vi "WVDIAL+HSRL_v5.1.vi"() -> ()   [LabVIEW 2012]
uses:
  C:/Users/H2ODial/Desktop/Shared Telescope WV DIAL Code/Libraries and VIs/PowerMeterCommands.dll
  Shared Telescope WV DIAL Code/Libraries and VIs/PowerMeterCommands.dll
  <vilib>/DAQmx/write.llb/DAQmx Write (Digital 1D Bool NChan 1Samp 1Line).vi
  <vilib>/DAQmx/miscellaneous.llb/DAQmx Fill In Error Info.vi
  <vilib>/Analysis/baseanly.llb/Mean (DBL).vi
  NCAR_DIAL_Labview/AMCS_Data.vi
  Shared Telescope WV DIAL Code/Libraries and VIs/Scalar_Data.vi
  <vilib>/Analysis/NI_AALBase.lvlib
  Shared Telescope WV DIAL Code/Libraries and VIs/Scalar_Data_2.vi
  Shared Telescope WV DIAL Code/Libraries and VIs/Scalar_Data_4.vi
  Shared Telescope WV DIAL Code/Libraries and VIs/Scalar_Data_3.vi
  Shared Telescope WV DIAL Code/bristol/CLDevIFace.dll
panel:
  out "sigma_off_total":dbl[](array[numeric])=[4.801394588286161e-25, 4.768950050217253e-25, 4.736689753639405e-25, 4.704613337303019e-25, 4.672720432926519e-25, 4.641010665257011e-25, 4.609483652155645e-25, 4.578139004644591e-25, 4.546976326993031e-25, 4.515995216769696e-25, 4.485195264899329e-25, 4.454576055746445e-25, 4.424137167181121e-25, 4.393878170609112e-25, 4.36379863107592e-25, 4.33389810729471e-25, 4.304176151739443e-25, 4.274632310672864e-25, 4.245266124220741e-25, 4.216077126439569e-25, 4.1870648453569715e-25, 4.158228803020544e-25, 4.1295685155887294e-25, 4.101083493348861e-25, 4.0727732407759397e-25, 4.044637256610407e-25, 4.016675033855836e-25, 3.9888860598986357e-25, 3.961269816478675e-25, 3.933825779804876e-25, 3.9065534205464125e-25, 3.879452203900322e-25, 3.852521589644783e-25, 3.8257610321550862e-25, 3.7991699804548973e-25, 3.772747878252632e-25, 3.7464941639826676e-25, 3.7204082708226036e-25, 3.6944896267636864e-25, 3.6687376545860182e-25, 3.643151771951297e-25, 3.617731391374568e-25, 3.592475920295502e-25, 3.5673847610815624e-25, 3.5424573110509713e-25, 3.51769296250307e-25, 3.4930911027336777e-25, 3.4686511140682367e-25, 3.4443723738419093e-25, 3.420254254472963e-25, 3.396296123410816e-25, 3.3724973432070024e-25, 3.348857271482379e-25, 3.3253752609613435e-25, 3.302050659473697e-25, 3.278882809942613e-25, 3.2558710504094295e-25, 3.2330147140280016e-25, 3.2103131290665886e-25, 3.1877656188850774e-25, 3.1653715019639748e-25, 3.1431300918716313e-25, 3.1210406972649136e-25, 3.099102621887104e-25, 3.077315164535497e-25, 3.055677619063733e-25, 3.0341892743640323e-25, 3.0128494143392254e-25, 2.9916573178829195e-25, 2.9706122588715016e-25, 2.949713506116264e-25, 2.928960323357407e-25, 2.9083519692181943e-25, 2.8878876971857424e-25, 2.8675667555590972e-25, 2.8473883874352263e-25, 2.82735183065705e-25, 2.807456317775674e-25, 2.78770107600355e-25, 2.768085327176829e-25, 2.7486082876930466e-25, 2.7292691684857373e-25, 2.710067174953994e-25, 2.69100150690391e-25, 2.6720713585077757e-25, 2.6532759182425502e-25, 2.6346143688111433e-25, 2.616085887119142e-25, 2.5976896441660036e-25, 2.5794248050002976e-25, 2.5612905286688828e-25, 2.543285968121087e-25, 2.5254102701448346e-25, 2.5076625753044143e-25, 2.4900420178674013e-25, 2.472547725712684e-25, 2.455178820294026e-25, 2.437934416518099e-25, 2.4208136227195425e-25, 2.4038155405432917e-25, 2.386939264904309e-25, 2.3701838838914442e-25, 2.3535484787249933e-25, 2.3370321236430464e-25, 2.320633885866848e-25, 2.304352825543552e-25, 2.288187995634922e-25, 2.2721384419102023e-25, 2.256203202865053e-25, 2.2403813096701963e-25, 2.224671786131482e-25, 2.2090736486310434e-25, 2.1935859061206393e-25, 2.1782075600723924e-25, 2.162937604472023e-25, 2.147775025765241e-25, 2.1327188029253344e-25, 2.1177679073943044e-25, 2.1029213031283628e-25, 2.088177946592786e-25, 2.073536786873868e-25, 2.058996765626047e-25, 2.044556817235209e-25, 2.0302158688396276e-25, 2.015972840423812e-25, 2.0018266449704104e-25, 1.9877761885463494e-25, 1.973820370468632e-25, 1.9599580834763557e-25, 1.9461882138944004e-25, 1.9325096418746903e-25, 1.918921241569432e-25, 1.905421881443037e-25, 1.892010424507014e-25, 1.8786857286323568e-25, 1.8654466468810693e-25, 1.8522920278453332e-25, 1.8392207160043708e-25, 1.826231552176911e-25, 1.813323373944262e-25, 1.800495016075253e-25, 1.7877453110235048e-25, 1.7750730895249978e-25, 1.7624771810553433e-25, 1.7499564144345078e-25, 1.7375096184837848e-25, 1.7251356226542884e-25, 1.7128332576430962e-25, 1.700601356212511e-25, 1.6884387538163331e-25, 1.6763442894316712e-25, 1.6643168063629809e-25, 1.6523551530533992e-25, 1.6404581839097108e-25, 1.6286247602390061e-25, 1.6168537512090233e-25, 1.605144034614135e-25, 1.5934944980685089e-25, 1.5819040397930432e-25, 1.5703715697926553e-25, 1.5588960107181738e-25, 1.5474762991142214e-25, 1.5361113863299152e-25, 1.5248002396306513e-25, 1.5135418433697008e-25, 1.50233520001562e-25, 1.4911793312712513e-25, 1.480073279180435e-25, 1.4690161073176908e-25, 1.4580069018064647e-25, 1.447044772476486e-25, 1.4361288539606514e-25, 1.4252583067416848e-25, 1.4144323182887283e-25, 1.4036501040910553e-25, 1.3929109086478254e-25, 1.3822140065101003e-25, 1.3715587032647203e-25, 1.3609443364486227e-25, 1.3503702764541747e-25, 1.3398359274152155e-25, 1.329340728030297e-25, 1.3188841522272228e-25, 1.3084657100845003e-25, 1.2980849483220153e-25, 1.2877414509217843e-25, 1.2774348397529735e-25, 1.2671647750218706e-25, 1.2569309555783823e-25, 1.2467331194344784e-25, 1.2365710438524509e-25, 1.226444545632135e-25, 1.2163534812596623e-25, 1.2062977468041493e-25, 1.196277278032819e-25, 1.1862920501492717e-25, 1.1763420776665477e-25, 1.1664274140569122e-25, 1.1565481514090832e-25, 1.146704420038681e-25, 1.136896387746299e-25, 1.1271242593980075e-25, 1.1173882761421185e-25, 1.107688714604918e-25, 1.0980258860269755e-25, 1.0884001353764384e-25, 1.078811840315363e-25, 1.0692614100744287e-25, 1.0597492844191873e-25, 1.050275932281712e-25, 1.040841850623073e-25, 1.0314475630412393e-25, 1.0220936184080334e-25, 1.0127805894236583e-25, 1.0035090711634834e-25, 9.942796795457985e-26, 9.85093049826673e-26, 9.759498349455631e-26, 9.668507040548591e-26, 9.577963407225883e-26, 9.487874414542166e-26, 9.398247139650076e-26, 9.309088755804386e-26, 9.220406515296338e-26, 9.132207733747452e-26, 9.044499773262688e-26, 8.957290026345629e-26, 8.870585900482974e-26, 8.784394801646169e-26, 8.698724119587757e-26, 8.613581212497107e-26, 8.528973392272335e-26, 8.444907910479177e-26, 8.361391944296957e-26, 8.278432583478717e-26, 8.196036817304802e-26, 8.114211522534205e-26, 8.032963451681958e-26, 7.952299221933221e-26, 7.872225304713498e-26, 7.792748015992029e-26, 7.713873506910441e-26, 7.635607755587433e-26, 7.557956559150637e-26, 7.480925526823318e-26, 7.40452007331766e-26, 7.328745413088994e-26, 7.253606555846716e-26, 7.179108301816113e-26, 7.105255237909276e-26, 7.032051735602558e-26, 6.959501948332896e-26, 6.887609809279164e-26, 6.816379032159524e-26, 6.745813109633723e-26, 6.675915313529315e-26, 6.606688697494169e-26, 6.538136097430423e-26, 6.47026013369233e-26, 6.403063215180626e-26, 6.336547541226546e-26, 6.270715106859048e-26, 6.20556770626669e-26, 6.141106938516726e-26, 6.077334213535519e-26, 6.014250756428306e-26, 5.951857615555011e-26, 5.890155669044941e-26, 5.829145630606328e-26, 5.768828060635133e-26, 5.709203369799531e-26, 5.650271830406457e-26, 5.592033586495535e-26, 5.534488657823541e-26, 5.477636955007899e-26, 5.421478286457689e-26, 5.366012367016147e-26, 5.311238832156924e-26, 5.257157245373203e-26, 5.203767111080975e-26, 5.151067883628761e-26, 5.099058981646601e-26, 5.047739796747887e-26, 4.99710970692362e-26, 4.9471680904655766e-26, 4.897914334302848e-26, 4.8493478509221053e-26, 4.8014680897944407e-26, 4.754274547829409e-26, 4.707766789526016e-26, 4.661944455372514e-26, 4.616807276932442e-26, 4.5723550945439755e-26, 4.52858787046509e-26, 4.485505703210599e-26, 4.443108844474691e-26, 4.401397715518555e-26, 4.360372926484654e-26, 4.320035290481737e-26, 4.2803858415410786e-26, 4.2414258571215696e-26, 4.2031568752669364e-26, 4.1655807122192707e-26, 4.1286994901985047e-26, 4.0925156557589725e-26, 4.057032001511829e-26, 4.022251691740667e-26, 3.988178290967981e-26, 3.954815788073776e-26, 3.9221686230680586e-26, 3.8902417233706774e-26, 3.859040524446151e-26, 3.828571019686779e-26, 3.7988397781509877e-26, 3.769854001153642e-26, 3.7416215439626103e-26, 3.7141509747308686e-26, 3.687451613900974e-26, 3.6615335855838153e-26, 3.63640786278229e-26, 3.612086341870923e-26, 3.5885818841799324e-26, 3.5659083977640876e-26, 3.544080898134836e-26, 3.5231155864237455e-26, 3.5030299361038637e-26, 3.4838427775418294e-26, 3.465574396234356e-26, 3.4482466342706975e-26, 3.4318830100156596e-26, 3.4165088275400604e-26, 3.402151318089598e-26, 3.388839783242867e-26, 3.3766057389929274e-26, 3.36548309398701e-26, 3.3555083377338027e-26, 3.346720715137672e-26, 3.3391624601031894e-26, 3.3328790250155764e-26, 3.3279193257884915e-26, 3.324336013175799e-26, 3.322185772847288e-26, 3.3215296392257455e-26, 3.3224333404110883e-26, 3.3249676503872935e-26, 3.329208802997051e-26, 3.335238896228958e-26, 3.343146339557761e-26, 3.353026321412742e-26, 3.364981297192093e-26, 3.379121497286846e-26, 3.395565434610739e-26, 3.414440403258726e-26, 3.4358829907497297e-26, 3.460039513028062e-26, 3.487066380487166e-26, 3.51713038203815e-26, 3.55040877164833e-26, 3.587089122589996e-26, 3.6273688416960675e-26, 3.6714542267064066e-26, 3.7195588478670957e-26, 3.7719011171675543e-26, 3.8287006590553707e-26, 3.890173237259351e-26, 3.95652358320561e-26, 4.02793573539223e-26, 4.1045600378726224e-26, 4.186495854869218e-26, 4.2737690452423645e-26, 4.3663028300744097e-26, 4.4638807992990383e-26, 4.5661005992560553e-26, 4.6723172620936825e-26, 4.781575526222953e-26, 4.8925318931385875e-26, 5.0033690286108284e-26, 5.1117084461502723e-26, 5.214532077700266e-26, 5.308129043822377e-26, 5.388090789277132e-26, 5.44938332756638e-26, 5.486527227774992e-26, 5.493910002738325e-26, 5.466237631938079e-26, 5.399100135383679e-26, 5.289584428918705e-26, 5.1368276864546713e-26, 4.9423845443889993e-26, 4.710298039802831e-26, 4.446823095455392e-26, 4.1598358649719716e-26, 3.85804282785832e-26, 3.5501475783679474e-26, 3.2441260709634926e-26, 2.946712395982361e-26, 2.6631308337930007e-26, 2.3970517538376977e-26, 2.150714060589855e-26, 1.9251465674211592e-26, 1.720428679383541e-26, 1.53594676712807e-26, 1.3706206451822994e-26, 1.2230884236655608e-26, 1.0918482976983566e-26, 9.753612237371755e-27, 8.721210233721729e-27, 7.806991018507e-27, 6.997701798420481e-27, 6.2812456801226914e-27, 5.646712358776296e-27, 5.084349444566265e-27, 4.5854974957865986e-27, 4.142505607433107e-27, 3.748638403172051e-27, 3.397981811656704e-27, 3.085352100165531e-27, 2.8062108305879284e-27, 2.5565869422707086e-27, 2.3330065259403903e-27, 2.1324302344192426e-27, 1.9521978729601313e-27, 1.789979757382958e-27, 1.643734082137034e-27, 1.5116697902511733e-27, 1.3922142210516644e-27, 1.2839850124507306e-27, 1.1857657103866845e-27, 1.096484610302639e-27, 1.015196395714895e-27, 9.410662182426697e-28, 8.733558712047939e-28, 8.114117898619021e-28, 7.546546232319497e-28, 7.025701642912456e-28, 6.547014513806149e-28, 6.106418931238552e-28, 5.700292622253593e-28, 5.325404588349162e-28, 4.9788692660923625e-28, 4.658106430581142e-28, 4.360806068197592e-28, 4.08489753956538e-28, 3.828522501146923e-28, 3.5900111064396606e-28, 3.3678610372110053e-28, 3.1607190332545146e-28, 2.967364589362001e-28, 2.7866955609085765e-28, 2.617715425159856e-28, 2.459522015206387e-28, 2.31129753123374e-28, 2.1722996779390465e-28, 2.041853801540389e-28, 1.9193458968197297e-28, 1.8042163895501554e-28, 1.6959545965331195e-28, 1.5940937941231567e-28, 1.498206814409963e-28, 1.4079021188262282e-28, 1.322820287603016e-28, 1.2426308841814503e-28, 1.1670296471282332e-28, 1.095735979222345e-28, 1.028490696002857e-28, 9.650540091750711e-29, 9.052037168469339e-29, 8.487335801198675e-29, 7.954518653327039e-29, 7.451800341677787e-29, 6.977515667544699e-29, 6.530109029807567e-29, 6.108124904915991e-29, 5.710199275226091e-29, 5.335051912802774e-29, 4.981479429414531e-29, 4.6483490131613607e-29, 4.334592782554835e-29, 4.039202695474115e-29, 3.7612259553878387e-29, 3.4997608663220985e-29, 3.253953089846661e-29, 3.0229922636158786e-29, 2.806108945951869e-29, 2.602571852405365e-29, 2.41168535589881e-29, 2.2327872228526563e-29, 2.065246562048159e-29, 1.9084619645126237e-29, 1.761859814754614e-29, 1.624892755927198e-29, 1.4970382931010645e-29, 1.3777975202772093e-29, 1.2666939582553547e-29, 1.1632724915852204e-29, 1.0670983941271466e-29, 9.777564337076934e-30, 8.948500471556312e-30, 8.180005779879964e-30, 7.468465697390879e-30, 6.810431085231261e-30, 6.202612091610602e-30, 5.641872396741644e-30, 5.12522379523866e-30, 4.6498210741493256e-30, 4.2129571491792276e-30, 3.812058425696018e-30, 3.444680354488451e-30, 3.108503155773409e-30, 2.8013276878747435e-30, 2.5210714397788027e-30, 2.2657646294144864e-30, 2.033546391805329e-30, 1.8226610435053844e-30, 1.6314544116870018e-30, 1.4583702181671436e-30, 1.301946510394041e-30, 1.160812132981031e-30, 1.0336832348936875e-30, 9.19359808752369e-31, 8.167222599729037e-31, 7.247280046352818e-31, 6.42408096031317e-31, 5.688638808252746e-31, 5.032636866339413e-31, 4.448395436382558e-31, 3.928839435526092e-31, 3.4674663990238277e-31, 3.058314941188273e-31, 2.6959337244037458e-31, 2.3753509904461953e-31, 2.0920447127862125e-31, 1.8419134350394772e-31, 1.6212478764982733e-31, 1.4267034433980083e-31, 1.255274084032685e-31, 1.1042704425817586e-31, 9.713732882503646e-32, 8.542234365126433e-32, 7.509010926979831e-32, 6.599724118567433e-32, 5.798258327626743e-32, 5.0914513032109e-32, 4.4677742840358584e-32, 3.9171311676341143e-32, 3.430696615097442e-32, 3.000769114943473e-32, 2.620636555271221e-32, 2.2844537200985846e-32, 1.9871313368209626e-32, 1.724236277148701e-32, 1.491902447124409e-32, 1.2867518305554977e-32, 1.1058250844486695e-32, 9.465210287068717e-33]
  out "sigma_on_total":dbl[](array[numeric])=[1.4915279728419454e-23, 1.4842365731966544e-23, 1.4769019163032043e-23, 1.4695253757788467e-23, 1.462108321716903e-23, 1.4546521199986097e-23, 1.447158131870194e-23, 1.439627713335683e-23, 1.432062214702501e-23, 1.4244629800835914e-23, 1.416831346884805e-23, 1.4091686453334493e-23, 1.401476198047694e-23, 1.3937553195090692e-23, 1.3860073157963141e-23, 1.378233483947944e-23, 1.370435111777655e-23, 1.3626134773198228e-23, 1.3547698485081338e-23, 1.3469054828400842e-23, 1.3390216270010062e-23, 1.3311195164756476e-23, 1.3232003753881505e-23, 1.315265415980152e-23, 1.3073158384514339e-23, 1.2993528307058406e-23, 1.2913775679522576e-23, 1.2833912126101407e-23, 1.2753949138594952e-23, 1.2673898077025441e-23, 1.2593770164365874e-23, 1.2513576486882712e-23, 1.2433327991214158e-23, 1.2353035482876853e-23, 1.2272709624381212e-23, 1.2192360933728872e-23, 1.2111999783785617e-23, 1.2031636399495558e-23, 1.1951280858745917e-23, 1.1870943088820745e-23, 1.179063286847115e-23, 1.1710359823865174e-23, 1.1630133430362646e-23, 1.1549963011158184e-23, 1.1469857736050211e-23, 1.1389826621774752e-23, 1.1309878531936014e-23, 1.1230022176071374e-23, 1.1150266109305435e-23, 1.1070618733984849e-23, 1.0991088297833858e-23, 1.0911682894818458e-23, 1.0832410465605054e-23, 1.075327879786099e-23, 1.0674295526174507e-23, 1.0595468132519867e-23, 1.0516803947245639e-23, 1.0438310149891488e-23, 1.0359993768724897e-23, 1.028186168237809e-23, 1.0203920620632735e-23, 1.0126177164388007e-23, 1.004863774789339e-23, 9.971308658609087e-24, 9.894196038876879e-24, 9.817305886336727e-24, 9.740644055897453e-24, 9.66421625982583e-24, 9.588028070218673e-24, 9.512084918974381e-24, 9.436392099708197e-24, 9.360954769268839e-24, 9.285777948467669e-24, 9.210866524075807e-24, 9.136225249623787e-24, 9.061858747248887e-24, 8.987771509156659e-24, 8.913967899106149e-24, 8.840452153334211e-24, 8.767228383070224e-24, 8.694300575302228e-24, 8.621672594735212e-24, 8.54934818499285e-24, 8.477330970786176e-24, 8.405624458768497e-24, 8.334232040093874e-24, 8.26315699129617e-24, 8.19240247593568e-24, 8.121971546612565e-24, 8.051867146610725e-24, 7.982092111191124e-24, 7.91264916943216e-24, 7.8435409460626e-24, 7.774769962767551e-24, 7.706338640024972e-24, 7.638249298761754e-24, 7.570504162344009e-24, 7.503105357207897e-24, 7.436054915859422e-24, 7.369354777003414e-24, 7.303006789004784e-24, 7.237012709367644e-24, 7.171374208324226e-24, 7.106092869293601e-24, 7.041170190650204e-24, 6.97660758762949e-24, 6.912406393431767e-24, 6.848567861106454e-24, 6.785093165255731e-24, 6.721983403264505e-24, 6.659239596832755e-24, 6.596862693493495e-24, 6.534853568410539e-24, 6.473213025417807e-24, 6.411941798788716e-24, 6.3510405548309414e-24, 6.290509892750529e-24, 6.230350346372108e-24, 6.170562386105167e-24, 6.111146419211091e-24, 6.052102792160526e-24, 5.9934317915687354e-24, 5.9351336452706864e-24, 5.877208524321972e-24, 5.8196565437619854e-24, 5.76247776404035e-24, 5.705672192417565e-24, 5.64923978370303e-24, 5.5931804425196404e-24, 5.5374940234905e-24, 5.4821803327048984e-24, 5.427239129518993e-24, 5.372670126602239e-24, 5.318472992194707e-24, 5.2646473503769066e-24, 5.211192782785618e-24, 5.158108829459499e-24, 5.10539498956517e-24, 5.053050723041136e-24, 5.001075451509333e-24, 4.949468558840217e-24, 4.8982293926143675e-24, 4.8473572651000655e-24, 4.796851453670154e-24, 4.746711202525307e-24, 4.6969357232888325e-24, 4.647524195499162e-24, 4.598475768361955e-24, 4.549789560679955e-24, 4.501464662660979e-24, 4.453500135934965e-24, 4.4058950150043495e-24, 4.3586483075526205e-24, 4.311758995648534e-24, 4.2652260364250495e-24, 4.219048362653655e-24, 4.173224883693688e-24, 4.127754486132952e-24, 4.0826360346046016e-24, 4.0378683722163014e-24, 3.9934503217979535e-24, 3.9493806859339985e-24, 3.9056582480862345e-24, 3.862281772971552e-24, 3.819250007463403e-24, 3.7765616807759944e-24, 3.734215505595965e-24, 3.6922101783280385e-24, 3.650544379764647e-24, 3.609216775654606e-24, 3.5682260172589774e-24, 3.527570741894083e-24, 3.4872495734622375e-24, 3.447261123048104e-24, 3.407603989033656e-24, 3.368276758374866e-24, 3.3292780061505364e-24, 3.290606296806844e-24, 3.2522601840825837e-24, 3.2142382118355154e-24, 3.176538914110844e-24, 3.1391608160083538e-24, 3.1021024337339513e-24, 3.0653622750140015e-24, 3.0289388399119578e-24, 2.9928306205862763e-24, 2.957036102223797e-24, 2.921553762996284e-24, 2.886382074756912e-24, 2.8515195030565572e-24, 2.8169645078141113e-24, 2.782715543322614e-24, 2.748771058894172e-24, 2.71512949885664e-24, 2.6817893031738804e-24, 2.6487489074336617e-24, 2.6160067433846084e-24, 2.5835612389782294e-24, 2.5514108189999835e-24, 2.51955390492328e-24, 2.4879889154638994e-24, 2.456714266715629e-24, 2.4257283723422857e-24, 2.3950296439844203e-24, 2.3646164913248486e-24, 2.3344873224248166e-24, 2.3046405438364146e-24, 2.2750745608716746e-24, 2.2457877779121212e-24, 2.216778598453289e-24, 2.1880454252542657e-24, 2.1595866608282875e-24, 2.131400707227615e-24, 2.103485966569378e-24, 2.0758408409643995e-24, 2.0484637328312535e-24, 2.021353045010762e-24, 1.994507180833902e-24, 1.9679245444152724e-24, 1.9416035408428514e-24, 1.915542576055622e-24, 1.8897400572521647e-24, 1.8641943928932106e-24, 1.8389039929188542e-24, 1.813867268749188e-24, 1.7890826334938338e-24, 1.7645485021106223e-24, 1.7402632913600035e-24, 1.7162254201577694e-24, 1.6924333094442993e-24, 1.66888538241001e-24, 1.6455800646330604e-24, 1.6225157840636093e-24, 1.5996909711590041e-24, 1.5771040590484899e-24, 1.5547534835828714e-24, 1.5326376832802828e-24, 1.510755099657201e-24, 1.4891041771310975e-24, 1.4676833631346243e-24, 1.44649110822398e-24, 1.4255258660850895e-24, 1.4047860937336335e-24, 1.3842702513880348e-24, 1.3639768026964584e-24, 1.3439042147649745e-24, 1.324050958126476e-24, 1.304415506922052e-24, 1.284996338865958e-24, 1.2657919353597275e-24, 1.2468007815143876e-24, 1.228021366173415e-24, 1.2094521820183057e-24, 1.1910917255865317e-24, 1.1729384973433326e-24, 1.1549910016186627e-24, 1.1372477468095316e-24, 1.1197072453129342e-24, 1.1023680135666647e-24, 1.0852285721375928e-24, 1.0682874457072983e-24, 1.0515431631559607e-24, 1.0349942575468164e-24, 1.0186392661829782e-24, 1.002476730637983e-24, 9.865051967629649e-25, 9.707232147605914e-25, 9.551293391457332e-25, 9.39722128860001e-25, 9.245001471889606e-25, 9.094619619146324e-25, 8.946061452123616e-25, 8.799312737179386e-25, 8.65435928609183e-25, 8.51118695565651e-25, 8.369781647900126e-25, 8.230129310101864e-25, 8.092215935920228e-25, 7.956027564445635e-25, 7.821550280769177e-25, 7.688770216681373e-25, 7.557673549946735e-25, 7.428246505170648e-25, 7.30047535360111e-25, 7.174346412961231e-25, 7.04984604874062e-25, 6.926960672865143e-25, 6.8056767449681615e-25, 6.685980771732338e-25, 6.567859307790466e-25, 6.451298955087012e-25, 6.336286363602155e-25, 6.222808230746433e-25, 6.110851302620752e-25, 6.000402372716947e-25, 5.891448283289271e-25, 5.7839759247643095e-25, 5.677972235862969e-25, 5.573424204095667e-25, 5.470318865351133e-25, 5.368643304265269e-25, 5.268384654678351e-25, 5.16953009900346e-25, 5.072066868702154e-25, 4.975982244718514e-25, 4.881263556774869e-25, 4.787898184158063e-25, 4.695873555477195e-25, 4.605177149080389e-25, 4.515796492621548e-25, 4.42771916358447e-25, 4.340932789269877e-25, 4.255425046890637e-25, 4.171183663666919e-25, 4.0881964166458944e-25, 4.006451133456628e-25, 3.925935691662753e-25, 3.8466380195018056e-25, 3.768546095362677e-25, 3.6916479484173746e-25, 3.6159316584590197e-25, 3.541385356169944e-25, 3.467997222902915e-25, 3.3957554911138307e-25, 3.3246484443824274e-25, 3.254664417370916e-25, 3.1857917961611124e-25, 3.1180190182139765e-25, 3.051334572486769e-25, 2.985726999551206e-25, 2.9211848919101016e-25, 2.857696893775905e-25, 2.7952517013337095e-25, 2.733838062926984e-25, 2.6734447792968603e-25, 2.6140607032789457e-25, 2.5556747403616704e-25, 2.498275848573554e-25, 2.441853038787586e-25, 2.3863953746296823e-25, 2.3318919728376534e-25, 2.278332003183737e-25, 2.225704688927324e-25, 2.1739993065442936e-25, 2.1232051862289785e-25, 2.0733117118382346e-25, 2.0243083210918132e-25, 1.976184505768082e-25, 1.9289298117223313e-25, 1.8825338392641452e-25, 1.8369862430522042e-25, 1.7922767325107508e-25, 1.7483950717412174e-25, 1.7053310799305548e-25, 1.6630746313165588e-25, 1.621615655402141e-25, 1.580944137272083e-25, 1.5410501175792854e-25, 1.5019236927958814e-25, 1.4635550153571604e-25, 1.4259342939087199e-25, 1.3890517934829874e-25, 1.3528978355570778e-25, 1.3174627983975394e-25, 1.2827371171531552e-25, 1.2487112840480117e-25, 1.2153758486306102e-25, 1.1827214179365787e-25, 1.1507386566320074e-25, 1.1194182872674774e-25, 1.0887510905251834e-25, 1.058727905293928e-25, 1.029339628950446e-25, 1.0005772175855101e-25, 9.72431686140841e-26, 9.44894108685872e-26, 9.179556185822558e-26, 8.916074086770922e-26, 8.658407316171975e-26, 8.406468999218454e-26, 8.160172863179967e-26, 7.919433238617652e-26, 7.684165062493321e-26, 7.454283879629295e-26, 7.229705845113006e-26, 7.010347726836595e-26, 6.796126907225739e-26, 6.586961385949759e-26, 6.38276978141041e-26, 6.18347133417278e-26, 5.988985907910388e-26, 5.799233992536743e-26, 5.614136706431352e-26, 5.43361579806481e-26, 5.25759364915564e-26, 5.0859932759575334e-26, 4.918738332379802e-26, 4.755753111884154e-26, 4.5969625496531854e-26, 4.442292225171654e-26, 4.291668364069986e-26, 4.1450178406905347e-26, 4.002268180317973e-26, 3.863347561315701e-26, 3.7281848171048934e-26, 3.5967094390677064e-26, 3.468851577979995e-26, 3.344542046705501e-26, 3.223712322196132e-26, 3.106294547577355e-26, 2.992221534363318e-26, 2.8814267646988245e-26, 2.77384439311716e-26, 2.669409248940071e-26, 2.5680568381228437e-26, 2.4697233453325032e-26, 2.3743456359824082e-26, 2.281861258018756e-26, 2.1922084440028567e-26, 2.105326112933142e-26, 2.021153872040787e-26, 1.9396320185987354e-26, 1.8607015418529674e-26, 1.7843041244697932e-26, 1.7103821443779257e-26, 1.6388786762649565e-26, 1.5697374932592083e-26, 1.5029030684283447e-26, 1.4383205761250682e-26, 1.3759358934207283e-26, 1.315695601525129e-26, 1.2575469868929259e-26, 1.2014380425673393e-26, 1.147317469184652e-26, 1.095134676079673e-26, 1.0448397822754321e-26, 9.963836172753061e-27, 9.4971772196569e-27, 9.04794349305064e-27, 8.615664649294304e-27, 8.199877476875684e-27, 7.800125900786263e-27, 7.41596098654387e-27, 7.046940940939089e-27, 6.69263111496513e-27, 6.352604002895075e-27, 6.026439241289035e-27, 5.7137236071845856e-27, 5.414051014326314e-27, 5.127022508554483e-27, 4.852246261413911e-27, 4.58933756343785e-27, 4.337918814680109e-27, 4.097619514659347e-27, 3.868076251135339e-27, 3.648932686256661e-27, 3.439839542349354e-27, 3.240454585084498e-27, 3.0504426059763557e-27, 2.8694754024787748e-27, 2.697231756497351e-27, 2.533397411574622e-27, 2.3776650476361677e-27, 2.229734254391782e-27, 2.089311502695099e-27, 1.9561101136589846e-27, 1.8298502264715367e-27, 1.7102587635784418e-27, 1.597069394077526e-27, 1.490022495057276e-27, 1.388865110858837e-27, 1.2933509098837144e-27, 1.203240139522051e-27, 1.1182995788130716e-27, 1.0383024886079031e-27, 9.630285597373842e-28, 8.922638586327791e-28, 8.25800770799641e-28, 7.634379416762275e-28, 7.049802153718404e-28, 6.502385707805079e-28, 5.990300553614198e-28, 5.511777164565142e-28, 5.065105301666708e-28, 4.6486332770176045e-28, 4.260767194248587e-28, 3.8999701624520967e-28, 3.5647614867305684e-28, 3.2537158343332264e-28, 2.965462375694583e-28, 2.698683902202115e-28, 2.4521159197164444e-28, 2.224545718662294e-28, 2.0148114208971141e-28, 1.8218010041295442e-28, 1.644451303999103e-28, 1.481746994271063e-28, 1.3327195466405238e-28, 1.196446169846401e-28, 1.0720487294456503e-28, 9.586926490362017e-29, 8.55585793950267e-29, 7.619773383069837e-29, 6.77156616513607e-29, 6.004519607440531e-29, 5.312295253643437e-29, 4.688920998465674e-29, 4.128779115562369e-29, 3.6265942014961644e-29, 3.1774210502624405e-29, 2.7766324764021174e-29, 2.4199071058475946e-29, 2.1032171517063065e-29, 1.8228161961805425e-29, 1.5752269980978955e-29, 1.357229347392151e-29, 1.165847988469448e-29, 9.983406339113933e-30, 8.52186091863709e-30, 7.250725293042887e-30, 6.148858947224475e-30, 5.196985233425073e-30, 4.377579477510319e-30, 3.674759372687666e-30, 3.0741778843134e-30, 2.5629188881985504e-30, 2.129395756437773e-30, 1.7632530969735417e-30, 1.4552718422808334e-30, 1.1972778702820177e-30, 9.820543263583868e-31, 8.032577992814456e-31, 6.553384851850636e-31, 5.334644543652936e-31, 4.334501134917267e-31, 3.516889327327518e-31, 2.85090482423036e-31, 2.3102179813251066e-31, 1.8725306598992244e-31, 1.5190759294300348e-31, 1.2341599889417139e-31, 1.004745403179991e-31, 8.200744823762983e-32, 6.713313779722865e-32, 5.513412267391353e-32, 4.5430445638202427e-32, 3.755641725612538e-32, 3.1140438418044294e-32, 2.588766950196661e-32, 2.1565299891004846e-32, 1.7990166479232517e-32, 1.501846887779191e-32, 1.2537332288520025e-32, 1.0457976319433735e-32, 8.710259118374657e-33]
  out "FileHour":i32=22
  out "L_Count":i32=2014
  out "background start":u32=534
  in  "Tab Control 2":enum32{"WV ND narrow", "WV ND wide"}(tab)
  out "CH3 RingBuffer long":dbl[][](array[numeric])
  out "CH3 RingBuffer short":dbl[][](array[numeric])
  in  "?":T1(tab)=enum."Raw Counts WV offline"
  out "NRB":dbl[][](graph)=[[2.020963360170281e-05, 7.627540920388829e-05, 0.0001737203677038386, 0.00031804133708114346, 0.0005081997367790425, 0.0007554792778400287, 0.0010484291521190752, 0.0014236671746623347, 0.0018766688616627084, 0.0024211128093211674, 0.003108603837864134, 0.003914025877784729, 0.004924828296497507, 0.006081056662523466, 0.007420472218672901, 0.008849650154360648, 0.010371729184413437, 0.012315479668306428, 0.014485774002489606, 0.016805076080561115, 0.019481297865527998, 0.021782337623552018, 0.0245233110616514, 0.027333614587787998, 0.030183602307263715, 0.03352578050261507, 0.036850415772967736, 0.04072527859793505, 0.044699853731394866, 0.04892654575091603, 0.05290103345620475, 0.057070591271614055, 0.06094791096393855, 0.06495661419487804, 0.06966097196013363, 0.07443274679199274, 0.07932433134895593, 0.08293278269107832, 0.08529593272037989, 0.08628493365309849, 0.08614683735981367, 0.0895522821951441, 0.09408054635124959, 0.10001183787388598, 0.10805726515641365, 0.11220235971302907, 0.11527139909776056, 0.11731524632465085, 0.11559758869278183, 0.11288241937180105, 0.10864149774714038, 0.103759844699048, 0.10036669203501673, 0.10079345225327473, 0.10133653719142077, 0.10392011108797332, 0.10765399257016298, 0.10847639040173439, 0.1111727634355607, 0.11033102836642139, 0.11160364425162826, 0.11237201174223443, 0.11293220353502097, 0.11611470152399855, 0.11988280457515896, 0.1250182824785479, 0.1293078925043753, 0.13161491538627124, 0.1335256951432043, 0.13877781635672834, 0.14588833388403924, 0.1525162849835717, 0.15629147529686666, 0.15546951921340244, 0.15481563526094977, 0.15325369084913773, 0.15095672838537877, 0.14780066163663746, 0.1426466570792243, 0.13569619631305252, 0.12398915720169047, 0.11506725294987205, 0.10321777758317247, 0.09475089868063362, 0.09155910071015527, 0.08842753125965389, 0.08308384640818023, 0.08599724174764481, 0.08457909373021681, 0.08350939060632413, 0.08526662116351132, 0.07841811966698599, 0.07521579178540691, 0.06714558649742469, 0.06342255068533684, 0.0637050627258514, 0.06408089778095057, 0.06704969463901601, 0.0696808363958791, 0.0690587099521849, 0.07456904160810134, 0.07536933669652675, 0.07668013652465497, 0.08322232788474623, 0.08562734854276098, 0.0914376493267812, 0.10133394710158722, 0.10837240306663742, 0.12475509624148345, 0.16689793981091888, 0.23328664075032238, 0.35188808487682044, 0.5424281177090396, 0.8071927480904378, 1.2119772875984736, 1.7864080691388573, 2.601123869622575, 3.7000497375140617, 5.029243150658778, 6.542194578493981, 8.126428612546306, 9.704567759797246, 11.19301703376241, 12.458015726961536, 13.38676804260307, 13.894705494058375, 14.001451661847625, 13.839516750580922, 13.57394546500907, 13.250439970369818, 12.852273526374864, 12.35166295810407, 11.696144981925006, 10.931202915907384, 10.067595672481655, 9.103078928975787, 8.057659858480005, 6.97764665635014, 6.015345272701211, 5.278975287205386, 4.831871743689986, 4.660409912964652, 4.644444811055265, 4.7061144696068675, 4.741728200035577, 4.697784589712353, 4.5959042054612365, 4.450651241302527, 4.261398951257744, 4.050910195919229, 3.817489544303836, 3.5391131213436853, 3.2471327707683266, 2.975372528669963, 2.7267156398073373, 2.4794075581227033, 2.2273460486656664, 1.9551503161957537, 1.681024324129587, 1.4297160338094892, 1.2240862485794186, 1.037972885987915, 0.8765919728781653, 0.7308761413820998, 0.5826095867681264, 0.4708388989763128, 0.36158164533313786, 0.2833790088137393, 0.21666235218657698, 0.15638062340463046, 0.12028362008697967, 0.06960870675373829, 0.05410227103997058, 0.04031082286780983, 0.026593266101065743, 0.02303214909282192, 0.00827236726618211, 0.010031014655625252, 0.004461672806757203, 0.004937293453871461, 0.0011189613557765225, -0.018667141890600966, -0.018872838871342095, -0.009406477976568009, -0.0027650427450897283, 0.005612791374859748, 0.008659276298978927, -0.0012303973150859023, -0.0028859048034287865, -0.003627869770464881, -0.013730022858502925, -0.004673180139108649, 0.0071442043013560256, 0.0115445776691833, 0.019906170998752894, 0.023391228903177564, 0.01967930475729538, 0.010995517265275487, 0.008115537576785637, -0.008223490292534318, -0.008438612653904309, 0.007960046811788043, 0.007633039417571788, -0.0004920247046047625, -0.018576844235517226, -0.029210706571153305, -0.02555488488399655, -0.020119112459026443, -0.007402263593608766, 0.011644527320968785, -0.01134613452622009, -0.0037786349328193087, -0.011711243530276473, -0.02625968079350423, -0.011476780802441635, -0.030276888116334433, -0.02700109417602674, -0.024285158897854292, -0.015530507697806365, -0.0023207153684570575, -0.0025022619331753634, -0.011912562987963986, -0.02851488484103791, -0.022015152082293835, -0.01805572762928951, -0.00815221326567346, 0.003959976956190213, -0.0021511167155719144, -0.0025144759222573672, -0.008964532499299552, -0.02218590368617358, -0.035458762869299394, -0.030773037425800096, -0.030318462017452714, -0.02803907105532127, 0.0019023128619800737, -0.0012174877176892695, 0.0015626356358757053, 0.002513768685763893, -0.0069235112795537875, -0.014038908589074271, 0.00026926693626070427, -0.004576651815937033, -0.005005446986479409, 0.002050171099187623, -0.025756957477399346, -0.016750248538706224, -0.02637945667262903, -0.022113050246786746, 0.005829396983909488, 0.0050485003851483325, 0.003420343736463852, -0.013159434753370733, -0.03381571228294774, -0.01272766080488575, -0.003788053872003038, 0.009631082249493569, 0.016045839178541382, 0.0016302557263238831, 0.023844005674827643, 0.013960216541708901, 0.011136676238174143, 0.028032091129227214, 0.017487522576306355, 0.04137567842060789, 0.025654331272517476, 0.000796023293004166, -0.033164529559518166, -0.03959109502790817, -0.02959140387729691, -0.023540134803692603, 0.0030128961838231825, -0.019727930076879518, -0.01198284053437428, -0.00635811825370373, -0.0021514957939473703, -0.0021671145869274814, -0.029594293415964007, -0.03134140667130025, -0.033883730757818864, -0.009231781364444126, 0.028572211280513266, 0.04823955509288692, 0.02871403590065173, 0.0070423701229230615, -0.016278958837779002, -0.03397605321686615, -0.005066656134954104, 0.0014812005230668084, -0.004584876793526415, 0.001223666380830473, -0.030129931552195035, 0.008289109622824066, 0.012036114688207785, -0.016748027203555824, 0.008747467856935214, -0.021031536574595663, -0.007757778497261617, 0.010980941834970684, 0.021399715586409306, 0.01767444861275386, 0.010303809677163614, 0.00012060615500020031, 0.007709142008481225, -0.0023218662271697983, 0.025646980532729863, 0.014981252977212298, -0.002367766920443276, -0.00332388994006669, -0.0058702938677793436, 0.03570388838213545, 0.03081868105785836, 0.03326881277230231, 0.018910305438978196, 0.0053442870882247666, -0.0051159040068622505, 0.017623249679543405, 0.03234752526807859, 0.03188287890750651, 0.06134170519066627, 0.023146905690649644, 0.0059249658756949115, -0.003974539407197516, 0.018410156916276905, 0.05182593366384886, 0.04516463879368706, 0.05387047816217671, 0.011801021902527076, -0.011588637587261547, 0.0019312835928925137, -0.03080000228073684, -0.010352979069787742, -0.013693015812498746, -0.003517126713415386, 0.03921565233645448, -0.009862417922918417, 0.005370899710682564, 0.016283545331230467, 0.017134883727146246, 0.05368299764129211, 0.04407000565518596, -0.008297158021748054, -0.00564111244594224, -0.026660152863915026, -0.004534401297258525, 0.032397142809446944, 0.013207812000496193, -0.01893162368151735, -0.007440246237142469, -0.012310638417782491, 0.02282021134422728, 0.062422427276102296, 0.019397856401382287, -0.002716279279138828, -0.026323015759716115, -0.036044486835827824, -0.024109098029399333, 0.012374814449785358, 0.0014391039013826803, 0.02911306157265743, 0.009159108188869449, -0.010587063885684103, -0.011943882028404565, -0.0820656827265583, -0.044452872804326714, -0.07637119491514727, -0.07413513146238972, 0.004625445579948104, -0.009211776415148807, -0.03848559535083536, -0.05813105040942421, -0.09480179587972846, -0.09896740806181374, -0.03472852766949326, -0.021983250596292254, 0.037794391566584984, 0.054799855311378515, 0.04242087588745626, 0.053967580287972335, 0.009200127794353351, -0.04795880637436305, -0.031437811975261444, -0.03979226904188478, -0.08503634384069148, -0.021710951279749993, -0.025738461775737298, 0.03315191076055578, 0.07633799519138025, 0.0707682969939044, 0.06863494844866702, 0.03082821640020612, 0.03704206224883394, 0.04686889864022042, -0.011012085963750223, -0.023365847152530577, -0.028634347138830132, -0.03136718694634836, -0.003953699520006499, -0.0196587741828821, -0.03289396117013728, -0.028833910608738567, 0.004988896811954685, 0.05621844997698572, 0.018975425774946802, -0.011096875217535, -0.06690985801808111, -0.11946401924829003, -0.08943792088401828, -0.08108707660125468, -0.04228806538120522, 0.012426725681956973, 0.01973436839980497, 0.017029387838860283, 0.04638261125470255, 0.014932252316656498, 0.017846033193922004, 0.059621203073039544, 0.0673673206694292, 0.08268120310490894, 0.06975153907287768, 0.05611371886686261, 0.06749308044390862, 0.02609093121500152, 0.04510785208158361, -0.016372315881433223, -0.06293661229021995, -0.036286936842063265, -0.019612281739682, 0.0026594488066321955, -0.011294665308557756, -0.04246052667494757, -0.04817384365082581, -0.05024433447113321, -0.0016083365005076667, 0.0033558047554186014, -0.009114849352938284, 0.013421518647955502, -0.03188020076747843, -0.06050726934267876, 0.0021617656233865897, -0.0022993429588677155, 0.10612322997663393, 0.12529542603481097, 0.027450963778686308, -0.012096409398199824, -0.15913366627246373, -0.12900762816664782, -0.10585704118748897, -0.04144659666163028, 0.030858084086696623, 0.047027575960958, 0.08816604810853647, 0.03127089667825644, -0.03357497744665111, -0.11395010424757208, -0.11308578368860221, -0.08134612078056679, 0.009920149045176213, 0.02518560161832109, 0.0002779712489847596, -0.004606485913066665, -0.04177843649116545, 0.051675537811200316, 0.04482825224307555, 0.050702690537533714, 0.0737429422203154, 0.046842295828900815, 0.10674692783834813, 0.09275551401568609, 0.07138693168848631, 0.058576725292767265, 0.028095765630968453, 0.0693620670680278, -0.010772914176104499, -0.04342170224420895, -0.056254474572071736, -0.13644413976886144, 0.014557354563469746, 0.050034067115134355, 0.061593395038345836, 0.03601591742875882, -0.056155634356297085, -0.06175192314005483, -0.07662500798175192, -0.03522660725174814, -0.00046542314356257775, -0.012929734176502571, 0.02768652457938517, 0.03408264454281327, -0.013878047709166395, -0.038478810523569267, -0.1515200684818307, -0.15373300005585958, -0.10627146182240307, -0.10831151121493415, -0.04169032943946463, 0.02222739550862387, -0.014334907722049577, 0.054299505082943206, -0.0070609371519486765, 0.0184649663031647, -0.0054622972602069945, -0.06863365486177031, 0.01201291251053317, -0.027303815566110588, 0.01042671236106932, 0.013000541027569132, -0.031866771570098706, -0.006466556560079296, 0.08490918563657528, 0.05179707245234805, 0.16133951606185634, 0.13604092425607042, 0.03418598889027207, 0.13100628979611995, 0.06768111071870647, 0.02931926070144779, 0.07525663643219518, 0.10031739236145769, 0.026996385460592603, 0.06989058251582808, -0.013960122450387092, -0.1155217419768775, -0.03210224794422068, -0.08834642305071791, -0.07232788698569816, -0.056185446909282157, -0.10492340376044737, -0.07591236126055854, -0.029151562981127987, 0.1059359995097289, 0.2290326634989594, 0.20376963000926943, 0.10619988170605181, 0.01541616096575596, 0.01641737390748474, -0.05170867076903334, 0.07262480608035493, -0.045415793397229655, -0.11357741152513673, -0.08035666037071708, -0.14336264821290465, -0.025757547319254642, -0.08027844576743458, 0.022826217380744793, 0.03465884490689662, 0.009236917565209704, 0.036885725627331195, 0.055827749120229905, 0.09974406608053392, 0.09013619677715916, -0.003602506141673624, 0.03354456710096207, 0.037697864053219336, -0.09873163522974107, 0.0, 0.0, 0.0, 0.0, 0.0]] caption="Water Vapor Number Density"
  out "NRB 2":dbl[][](graph)=[[3.664325328762682e-05, 8.578066435905075e-05, 0.00019640091176320866, 0.00037959626807595445, 0.0006348941300169956, 0.0010215884116584445, 0.0015577066105081365, 0.002167181287015159, 0.00285868511986523, 0.003668298545758931, 0.004701471580960624, 0.006119238107290852, 0.007863432861492558, 0.010027546431010968, 0.012544665615599495, 0.015057091633429633, 0.018321199010642525, 0.021994771578991126, 0.02576613085481857, 0.029885958030703964, 0.03425297390662341, 0.038911443131181854, 0.04334736477360056, 0.04775304605122944, 0.05159548492017764, 0.0558931790813754, 0.06075683986532259, 0.06635038055893583, 0.0729387056097223, 0.0789819206715066, 0.08618887765510425, 0.09225733369277504, 0.09803757981160244, 0.10452987474653358, 0.11052100070164539, 0.11753346139397144, 0.12371740766300787, 0.12986232406282863, 0.1332572648681056, 0.13581257784585182, 0.13594266126483961, 0.13724017226734156, 0.138393214577315, 0.14471226645352597, 0.15623587260027075, 0.16291281380405623, 0.1717221504944407, 0.17319798151707771, 0.16784968448373194, 0.1618948524741329, 0.15492238732832733, 0.14903833416814286, 0.14854204141962923, 0.15098254634132516, 0.1505020673799309, 0.14816993150707145, 0.14695435588246414, 0.14738673828676546, 0.15017230940349388, 0.15631955960520136, 0.15756823190408892, 0.1515231096530448, 0.1516663535839558, 0.15638374112611497, 0.16375722622580002, 0.17306111652265244, 0.17223560435005145, 0.1672184647591005, 0.16249465423311685, 0.17007763442454282, 0.1805126492178654, 0.19030191123054985, 0.1972657308720967, 0.1970685601301737, 0.19509320214190604, 0.19444082103115096, 0.19176008516353008, 0.18023975016191435, 0.17553392953526645, 0.1589115233396072, 0.1494930505615103, 0.1404823603590125, 0.12382982374055787, 0.12407760907511578, 0.10881639010131301, 0.09561572619723971, 0.0882912079214967, 0.08382857013548725, 0.08574458988161086, 0.09697617068565112, 0.10179933566625249, 0.08843213423746735, 0.08993605790003598, 0.0775946763081636, 0.06517139451732387, 0.06868335468685989, 0.06346525520118712, 0.06598702775484523, 0.07045104113630396, 0.07102195433096696, 0.07460779155512785, 0.07746827856440726, 0.08260722223831354, 0.08657904659911396, 0.09054832969784396, 0.09551308044262664, 0.09985979319220557, 0.11234012160577972, 0.13344354734651076, 0.17615659076104, 0.2495518960496045, 0.37182616765598403, 0.5594051674782835, 0.8344407805039018, 1.2563723339361608, 1.8681848065032547, 2.737229515826324, 3.929537166422711, 5.350204222523604, 6.966061098745903, 8.66208339939891, 10.341975055100326, 11.935367463661503, 13.300662152686877, 14.267805234744909, 14.785089509845278, 14.913141856242337, 14.772494080298378, 14.543483383948129, 14.25620427152592, 13.83548322509587, 13.283062588092468, 12.606934235658315, 11.774215949749557, 10.860643703956509, 9.837362612197245, 8.682597924211157, 7.494315190194337, 6.478754925825519, 5.665308298845379, 5.191036744019726, 5.025932242202884, 5.055960440886686, 5.123865980751719, 5.174725599310386, 5.147101895525789, 4.976951201411453, 4.828893300639637, 4.612501706145317, 4.3683408098930645, 4.087032861483217, 3.7956576938103916, 3.506470079590515, 3.2180497928459344, 3.012004016358344, 2.735950746965229, 2.4516877014440337, 2.146942348131546, 1.7890684043257388, 1.4990052134210268, 1.2202517370303771, 1.0356179509160008, 0.8693406081400015, 0.7491759950971097, 0.6275305653787341, 0.5291365503854003, 0.4203155045195759, 0.2672628273301941, 0.21370409406342974, 0.12911361513084438, 0.06501317083388042, 0.02539583745573544, -0.012089949641497389, -0.05574979809012831, -0.05780916519963046, -0.02581982704940756, -0.06773021933237808, -0.04159120834983531, -0.013684271791444791, -0.02925516348583521, -0.01886348769001042, -0.02005763389694655, -0.05137487371923708, -0.042764254463579995, -0.014843225422055963, -0.07627923472508875, -0.07398188654126416, -0.08038095851011275, -0.08855621682356063, -0.047626616961437024, -0.030890685408544994, 0.0027726760745075255, -0.028340679637629283, 0.0003432702817362685, -0.04023984207539884, -0.07530845334370231, -0.05350892106831006, -0.11053324742329858, -0.08469750602153464, -0.09334889800108401, -0.0865420190820581, -0.07796731806669636, -0.09889364370634941, -0.10468314249220471, -0.12140286744331506, -0.09496750523481973, -0.08654718319151583, -0.11883524786270719, -0.11622808085934366, -0.10991152419441563, -0.0647681283309405, -0.05543312587141729, -0.04186488014360598, -0.062385788712694276, -0.07167666457274835, -0.04135656635028461, -0.00034857076676722863, 0.0023180535386341256, -0.012875930890484357, -0.015872741012524543, -0.029413379939107802, 0.005824093917938762, -0.001189793465023191, -0.025906332035571154, -0.026640032626319022, -0.10873360774857133, -0.1219570191470042, -0.09847094276556558, -0.11215933722065854, -0.071888439130888, -0.08291809814418706, -0.0886174618980101, -0.09189450627667858, -0.11186366153700103, -0.09694602193750136, -0.050105940958925704, -0.10881119085938451, -0.10898269094652316, -0.07894581910102427, -0.13860952493382891, -0.07432300053383152, -0.03372062186983823, -0.10756129355863683, -0.06910252526280258, -0.12560304205273806, -0.12543069709359272, -0.1050837398725921, -0.07992262883897083, -0.0283237504648303, -0.017192241614252236, 0.08968558348025148, 0.007084812394832199, -0.06456460842583929, -0.07147170895732163, -0.17409528374490113, -0.10725079136171854, -0.012493590602395764, -0.04404597699099435, -0.07785989144641998, -0.1358695904781577, -0.16347724775947556, -0.19966135088168044, -0.15525037660933627, -0.07007066483256019, -0.12467040267367596, -0.11836523786672688, -0.10276733515461521, -0.178296774057137, -0.14328683444796936, -0.13929559570292535, -0.08524184624135792, -0.03819862223612276, -0.06310824519101588, -0.05290360994291476, -0.0867771901391151, -0.13372494643931376, -0.1024960477509449, -0.07310257360140365, -0.07903111727571714, -0.07985773342813518, -0.051727323012341425, -0.07837479282718213, -0.11995201495362466, -0.10214487951734484, -0.12084824693539285, -0.13413084373119105, -0.17154162476973325, -0.14039856929788408, -0.13502765623358717, -0.06454280108088699, 0.07605107097219688, 0.03656242562741421, 0.07766746508933023, -0.01949192189510563, -0.05701004654385092, -0.04726366598125846, -0.0467090833412978, -0.0458503250575347, -0.10583431075323613, -0.12498203422581738, -0.26472400202253593, -0.16794175535117126, -0.11050519636985778, -0.13016937979279103, -0.037577853099010815, -0.004715750340805577, -0.09070690238999544, 0.0018057087155675252, 0.06587121748154647, -0.07692786129636506, -0.038112005554471654, -0.07342025498393201, -0.15773816035770707, -0.10042924853418898, -0.1784491875894576, -0.20301076016150366, -0.08874286727345129, -0.13040518138049073, -0.04245190125162826, -0.045763957355803006, -0.19348351555802645, -0.11657564464071989, -0.0866179503313669, -0.0757076372853694, -0.08490164248101639, -0.012025169966696931, -0.08524310802003922, -0.026394072637770452, 0.01922988319657702, -0.05334715318203209, -0.047878153735040195, -0.1268426281926552, -0.08839999443774964, -0.1471754814889216, -0.1562164888162528, -0.11797961509431791, -0.14833011319894504, -0.15713938759572277, -0.011484275480767954, -0.034854850611195115, -0.11498486107226094, -0.14542080053472647, -0.3161548322647022, -0.2096908128432946, -0.2435551794643545, -0.1436996494552559, -0.03590692288322063, -0.20979368319600922, -0.14217752561858113, -0.15878033650435738, -0.30298609558038825, -0.2830164293681652, -0.19527796719014534, -0.2377945198957981, -0.17209450960779715, -0.11820380644599332, -0.13613596833764807, -0.06532520870301776, -0.00691668295614864, -0.0510676680334108, -0.12714579811304888, -0.2430346098985066, -0.3432144120723012, -0.2820653162396176, -0.2682098316761112, -0.2382546451872164, -0.1420891565303358, -0.19745921770926092, -0.08289975756851237, -0.048063020318079824, -0.18067969664435302, -0.17296674487447297, -0.23780106525275038, -0.2663473667355993, -0.1093171708713277, -0.0468313333592609, -0.050838175619409245, -0.134681150257329, -0.1866572308965044, -0.24490173939278867, -0.33253008886489027, -0.13802882809134132, -0.11306165376573979, -0.05761637958478377, 0.03172154305292979, -0.04541653329409793, -0.14908939562556683, -0.2224901363967072, -0.34564121504083917, -0.4087340307819123, -0.26332684088350494, -0.2352254213301905, -0.22826136595503657, -0.2227560113188565, -0.3733987945226789, -0.4110442575158397, -0.34073516993063213, -0.09487175055393855, 0.020917858882750794, -0.008058012458123901, 0.0700165757429996, -0.07115497316786143, 0.03153680251782819, 0.15790980024844817, 0.1641132084348499, 0.24391461855724683, 0.12960735583891575, 0.10163863337027003, 0.0838944487804799, 0.1720791715301368, 0.05903813637156058, 0.08905638817606407, -0.016481621174385598, -0.22159130712211367, -0.16063036994351407, -0.22259376100315034, -0.28112479633627757, -0.29228966901783576, -0.3076125648916034, -0.2805211995660978, -0.3017712541935481, -0.31144483911618875, -0.43412481419281473, -0.43023965187700125, -0.20188944486026972, -0.27420142595684477, 0.013713629991017853, -0.028596916247378035, -0.039069805678392376, 0.19294321396540667, 0.17972185572463478, 0.18549084828814674, 0.07048443651756973, -0.11343311135747812, -0.29841516560985804, -0.2972761821112056, -0.3409202288340118, -0.5320179271800709, -0.4987901681996697, -0.4780362261568327, -0.32662572761079006, -0.1002226475223006, -0.0753845288233559, -0.08354263466865222, -0.18861965545636977, -0.19998531287066043, -0.17117125317718318, -0.2992747934838438, -0.12807157220413126, -0.21496416832975196, 0.08587690253315688, 0.2037386837128645, 0.16055995438757897, 0.13266073109192197, -0.2054014796174304, -0.1932500945387914, -0.14164792482204105, 0.16204421903549737, 0.2511776151464063, 0.31800844569434256, 0.2828700402765013, 0.016053902779057747, -0.14184982936095286, -0.4497981002191686, -0.6274939130073838, -0.5677717117379886, -0.5759759546968973, -0.43877003703932643, -0.18043950812909038, -0.0921534279978055, 0.10099356685156655, 0.18903604406975974, -0.15174000628449463, -0.41148800635102206, -0.566803846861678, -0.5115463032133246, -0.4129540572098877, -0.24028247811734693, -0.23977254169195888, -0.345077903898352, -0.241778997730978, -0.10766740461698888, -0.21835428157464457, -0.09230638613298363, -0.1284446395086948, -0.5192175147934049, -0.4351522788387683, -0.5998272027681343, -0.5675233644782293, -0.29772182900366384, -0.2973449941751325, -0.048187728449152666, -0.39293515187697864, -0.4421070854547212, -0.352408459392467, -0.5879522290161076, -0.2238498370045122, -0.09526501886026201, 0.007208237516608921, 0.19395301485279565, -0.11300521930202113, -0.11262402645988066, -0.15153283209957735, -0.3712153748258471, -0.1459983507594029, -0.1567300858462336, -0.18707999985448762, 0.23432297253693712, 0.16846254945019018, 0.07629297631676758, 0.19136254912494025, -0.12062080957902285, -0.32023983064470013, -0.04910129955080258, 0.0015425908560119479, -0.044204928981273914, 0.09871775263329234, -0.009079933122504033, -0.28594055973071747, -0.30670099144406304, -0.177820902544205, -0.09656446131626387, -0.015583447727136416, -0.3277693404416181, -0.4282959614885696, -0.5048961466647641, -0.5582089570104771, -0.2812038900059238, -0.12876376332627615, -0.34552882475842406, -0.28813538104215924, 0.030640225348324696, 0.0016523068854503661, -0.14345942998926606, -0.04468268163652816, -0.31162496954386854, -0.1450758615164144, 0.30012179559782776, 0.20618762476249392, -0.055158004203827576, -0.20430842352277223, -0.7069182028239812, -0.8205920021670954, -0.4099852583386871, -0.27801002398188, 0.21945954110074956, 0.4101198038162659, 0.4701765419411601, 0.302559158685815, 0.0697361625789132, -0.09454933461102194, -0.2318322222960131, -0.02752833201168319, 0.13465278700133865, 0.4222037190408889, 0.0, 0.0, 0.0, 0.0, 0.0]] caption="Water Vapor Number Density"
  out "CH 1 (WV off) counts display":dbl[][](graph)=[[67.32, 72.32, 54.31999999999999, 35.31999999999999, 40.31999999999999, 63.31999999999999, 69.32, 62.31999999999999, 52.31999999999999, 57.31999999999999, 66.32, 84.32, 103.32, 59.31999999999999, 74.32, 91.32, 84.32, 100.32, 94.32, 94.32, 137.32, 99.32, 104.32, 121.32, 120.32, 129.32, 130.32, 137.32, 127.32, 139.32, 130.32, 146.32, 138.32, 129.32, 149.32, 154.32, 145.32, 163.32, 136.32, 156.32, 139.32, 141.32, 101.32, 124.32, 119.32, 151.32, 140.32, 131.32, 152.32, 153.32, 150.32, 122.32, 109.32, 114.32, 115.32, 101.32, 84.32, 95.32, 76.32, 96.32, 85.32, 87.32, 96.32, 75.32, 97.32, 64.32, 79.32, 57.31999999999999, 83.32, 98.32, 57.31999999999999, 72.32, 114.32, 85.32, 77.32, 65.32, 68.32, 70.32, 112.32, 69.32, 59.31999999999999, 76.32, 51.31999999999999, 41.31999999999999, 73.32, 37.31999999999999, 46.31999999999999, 18.319999999999993, 36.31999999999999, 44.31999999999999, 57.31999999999999, 40.31999999999999, 24.319999999999993, 12.319999999999993, 15.319999999999993, 22.319999999999993, 18.319999999999993, 14.319999999999993, 42.31999999999999, 15.319999999999993, 10.319999999999993, 6.319999999999993, 18.319999999999993, 41.31999999999999, 12.319999999999993, 17.319999999999993, 3.319999999999993, 19.319999999999993, 20.319999999999993, 43.31999999999999, 24.319999999999993, 43.31999999999999, 65.32, 153.32, 249.32, 361.32, 500.32, 608.3199999999999, 935.3199999999999, 1167.32, 1537.32, 2033.32, 2562.32, 3109.32, 3585.32, 3781.32, 3650.32, 3442.32, 3096.32, 2960.32, 2642.32, 2484.32, 2229.32, 1833.32, 1407.32, 1152.32, 937.3199999999999, 797.3199999999999, 653.3199999999999, 589.3199999999999, 449.32, 426.32, 441.32, 479.32, 498.32, 445.32, 420.32, 428.32, 354.32, 309.32, 248.32, 214.32, 225.32, 264.32, 261.32, 257.32, 271.32, 187.32, 146.32, 129.32, 109.32, 97.32, 70.32, 46.31999999999999, 38.31999999999999, -0.6800000000000068, 11.319999999999993, 0.3199999999999932, -2.680000000000007, 4.319999999999993, -8.680000000000007, 4.319999999999993, 13.319999999999993, 0.3199999999999932, -7.680000000000007, -14.680000000000007, -3.680000000000007, -6.680000000000007, -7.680000000000007, -10.680000000000007, 9.319999999999993, -3.680000000000007, -8.680000000000007, 1.3199999999999932, -17.680000000000007, 9.319999999999993, 7.319999999999993, 8.319999999999993, 15.319999999999993, -8.680000000000007, -1.6800000000000068, 21.319999999999993, 0.3199999999999932, 1.3199999999999932, 12.319999999999993, 7.319999999999993, -3.680000000000007, -2.680000000000007, 9.319999999999993, -1.6800000000000068, -7.680000000000007, 9.319999999999993, 4.319999999999993, -11.680000000000007, 2.319999999999993, 12.319999999999993, 9.319999999999993, 0.3199999999999932, 1.3199999999999932, 3.319999999999993, -11.680000000000007, 6.319999999999993, -23.680000000000007, -17.680000000000007, -2.680000000000007, -4.680000000000007, 5.319999999999993, 9.319999999999993, -9.680000000000007, -3.680000000000007, -5.680000000000007, 2.319999999999993, -10.680000000000007, -4.680000000000007, -3.680000000000007, 0.3199999999999932, -1.6800000000000068, 16.319999999999993, -7.680000000000007, -0.6800000000000068, 21.319999999999993, 2.319999999999993, 9.319999999999993, 0.3199999999999932, 19.319999999999993, 11.319999999999993, -7.680000000000007, 16.319999999999993, 3.319999999999993, -3.680000000000007, 1.3199999999999932, 3.319999999999993, -0.6800000000000068, -1.6800000000000068, 0.3199999999999932, 14.319999999999993, -9.680000000000007, 16.319999999999993, -16.680000000000007, -19.680000000000007, -17.680000000000007, 0.3199999999999932, 4.319999999999993, 1.3199999999999932, -4.680000000000007, 1.3199999999999932, -8.680000000000007, 7.319999999999993, -4.680000000000007, -6.680000000000007, -1.6800000000000068, -0.6800000000000068, 5.319999999999993, -6.680000000000007, 4.319999999999993, -6.680000000000007, 23.319999999999993, 8.319999999999993, 2.319999999999993, 5.319999999999993, -1.6800000000000068, 5.319999999999993, -2.680000000000007, 2.319999999999993, 1.3199999999999932, -3.680000000000007, 2.319999999999993, -1.6800000000000068, 7.319999999999993, 8.319999999999993, -12.680000000000007, 2.319999999999993, 3.319999999999993, 11.319999999999993, -9.680000000000007, 1.3199999999999932, 3.319999999999993, -10.680000000000007, -3.680000000000007, 2.319999999999993, 5.319999999999993, -4.680000000000007, -10.680000000000007, 15.319999999999993, -10.680000000000007, -9.680000000000007, 4.319999999999993, -21.680000000000007, 10.319999999999993, -6.680000000000007, -13.680000000000007, 19.319999999999993, -2.680000000000007, -27.680000000000007, 8.319999999999993, 10.319999999999993, 21.319999999999993, -4.680000000000007, 7.319999999999993, 2.319999999999993, -0.6800000000000068, -6.680000000000007, 8.319999999999993, 3.319999999999993, 22.319999999999993, -1.6800000000000068, -11.680000000000007, -10.680000000000007, -6.680000000000007, 19.319999999999993, 19.319999999999993, 0.3199999999999932, 11.319999999999993, -4.680000000000007, 3.319999999999993, 5.319999999999993, -0.6800000000000068, 2.319999999999993, -5.680000000000007, -7.680000000000007, -3.680000000000007, -2.680000000000007, -7.680000000000007, -3.680000000000007, 7.319999999999993, 0.3199999999999932, -5.680000000000007, 0.3199999999999932, 7.319999999999993, 9.319999999999993, 5.319999999999993, 2.319999999999993, -7.680000000000007, -3.680000000000007, 6.319999999999993, 7.319999999999993, 3.319999999999993, 16.319999999999993, 2.319999999999993, -4.680000000000007, 4.319999999999993, 5.319999999999993, 13.319999999999993, -0.6800000000000068, -9.680000000000007, -11.680000000000007, 16.319999999999993, 3.319999999999993, 17.319999999999993, 9.319999999999993, 3.319999999999993, -5.680000000000007, -8.680000000000007, -1.6800000000000068, -0.6800000000000068, -11.680000000000007, 4.319999999999993, -10.680000000000007, -3.680000000000007, -3.680000000000007, -3.680000000000007, -8.680000000000007, -4.680000000000007, 1.3199999999999932, -17.680000000000007, -1.6800000000000068, -1.6800000000000068, 7.319999999999993, -22.680000000000007, 7.319999999999993, 9.319999999999993, 6.319999999999993, -5.680000000000007, -4.680000000000007, 5.319999999999993, 0.3199999999999932, 6.319999999999993, 14.319999999999993, -4.680000000000007, 1.3199999999999932, 1.3199999999999932, 3.319999999999993, 1.3199999999999932, -3.680000000000007, 0.3199999999999932, 8.319999999999993, -0.6800000000000068, 0.3199999999999932, 10.319999999999993, 5.319999999999993, 11.319999999999993, 2.319999999999993, -8.680000000000007, -5.680000000000007, -6.680000000000007, -6.680000000000007, -12.680000000000007, -9.680000000000007, 8.319999999999993, 4.319999999999993, 9.319999999999993, -5.680000000000007, 3.319999999999993, -2.680000000000007, 4.319999999999993, -2.680000000000007, 12.319999999999993, 4.319999999999993, -7.680000000000007, 15.319999999999993, -5.680000000000007, -2.680000000000007, 6.319999999999993, -0.6800000000000068, -7.680000000000007, -4.680000000000007, 18.319999999999993, 3.319999999999993, -16.680000000000007, 12.319999999999993, 9.319999999999993, 9.319999999999993, 2.319999999999993, -16.680000000000007, 4.319999999999993, 2.319999999999993, 13.319999999999993, -2.680000000000007, 1.3199999999999932, 2.319999999999993, -4.680000000000007, 2.319999999999993, 2.319999999999993, 0.3199999999999932, 26.319999999999993, 10.319999999999993, 2.319999999999993, -2.680000000000007, 8.319999999999993, 5.319999999999993, 10.319999999999993, 3.319999999999993, 8.319999999999993, 13.319999999999993, -6.680000000000007, -2.680000000000007, -15.680000000000007, 7.319999999999993, 2.319999999999993, 14.319999999999993, 7.319999999999993, 6.319999999999993, 6.319999999999993, 7.319999999999993, -0.6800000000000068, 5.319999999999993, 17.319999999999993, -10.680000000000007, -2.680000000000007, -10.680000000000007, 9.319999999999993, -5.680000000000007, 9.319999999999993, 2.319999999999993, 11.319999999999993, 6.319999999999993, -2.680000000000007, -4.680000000000007, 5.319999999999993, 14.319999999999993, 1.3199999999999932, -7.680000000000007, -0.6800000000000068, -17.680000000000007, -3.680000000000007, 12.319999999999993, -6.680000000000007, 7.319999999999993, 14.319999999999993, -10.680000000000007, 0.3199999999999932, -16.680000000000007, 0.3199999999999932, 14.319999999999993, 0.3199999999999932, 11.319999999999993, 1.3199999999999932, 0.3199999999999932, -6.680000000000007, 6.319999999999993, -5.680000000000007, 1.3199999999999932, 6.319999999999993, 15.319999999999993, -0.6800000000000068, -10.680000000000007, 13.319999999999993, 8.319999999999993, -5.680000000000007, -2.680000000000007, -10.680000000000007, 5.319999999999993, 26.319999999999993, 19.319999999999993, 5.319999999999993, 1.3199999999999932, 25.319999999999993, -2.680000000000007, -6.680000000000007, -5.680000000000007, -19.680000000000007, 1.3199999999999932, 7.319999999999993, -12.680000000000007, 6.319999999999993, 9.319999999999993, 9.319999999999993, -0.6800000000000068, -12.680000000000007, 16.319999999999993, -7.680000000000007, 0.3199999999999932, -16.680000000000007, -8.680000000000007, -10.680000000000007, 4.319999999999993, 2.319999999999993, 3.319999999999993, -0.6800000000000068, -0.6800000000000068, -4.680000000000007, 4.319999999999993, 2.319999999999993, -9.680000000000007, 2.319999999999993, 12.319999999999993, 2.319999999999993, 0.3199999999999932, -8.680000000000007, 17.319999999999993, 6.319999999999993, 5.319999999999993, 13.319999999999993, -3.680000000000007, 2.319999999999993, -2.680000000000007, -10.680000000000007, -22.680000000000007, -3.680000000000007, 0.0]] caption="Water Vapor Number Density"
  out "CH 3 (HSRL comb) counts display":dbl[][](graph)=[[175.76, 44.75999999999999, 32.75999999999999, 72.75999999999999, 15.759999999999991, 26.75999999999999, 96.75999999999999, 72.75999999999999, 82.75999999999999, 40.75999999999999, 82.75999999999999, 123.75999999999999, 69.75999999999999, 95.75999999999999, 105.75999999999999, 118.75999999999999, 81.75999999999999, 84.75999999999999, 153.76, 193.76, 106.75999999999999, 228.76, 210.76, 153.76, 208.76, 170.76, 180.76, 208.76, 269.76, 218.76, 232.76, 193.76, 222.76, 174.76, 145.76, 258.76, 181.76, 258.76, 231.76, 237.76, 200.76, 220.76, 234.76, 184.76, 237.76, 208.76, 210.76, 150.76, 188.76, 220.76, 216.76, 187.76, 160.76, 158.76, 152.76, 155.76, 115.75999999999999, 111.75999999999999, 108.75999999999999, 101.75999999999999, 102.75999999999999, 160.76, 152.76, 138.76, 95.75999999999999, 105.75999999999999, 52.75999999999999, 85.75999999999999, 120.75999999999999, 62.75999999999999, 98.75999999999999, 105.75999999999999, 91.75999999999999, 29.75999999999999, 111.75999999999999, 111.75999999999999, 32.75999999999999, 79.75999999999999, 82.75999999999999, 92.75999999999999, 60.75999999999999, 60.75999999999999, 15.759999999999991, 60.75999999999999, 14.759999999999991, 57.75999999999999, 59.75999999999999, 70.75999999999999, 65.75999999999999, 30.75999999999999, 84.75999999999999, 6.759999999999991, 32.75999999999999, 8.759999999999991, 13.759999999999991, 59.75999999999999, 25.75999999999999, 34.75999999999999, 32.75999999999999, 9.759999999999991, -4.240000000000009, 16.75999999999999, 14.759999999999991, 65.75999999999999, 29.75999999999999, 11.759999999999991, 56.75999999999999, 36.75999999999999, 3.759999999999991, 9.759999999999991, 64.75999999999999, 63.75999999999999, 72.75999999999999, 138.76, 221.76, 340.76, 478.76, 656.76, 928.76, 1199.76, 1441.76, 1982.76, 2581.76, 3187.76, 3657.76, 3744.76, 3807.76, 3394.76, 3075.76, 3067.76, 2645.76, 2431.76, 2085.76, 1767.76, 1414.76, 1167.76, 976.76, 785.76, 676.76, 570.76, 515.76, 467.76, 494.76, 414.76, 443.76, 474.76, 446.76, 393.76, 379.76, 303.76, 261.76, 286.76, 273.76, 257.76, 270.76, 285.76, 234.76, 316.76, 171.76, 125.75999999999999, 101.75999999999999, 110.75999999999999, 56.75999999999999, 9.759999999999991, 16.75999999999999, 3.759999999999991, 59.75999999999999, -21.24000000000001, 9.759999999999991, 0.7599999999999909, 36.75999999999999, 8.759999999999991, -37.24000000000001, -11.240000000000009, -7.240000000000009, -53.24000000000001, -0.2400000000000091, 41.75999999999999, 15.759999999999991, -16.24000000000001, 21.75999999999999, -9.240000000000009, 47.75999999999999, 17.75999999999999, -0.2400000000000091, -18.24000000000001, 62.75999999999999, 26.75999999999999, 45.75999999999999, -4.240000000000009, -12.240000000000009, -13.240000000000009, -36.24000000000001, 41.75999999999999, 39.75999999999999, -16.24000000000001, 27.75999999999999, -0.2400000000000091, -20.24000000000001, -28.24000000000001, -26.24000000000001, -17.24000000000001, -1.240000000000009, -18.24000000000001, 0.7599999999999909, -6.240000000000009, 19.75999999999999, -33.24000000000001, -4.240000000000009, -4.240000000000009, -3.240000000000009, 5.759999999999991, -42.24000000000001, -13.240000000000009, -10.240000000000009, -33.24000000000001, -16.24000000000001, 8.759999999999991, 22.75999999999999, 38.75999999999999, -16.24000000000001, -35.24000000000001, 28.75999999999999, -15.240000000000009, -36.24000000000001, -44.24000000000001, -51.24000000000001, -34.24000000000001, 21.75999999999999, -3.240000000000009, -32.24000000000001, 35.75999999999999, 3.759999999999991, -16.24000000000001, -30.24000000000001, -12.240000000000009, 10.759999999999991, 16.75999999999999, -0.2400000000000091, -15.240000000000009, 48.75999999999999, -29.24000000000001, -4.240000000000009, 6.759999999999991, 0.7599999999999909, -40.24000000000001, -4.240000000000009, 5.759999999999991, 9.759999999999991, -16.24000000000001, -13.240000000000009, -7.240000000000009, 5.759999999999991, 16.75999999999999, -56.24000000000001, 9.759999999999991, 7.759999999999991, -45.24000000000001, 12.759999999999991, 18.75999999999999, 19.75999999999999, -14.240000000000009, -16.24000000000001, 12.759999999999991, 10.759999999999991, -72.24000000000001, 15.759999999999991, -41.24000000000001, 14.759999999999991, -44.24000000000001, -1.240000000000009, -15.240000000000009, -39.24000000000001, 48.75999999999999, -18.24000000000001, -16.24000000000001, 14.759999999999991, 7.759999999999991, 14.759999999999991, 11.759999999999991, -14.240000000000009, -1.240000000000009, 30.75999999999999, 25.75999999999999, -29.24000000000001, -35.24000000000001, -10.240000000000009, 12.759999999999991, 42.75999999999999, -45.24000000000001, -31.24000000000001, -53.24000000000001, 17.75999999999999, 41.75999999999999, 5.759999999999991, 66.75999999999999, -9.240000000000009, 29.75999999999999, -20.24000000000001, -19.24000000000001, -30.24000000000001, -29.24000000000001, 17.75999999999999, -2.240000000000009, 23.75999999999999, 13.759999999999991, -7.240000000000009, -33.24000000000001, 1.759999999999991, -2.240000000000009, 15.759999999999991, 7.759999999999991, -10.240000000000009, -18.24000000000001, 13.759999999999991, -29.24000000000001, 5.759999999999991, -22.24000000000001, 21.75999999999999, 38.75999999999999, -13.240000000000009, 50.75999999999999, -32.24000000000001, 6.759999999999991, 16.75999999999999, -8.240000000000009, 51.75999999999999, 29.75999999999999, 13.759999999999991, -14.240000000000009, -30.24000000000001, -37.24000000000001, 40.75999999999999, -1.240000000000009, 1.759999999999991, -14.240000000000009, 24.75999999999999, -8.240000000000009, 10.759999999999991, -41.24000000000001, 32.75999999999999, 60.75999999999999, 20.75999999999999, -10.240000000000009, 19.75999999999999, -11.240000000000009, 16.75999999999999, -14.240000000000009, 25.75999999999999, 32.75999999999999, 15.759999999999991, -17.24000000000001, -2.240000000000009, -8.240000000000009, -36.24000000000001, 20.75999999999999, 23.75999999999999, -26.24000000000001, 8.759999999999991, 38.75999999999999, -8.240000000000009, -23.24000000000001, -67.24000000000001, -16.24000000000001, -17.24000000000001, 14.759999999999991, 38.75999999999999, -56.24000000000001, -38.24000000000001, 4.759999999999991, 4.759999999999991, -10.240000000000009, 65.75999999999999, -19.24000000000001, 25.75999999999999, 10.759999999999991, -7.240000000000009, -4.240000000000009, 31.75999999999999, 6.759999999999991, 13.759999999999991, -16.24000000000001, 50.75999999999999, 5.759999999999991, 96.75999999999999, -9.240000000000009, -14.240000000000009, 15.759999999999991, 0.7599999999999909, 17.75999999999999, -9.240000000000009, -11.240000000000009, 2.759999999999991, 15.759999999999991, -15.240000000000009, -5.240000000000009, -7.240000000000009, -38.24000000000001, -59.24000000000001, 4.759999999999991, -3.240000000000009, -15.240000000000009, -15.240000000000009, 58.75999999999999, -20.24000000000001, -16.24000000000001, -11.240000000000009, -6.240000000000009, 9.759999999999991, -7.240000000000009, 3.759999999999991, -7.240000000000009, -10.240000000000009, 26.75999999999999, -3.240000000000009, -11.240000000000009, -22.24000000000001, -40.24000000000001, 22.75999999999999, -35.24000000000001, 10.759999999999991, -6.240000000000009, -11.240000000000009, -43.24000000000001, -12.240000000000009, -31.24000000000001, -59.24000000000001, 35.75999999999999, 13.759999999999991, 13.759999999999991, -26.24000000000001, -50.24000000000001, -16.24000000000001, 6.759999999999991, 33.75999999999999, 20.75999999999999, 3.759999999999991, -25.24000000000001, -22.24000000000001, 37.75999999999999, -9.240000000000009, 4.759999999999991, 12.759999999999991, 1.759999999999991, -3.240000000000009, 51.75999999999999, 50.75999999999999, -1.240000000000009, -15.240000000000009, 15.759999999999991, -17.24000000000001, 33.75999999999999, 7.759999999999991, -0.2400000000000091, 12.759999999999991, 35.75999999999999, -43.24000000000001, -31.24000000000001, -0.2400000000000091, -18.24000000000001, 32.75999999999999, 15.759999999999991, -0.2400000000000091, 42.75999999999999, 44.75999999999999, -5.240000000000009, 24.75999999999999, -40.24000000000001, -25.24000000000001, 14.759999999999991, 16.75999999999999, 3.759999999999991, 15.759999999999991, 2.759999999999991, 3.759999999999991, -4.240000000000009, -4.240000000000009, -3.240000000000009, 2.759999999999991, -48.24000000000001, 31.75999999999999, -43.24000000000001, 6.759999999999991, -20.24000000000001, -13.240000000000009, -6.240000000000009, -21.24000000000001, 4.759999999999991, -57.24000000000001, -29.24000000000001, -28.24000000000001, 30.75999999999999, -23.24000000000001, -17.24000000000001, -3.240000000000009, 8.759999999999991, 14.759999999999991, 6.759999999999991, 36.75999999999999, -25.24000000000001, -14.240000000000009, 3.759999999999991, -23.24000000000001, -3.240000000000009, 11.759999999999991, -2.240000000000009, -65.24000000000001, -42.24000000000001, -41.24000000000001, 64.75999999999999, 0.7599999999999909, -21.24000000000001, -2.240000000000009, 58.75999999999999, -27.24000000000001, -32.24000000000001, 2.759999999999991, -0.2400000000000091, -21.24000000000001, -4.240000000000009, 53.75999999999999, 22.75999999999999, 4.759999999999991, -18.24000000000001, -26.24000000000001, -0.2400000000000091, -60.24000000000001, 6.759999999999991, 14.759999999999991, 2.759999999999991, 5.759999999999991, -7.240000000000009, 34.75999999999999, 44.75999999999999, -36.24000000000001, -32.24000000000001, 13.759999999999991, -2.240000000000009, 19.75999999999999, 22.75999999999999, 25.75999999999999, -18.24000000000001, -27.24000000000001, -2.240000000000009, 0.7599999999999909, 6.759999999999991, -17.24000000000001, -29.24000000000001, -3.240000000000009, 25.75999999999999, 27.75999999999999, -26.24000000000001, -35.24000000000001, 22.75999999999999, 17.75999999999999, 21.75999999999999, 31.75999999999999, -21.24000000000001, 13.759999999999991, 0.0]] caption="Water Vapor Number Density"
  out "CH3 (HSRL combined) smooth S":dbl[](array[numeric])=[92.31466666666667, 54.048, 54.998000000000005, 59.789666666666676, 63.998000000000005, 71.50633333333334, 80.09800000000001, 85.31466666666668, 88.91466666666668, 92.41466666666669, 97.88133333333334, 107.03966666666668, 117.18966666666668, 128.8396666666667, 140.3896666666667, 148.08966666666666, 159.59799999999998, 170.88133333333332, 179.64799999999997, 188.03966666666668, 195.46466666666663, 202.30633333333333, 206.18966666666665, 208.6063333333333, 207.72299999999998, 208.04799999999997, 209.7063333333333, 212.93966666666665, 218.20633333333333, 220.78966666666668, 225.63133333333332, 226.6563333333333, 226.4813333333333, 227.48133333333334, 226.97299999999998, 228.148, 227.348, 226.24799999999996, 220.423, 213.57299999999998, 203.498, 195.78966666666665, 188.373, 188.123, 194.16466666666668, 193.75633333333332, 195.63133333333332, 189.18966666666665, 175.9646666666667, 163.02300000000002, 149.96466666666666, 138.78966666666668, 133.16466666666665, 130.38966666666667, 125.29799999999999, 118.99799999999999, 113.923, 110.35633333333332, 108.66466666666666, 109.37299999999999, 106.66466666666665, 99.298, 96.26466666666667, 96.18133333333334, 97.63966666666667, 100.08133333333333, 96.65633333333332, 91.10633333333332, 85.98966666666668, 87.44800000000001, 90.21466666666666, 92.48133333333332, 93.25633333333334, 90.66466666666668, 87.38133333333336, 84.81466666666668, 81.48966666666668, 74.64800000000002, 70.87300000000002, 62.57300000000001, 57.42300000000001, 52.656333333333336, 45.306333333333335, 44.323, 37.964666666666666, 32.58966666666666, 29.406333333333333, 27.28966666666667, 27.28966666666667, 30.181333333333335, 30.989666666666665, 26.339666666666666, 26.214666666666666, 22.139666666666663, 18.20633333333333, 18.789666666666665, 17.00633333333333, 17.323, 18.122999999999998, 17.90633333333333, 18.439666666666664, 18.772999999999996, 19.63133333333333, 20.18133333333333, 20.70633333333333, 21.431333333333335, 21.989666666666665, 24.281333333333333, 28.314666666666664, 36.698, 51.048, 74.68966666666665, 110.34799999999998, 161.63966666666664, 238.96466666666663, 348.8313333333333, 501.59799999999996, 706.4146666666666, 943.3563333333334, 1204.5563333333334, 1469.0563333333337, 1720.7230000000006, 1948.939666666667, 2132.806333333334, 2248.648, 2292.264666666667, 2276.239666666667, 2220.989666666667, 2154.3230000000003, 2081.031333333334, 1990.814666666667, 1884.606333333334, 1764.139666666667, 1625.506333333334, 1479.539666666667, 1322.6979999999999, 1152.5230000000001, 982.1896666666668, 838.1896666666667, 723.3896666666667, 653.9396666666668, 624.4480000000001, 619.4563333333334, 619.0896666666667, 616.6563333333334, 605.0646666666667, 577.298, 552.723, 521.0646666666668, 487.098, 449.88966666666664, 412.49799999999993, 376.24799999999993, 340.95633333333325, 315.1063333333333, 282.6646666666666, 250.16466666666668, 216.38133333333332, 178.123, 147.43133333333333, 118.56466666666665, 99.40633333333334, 82.43966666666668, 70.18966666666668, 58.08966666666668, 48.398, 37.98966666666667, 23.872999999999998, 18.864666666666665, 11.264666666666665, 5.606333333333332, 2.164666666666665, -1.0186666666666686, -4.643666666666669, -4.760333333333335, -2.1020000000000016, -5.452000000000002, -3.310333333333335, -1.0770000000000026, -2.277000000000002, -1.4520000000000017, -1.527000000000002, -3.8686666666666687, -3.1853333333333356, -1.0936666666666688, -5.560333333333336, -5.3353333333333355, -5.735333333333335, -6.2520000000000024, -3.3270000000000017, -2.1353333333333353, 0.18966666666666465, -1.9186666666666685, 0.022999999999998133, -2.6686666666666685, -4.943666666666669, -3.477000000000002, -7.110333333333335, -5.393666666666668, -5.885333333333335, -5.402000000000002, -4.818666666666669, -6.052000000000001, -6.343666666666668, -7.285333333333336, -5.643666666666668, -5.093666666666668, -6.927000000000001, -6.7103333333333355, -6.285333333333336, -3.6686666666666694, -3.1103333333333354, -2.327000000000002, -3.4353333333333356, -3.9103333333333348, -2.2353333333333354, -0.01866666666666883, 0.122999999999998, -0.677000000000002, -0.827000000000002, -1.5186666666666686, 0.29799999999999804, -0.06033333333333535, -1.302000000000002, -1.3270000000000022, -5.368666666666669, -5.968666666666668, -4.777000000000002, -5.393666666666669, -3.4270000000000023, -3.9186666666666685, -4.152000000000002, -4.268666666666668, -5.152000000000002, -4.427000000000002, -2.268666666666669, -4.885333333333335, -4.852000000000002, -3.485333333333335, -6.068666666666668, -3.2270000000000016, -1.452000000000002, -4.593666666666669, -2.927000000000002, -5.277000000000002, -5.227000000000002, -4.343666666666668, -3.2770000000000024, -1.152000000000002, -0.6936666666666685, 3.589666666666665, 0.28133333333333166, -2.5436666666666685, -2.7936666666666685, -6.7520000000000024, -4.127000000000002, -0.47700000000000187, -1.6686666666666685, -2.927000000000002, -5.068666666666669, -6.052000000000002, -7.3353333333333355, -5.660333333333335, -2.5353333333333348, -4.477000000000002, -4.218666666666669, -3.6353333333333353, -6.260333333333335, -4.993666666666669, -4.818666666666669, -2.9270000000000023, -1.3020000000000018, -2.1353333333333353, -1.777000000000002, -2.8936666666666686, -4.427000000000002, -3.3686666666666687, -2.3853333333333353, -2.560333333333335, -2.5686666666666684, -1.652000000000002, -2.485333333333335, -3.777000000000002, -3.1936666666666684, -3.752000000000002, -4.135333333333335, -5.2520000000000024, -4.268666666666669, -4.077000000000002, -1.9353333333333353, 2.2646666666666646, 1.0813333333333313, 2.2813333333333317, -0.5686666666666684, -1.6520000000000017, -1.3603333333333354, -1.3353333333333355, -1.302000000000002, -2.9853333333333354, -3.5020000000000024, -7.368666666666669, -4.643666666666669, -3.0353333333333357, -3.5520000000000023, -1.0186666666666688, -0.12700000000000222, -2.4270000000000023, 0.04799999999999793, 1.7396666666666647, -2.0186666666666686, -0.9936666666666688, -1.902000000000002, -4.060333333333335, -2.5686666666666684, -4.535333333333336, -5.127000000000002, -2.227000000000002, -3.252000000000002, -1.052000000000002, -1.127000000000002, -4.735333333333335, -2.8353333333333355, -2.0936666666666683, -1.8186666666666684, -2.027000000000002, -0.2853333333333352, -2.0103333333333353, -0.6186666666666687, 0.44799999999999807, -1.2353333333333352, -1.102000000000002, -2.902000000000002, -2.0103333333333353, -3.327000000000002, -3.5103333333333353, -2.635333333333335, -3.293666666666668, -3.4686666666666683, -0.252000000000002, -0.7603333333333355, -2.4936666666666687, -3.1353333333333353, -6.777000000000002, -4.468666666666669, -5.160333333333336, -3.027000000000002, -0.7520000000000018, -4.368666666666669, -2.943666666666669, -3.2686666666666686, -6.202000000000002, -5.760333333333335, -3.9520000000000017, -4.785333333333336, -3.443666666666669, -2.352000000000002, -2.693666666666669, -1.2853333333333352, -0.1353333333333353, -0.9936666666666687, -2.4603333333333355, -4.677000000000001, -6.568666666666669, -5.368666666666669, -5.077000000000002, -4.485333333333335, -2.660333333333335, -3.677000000000002, -1.535333333333335, -0.8853333333333353, -3.310333333333335, -3.152000000000002, -4.310333333333335, -4.802000000000002, -1.9603333333333353, -0.8353333333333354, -0.9020000000000019, -2.377000000000002, -3.277000000000002, -4.277000000000002, -5.777000000000002, -2.3853333333333353, -1.9436666666666687, -0.9853333333333354, 0.5396666666666647, -0.7686666666666686, -2.5103333333333353, -3.727000000000002, -5.760333333333335, -6.777000000000002, -4.343666666666668, -3.860333333333335, -3.7270000000000016, -3.6186666666666687, -6.035333333333335, -6.610333333333335, -5.452000000000002, -1.5103333333333349, 0.3313333333333313, -0.12700000000000178, 1.0979999999999985, -1.1103333333333354, 0.4896666666666649, 2.4396666666666644, 2.522999999999998, 3.731333333333331, 1.9729999999999979, 1.5396666666666647, 1.2646666666666646, 2.581333333333331, 0.8813333333333311, 1.3229999999999977, -0.24366666666666892, -3.2603333333333353, -2.352000000000002, -3.243666666666669, -4.077000000000002, -4.218666666666668, -4.4186666666666685, -4.010333333333335, -4.2936666666666685, -4.410333333333336, -6.118666666666668, -6.035333333333336, -2.818666666666669, -3.810333333333335, 0.18966666666666454, -0.39366666666666883, -0.5353333333333354, 2.6313333333333313, 2.439666666666665, 2.5063333333333313, 0.9479999999999982, -1.5186666666666686, -3.977000000000002, -3.943666666666669, -4.5020000000000024, -6.993666666666668, -6.527000000000002, -6.227000000000002, -4.235333333333335, -1.2936666666666683, -0.9686666666666687, -1.0686666666666687, -2.402000000000002, -2.5353333333333357, -2.160333333333335, -3.7603333333333353, -1.602000000000002, -2.6770000000000023, 1.0646666666666644, 2.5146666666666646, 1.9729999999999979, 1.6229999999999984, -2.502000000000002, -2.343666666666669, -1.7103333333333353, 1.9479999999999977, 3.0063333333333313, 3.789666666666664, 3.356333333333331, 0.18966666666666487, -1.6686666666666685, -5.268666666666668, -7.318666666666669, -6.593666666666668, -6.660333333333335, -5.052000000000002, -2.068666666666669, -1.0520000000000023, 1.147999999999998, 2.1396666666666646, -1.7103333333333353, -4.618666666666669, -6.3353333333333355, -5.693666666666669, -4.577000000000003, -2.652000000000002, -2.6353333333333353, -3.7770000000000024, -2.6353333333333353, -1.1686666666666687, -2.3603333333333354, -0.9936666666666688, -1.377000000000002, -5.5436666666666685, -4.6270000000000024, -6.352000000000002, -5.985333333333336, -3.127000000000002, -3.110333333333335, -0.5020000000000018, -4.077000000000002, -4.568666666666669, -3.6270000000000024, -6.027000000000002, -2.2853333333333357, -0.9686666666666687, 0.07299999999999796, 1.9563333333333315, -1.1353333333333353, -1.127000000000002, -1.5103333333333355, -3.685333333333335, -1.4436666666666684, -1.5436666666666685, -1.8353333333333353, 2.2896666666666645, 1.6396666666666646, 0.7396666666666646, 1.847999999999998, -1.1603333333333352, -3.068666666666669, -0.46866666666666856, 0.01466666666666483, -0.41866666666666863, 0.9313333333333313, -0.08533333333333537, -2.677000000000002, -2.8603333333333354, -1.652000000000002, -0.8936666666666688, -0.14366666666666872, -3.0103333333333353, -3.9186666666666685, -4.602000000000002, -5.068666666666669, -2.5436666666666685, -1.1603333333333354, -3.102000000000002, -2.5770000000000017, 0.2729999999999979, 0.014666666666664663, -1.2686666666666686, -0.3936666666666687, -2.7353333333333354, -1.2686666666666686, 2.6146666666666647, 1.789666666666665, -0.4770000000000021, -1.7603333333333353, -6.068666666666669, -7.018666666666668, -3.4936666666666683, -2.360333333333336, 1.8563333333333314, 3.456333333333331, 3.9479999999999977, 2.531333333333331, 0.5813333333333315, -0.7853333333333353, -1.9186666666666685, -0.22700000000000187, 1.1063333333333314, 3.4563333333333315]
  out "CH3 (HSRL combined) smooth L":dbl[](array[numeric])=[96.13322222222223, 59.384611111111106, 60.53322222222222, 67.05961111111111, 75.32905555555554, 85.61794444444443, 94.09294444444444, 99.44016666666668, 105.14988888888891, 110.70822222222226, 119.01794444444448, 128.82488888888892, 139.1943333333334, 151.32488888888895, 163.18600000000004, 175.71238888888894, 190.7137777777778, 204.22766666666666, 218.98461111111112, 232.46794444444444, 242.61933333333334, 253.34988888888887, 260.1193333333333, 264.5373888888888, 268.41099999999994, 270.3346111111111, 273.6221111111111, 277.261, 280.1012777777778, 282.3248888888889, 283.4026666666667, 282.78461111111113, 281.4818333333333, 278.4582222222222, 273.1873888888889, 267.0873888888889, 259.16794444444446, 249.3096111111111, 238.68738888888888, 228.4346111111111, 218.67627777777778, 211.17072222222225, 205.85961111111115, 201.28877777777785, 199.32766666666674, 196.4929444444445, 191.8554444444445, 184.5165555555556, 174.1901666666667, 161.62211111111117, 149.51238888888895, 139.0707222222223, 131.23322222222228, 126.58183333333338, 122.2179444444445, 118.31238888888893, 114.46794444444447, 111.6165555555556, 108.59572222222226, 106.80961111111114, 103.89433333333334, 100.88183333333333, 99.25127777777776, 96.6832222222222, 95.17627777777776, 93.38461111111108, 90.5457222222222, 89.53183333333331, 88.72627777777774, 88.5693333333333, 88.5582222222222, 88.21655555555553, 86.99155555555554, 84.9082222222222, 81.85127777777774, 76.61655555555554, 71.56794444444444, 64.74988888888889, 58.736000000000004, 53.60961111111111, 48.85822222222222, 45.279055555555544, 42.24988888888887, 41.33461111111109, 39.806833333333316, 37.54294444444443, 35.962388888888874, 34.06516666666665, 32.62627777777776, 32.84294444444443, 32.5207222222222, 31.38322222222221, 30.212388888888874, 29.169333333333324, 28.029055555555544, 26.397111111111105, 25.876277777777773, 25.51794444444444, 24.252666666666666, 23.081833333333332, 21.449888888888893, 19.60544444444445, 19.14572222222223, 19.558222222222227, 20.55683333333334, 20.815166666666673, 20.79294444444445, 21.64155555555556, 21.327666666666673, 21.981833333333338, 25.259611111111113, 28.65544444444445, 35.01516666666667, 44.75405555555556, 57.74572222222221, 77.97349999999999, 105.02211111111109, 142.3332222222222, 187.6179444444444, 239.21516666666668, 296.62211111111117, 357.7735000000001, 423.213777777778, 494.67627777777795, 577.7721111111114, 687.3262777777779, 848.4984999999999, 1086.3818333333334, 1409.838777777778, 1794.3554444444446, 2193.412388888889, 2540.112388888889, 2779.0735, 2872.727666666666, 2810.779055555555, 2617.7832222222214, 2336.501277777778, 2023.251277777778, 1727.9693333333335, 1486.0637777777777, 1302.9623888888889, 1175.2262777777778, 1083.4901666666667, 1005.1929444444444, 931.2012777777776, 853.5846111111109, 771.8221111111109, 688.3832222222222, 604.0887777777778, 520.9929444444444, 444.8665555555555, 376.6971111111111, 320.12488888888885, 273.2040555555556, 234.7498888888889, 201.33600000000004, 170.54850000000005, 143.9054444444445, 117.52211111111113, 94.71794444444444, 75.33738888888888, 58.23322222222221, 45.597111111111104, 36.1471111111111, 27.722111111111104, 20.894333333333332, 14.767944444444442, 9.079055555555554, 6.251277777777777, 3.8193333333333332, 1.7651666666666666, 0.3026666666666669, -1.0639999999999998, -1.3709444444444443, -1.4209444444444443, -1.5653888888888887, -2.540388888888889, -2.3709444444444445, -2.339, -2.5181666666666667, -2.647333333333333, -2.889, -3.061222222222222, -1.4848333333333332, -0.3487222222222221, -1.586222222222222, -1.9431666666666665, -3.0792777777777776, -2.7556666666666665, -1.9542777777777776, -1.7334444444444443, -1.561222222222222, -2.0431666666666666, -2.0542777777777776, -1.9334444444444445, -2.7973333333333334, -3.5265, -2.7667777777777776, -2.2806666666666664, -1.4973333333333332, -1.437611111111111, -2.5501111111111108, -3.752888888888889, -4.7459444444444445, -4.519555555555556, -4.0487222222222226, -3.2917777777777775, -2.937611111111111, -2.6445555555555553, -2.283444444444444, -1.8709444444444445, -1.5792777777777776, -1.0584444444444443, -1.1723333333333332, -1.1653888888888888, -1.1334444444444443, -1.075111111111111, -0.4514999999999999, -1.1459444444444444, -0.3903888888888888, -0.450111111111111, -0.9723333333333333, -0.8737222222222221, -2.716777777777777, -3.401499999999999, -4.4417777777777765, -5.465388888888888, -4.379277777777777, -4.508444444444444, -3.868166666666666, -2.2167777777777777, -1.3042777777777776, -0.6014999999999999, -0.37927777777777766, -1.4612222222222222, -1.9639999999999997, -2.234833333333333, -1.9709444444444444, -0.47788888888888875, -1.2681666666666664, -1.6806666666666665, -1.4306666666666665, -1.1431666666666667, -0.6223333333333332, 0.3721111111111113, -0.1417777777777776, -1.189, -0.8195555555555555, -1.8653888888888888, -1.1084444444444443, -0.9931666666666668, -2.214, -2.666777777777778, -3.6320555555555556, -3.8917777777777776, -2.109833333333333, -1.2056666666666667, -1.0070555555555556, -0.5570555555555554, -1.9973333333333334, -2.0278888888888886, -1.6917777777777778, -1.5959444444444444, -1.2167777777777777, -1.1334444444444445, -1.6292777777777778, -2.0042777777777774, -2.1931666666666665, -1.311222222222222, -1.052888888888889, -1.2098333333333333, -0.012611111111111073, -0.44316666666666665, 0.8748888888888889, 0.42766666666666664, -0.6417777777777778, -1.1848333333333334, -2.6848333333333336, -0.9042777777777775, -0.15566666666666656, 0.7735000000000001, 1.0679444444444446, 0.43600000000000005, 0.7679444444444445, -0.3459444444444444, -1.1431666666666667, -2.0820555555555553, -2.7473333333333336, -2.3181666666666665, -1.2945555555555557, -0.10288888888888875, 0.20683333333333342, 1.3221111111111112, -0.009833333333333139, -0.08622222222222209, -1.3417777777777775, -2.1764999999999994, -2.0098333333333334, -3.2153888888888886, -1.7584444444444445, -2.3376111111111113, -1.8792777777777778, -0.3278888888888889, -1.3556666666666666, -0.41816666666666663, 0.3762777777777779, -1.1487222222222222, 0.033222222222222264, -0.22372222222222213, -1.2278888888888888, -1.5473333333333334, -1.6445555555555555, -1.9848333333333332, -1.9084444444444446, -1.9209444444444443, -3.068166666666667, -2.427888888888889, -2.751499999999999, -1.6667777777777772, -1.0862222222222218, -2.532055555555555, -2.3320555555555553, -2.7084444444444444, -2.809833333333333, -3.1598333333333333, -1.5056666666666665, -0.30288888888888876, -1.4792777777777772, -0.9403888888888884, -1.9709444444444437, -3.318166666666666, -2.468166666666667, -1.7417777777777776, -1.7778888888888886, -2.095944444444444, -1.2195555555555555, -1.1306666666666667, -1.600111111111111, 0.04155555555555568, -0.5417777777777777, -0.5834444444444443, -0.5903888888888887, -1.3014999999999999, -1.7709444444444444, -3.455666666666667, -3.127888888888889, -3.1515, -3.289, -1.8584444444444443, -1.836222222222222, -3.2112222222222218, -3.472333333333333, -2.982055555555555, -3.462611111111111, -2.1598333333333333, -1.0265, -2.0903888888888886, -1.537611111111111, -1.8223333333333331, -2.4792777777777775, -2.1070555555555557, -2.100111111111111, -1.7112222222222222, -0.3987222222222221, -0.15149999999999988, -0.35844444444444434, -1.4542777777777776, -2.0570555555555554, -1.3195555555555554, -0.886222222222222, 0.274888888888889, -0.5042777777777776, -0.4667777777777775, -0.14455555555555533, 0.020722222222222392, 1.1637777777777778, 0.2860000000000001, -0.9973333333333334, -0.6501111111111112, -1.9653888888888889, -2.6306666666666665, -0.6265, -1.1778888888888888, 0.7151666666666667, 2.174888888888889, 1.3096111111111113, 0.40266666666666695, -1.0209444444444444, -1.8028888888888888, -1.1306666666666665, -0.23205555555555546, 0.3235000000000001, 0.019333333333333425, -0.43761111111111106, -1.5265, -1.6612222222222222, -0.6167777777777776, -0.8292777777777777, 0.3082222222222223, 0.6179444444444445, 0.786, 0.7304444444444446, 0.6776666666666668, 0.8026666666666669, 0.0012777777777778776, -0.325111111111111, 0.008222222222222297, -0.5723333333333334, -0.11399999999999993, 0.9096111111111111, -0.10844444444444434, 0.7707222222222223, 0.4304444444444445, -0.10566666666666659, 0.7679444444444445, -0.19038888888888877, 0.46794444444444455, 0.02072222222222231, -0.20983333333333326, 0.49016666666666675, 0.21516666666666678, 0.3401666666666668, -0.027888888888888796, -0.9209444444444443, -1.1820555555555554, -2.1320555555555556, -1.2751111111111113, -0.8362222222222223, -0.9695555555555555, 0.2179444444444445, 0.17211111111111121, 0.2887777777777779, 0.16100000000000012, -0.9223333333333331, -1.9306666666666665, -1.2362222222222221, -0.9417777777777776, 0.3165555555555557, 0.9832222222222223, 0.9985000000000002, 1.040166666666667, 1.6193333333333335, 1.2387777777777778, 0.6332222222222224, 0.34572222222222226, -0.950111111111111, -0.07372222222222208, 0.19294444444444453, 0.062388888888888994, 0.22072222222222226, 0.6193333333333334, 1.0110000000000001, 1.4748888888888887, 2.1193333333333335, 1.0568333333333335, -0.10149999999999987, 0.3637777777777779, 0.9207222222222223, 0.5985000000000001, -0.4153888888888889, -1.2945555555555557, -2.937611111111111, -2.637611111111111, -2.6390000000000002, -2.9598333333333335, -1.6362222222222225, -2.1278888888888887, -0.689, 0.10266666666666677, -0.5139999999999999, 0.5623888888888889, 0.6457222222222223, 0.3137777777777779, -1.0056666666666665, -2.0792777777777776, -2.920944444444444, -2.516777777777777, -0.5653888888888889, -0.22233333333333322, -0.03344444444444428, -0.6528888888888889, -0.750111111111111, -2.3820555555555565, -2.0570555555555563, -1.6237222222222232, -2.5403888888888897, -2.0028888888888887, -2.773722222222222, -3.661222222222222, -3.170944444444444, -1.4876111111111108, -0.16261111111111093, 1.4318333333333335, 1.6290555555555557, 0.8123888888888889, 0.7554444444444446, -0.6237222222222221, -0.6514999999999999, -0.448722222222222, -1.2820555555555555, -1.4806666666666666, -1.5098333333333331, -1.5820555555555553, -0.9667777777777777, 0.4123888888888889, 0.6693333333333333, 1.2235, 1.4235, 0.8943333333333334, 0.4332222222222223, 0.6401666666666668, 0.8012777777777779, -0.09872222222222204, -0.5417777777777776, -0.9584444444444442, -1.4348333333333332, -0.5042777777777776, 0.5207222222222223, 0.4318333333333334, 0.26655555555555566, -0.4056666666666665, -0.49594444444444435, 0.09572222222222232, 0.5290555555555556, 0.774888888888889, 1.0707222222222224, 0.9596111111111112, -0.11122222222222211, 0.6262777777777779, -1.098722222222222, -1.5195555555555553, -0.6626111111111109, -1.237611111111111, -0.5278888888888889, -0.7417777777777776, -0.6403888888888888, -1.052888888888889, -1.3528888888888888, -1.2167777777777777, -1.6237222222222223, -0.975111111111111, -0.21538888888888877, 0.5526666666666668, 1.1568333333333334, 1.4193333333333333, 1.3026666666666666, 1.0637777777777777, 0.6429444444444445, 0.8068333333333334, 0.774888888888889, 0.015166666666666717, 0.3637777777777778, 0.36377777777777787, 0.3429444444444445, 0.8568333333333336]
  out "CH3 Bin Readings":dbl[](array[numeric])=[854.0, 723.0, 711.0, 751.0, 694.0, 705.0, 775.0, 751.0, 761.0, 719.0, 761.0, 802.0, 748.0, 774.0, 784.0, 797.0, 760.0, 763.0, 832.0, 872.0, 785.0, 907.0, 889.0, 832.0, 887.0, 849.0, 859.0, 887.0, 948.0, 897.0, 911.0, 872.0, 901.0, 853.0, 824.0, 937.0, 860.0, 937.0, 910.0, 916.0, 879.0, 899.0, 913.0, 863.0, 916.0, 887.0, 889.0, 829.0, 867.0, 899.0, 895.0, 866.0, 839.0, 837.0, 831.0, 834.0, 794.0, 790.0, 787.0, 780.0, 781.0, 839.0, 831.0, 817.0, 774.0, 784.0, 731.0, 764.0, 799.0, 741.0, 777.0, 784.0, 770.0, 708.0, 790.0, 790.0, 711.0, 758.0, 761.0, 771.0, 739.0, 739.0, 694.0, 739.0, 693.0, 736.0, 738.0, 749.0, 744.0, 709.0, 763.0, 685.0, 711.0, 687.0, 692.0, 738.0, 704.0, 713.0, 711.0, 688.0, 674.0, 695.0, 693.0, 744.0, 708.0, 690.0, 735.0, 715.0, 682.0, 688.0, 743.0, 742.0, 751.0, 817.0, 900.0, 1019.0, 1157.0, 1335.0, 1607.0, 1878.0, 2120.0, 2661.0, 3260.0, 3866.0, 4336.0, 4423.0, 4486.0, 4073.0, 3754.0, 3746.0, 3324.0, 3110.0, 2764.0, 2446.0, 2093.0, 1846.0, 1655.0, 1464.0, 1355.0, 1249.0, 1194.0, 1146.0, 1173.0, 1093.0, 1122.0, 1153.0, 1125.0, 1072.0, 1058.0, 982.0, 940.0, 965.0, 952.0, 936.0, 949.0, 964.0, 913.0, 995.0, 850.0, 804.0, 780.0, 789.0, 735.0, 688.0, 695.0, 682.0, 738.0, 657.0, 688.0, 679.0, 715.0, 687.0, 641.0, 667.0, 671.0, 625.0, 678.0, 720.0, 694.0, 662.0, 700.0, 669.0, 726.0, 696.0, 678.0, 660.0, 741.0, 705.0, 724.0, 674.0, 666.0, 665.0, 642.0, 720.0, 718.0, 662.0, 706.0, 678.0, 658.0, 650.0, 652.0, 661.0, 677.0, 660.0, 679.0, 672.0, 698.0, 645.0, 674.0, 674.0, 675.0, 684.0, 636.0, 665.0, 668.0, 645.0, 662.0, 687.0, 701.0, 717.0, 662.0, 643.0, 707.0, 663.0, 642.0, 634.0, 627.0, 644.0, 700.0, 675.0, 646.0, 714.0, 682.0, 662.0, 648.0, 666.0, 689.0, 695.0, 678.0, 663.0, 727.0, 649.0, 674.0, 685.0, 679.0, 638.0, 674.0, 684.0, 688.0, 662.0, 665.0, 671.0, 684.0, 695.0, 622.0, 688.0, 686.0, 633.0, 691.0, 697.0, 698.0, 664.0, 662.0, 691.0, 689.0, 606.0, 694.0, 637.0, 693.0, 634.0, 677.0, 663.0, 639.0, 727.0, 660.0, 662.0, 693.0, 686.0, 693.0, 690.0, 664.0, 677.0, 709.0, 704.0, 649.0, 643.0, 668.0, 691.0, 721.0, 633.0, 647.0, 625.0, 696.0, 720.0, 684.0, 745.0, 669.0, 708.0, 658.0, 659.0, 648.0, 649.0, 696.0, 676.0, 702.0, 692.0, 671.0, 645.0, 680.0, 676.0, 694.0, 686.0, 668.0, 660.0, 692.0, 649.0, 684.0, 656.0, 700.0, 717.0, 665.0, 729.0, 646.0, 685.0, 695.0, 670.0, 730.0, 708.0, 692.0, 664.0, 648.0, 641.0, 719.0, 677.0, 680.0, 664.0, 703.0, 670.0, 689.0, 637.0, 711.0, 739.0, 699.0, 668.0, 698.0, 667.0, 695.0, 664.0, 704.0, 711.0, 694.0, 661.0, 676.0, 670.0, 642.0, 699.0, 702.0, 652.0, 687.0, 717.0, 670.0, 655.0, 611.0, 662.0, 661.0, 693.0, 717.0, 622.0, 640.0, 683.0, 683.0, 668.0, 744.0, 659.0, 704.0, 689.0, 671.0, 674.0, 710.0, 685.0, 692.0, 662.0, 729.0, 684.0, 775.0, 669.0, 664.0, 694.0, 679.0, 696.0, 669.0, 667.0, 681.0, 694.0, 663.0, 673.0, 671.0, 640.0, 619.0, 683.0, 675.0, 663.0, 663.0, 737.0, 658.0, 662.0, 667.0, 672.0, 688.0, 671.0, 682.0, 671.0, 668.0, 705.0, 675.0, 667.0, 656.0, 638.0, 701.0, 643.0, 689.0, 672.0, 667.0, 635.0, 666.0, 647.0, 619.0, 714.0, 692.0, 692.0, 652.0, 628.0, 662.0, 685.0, 712.0, 699.0, 682.0, 653.0, 656.0, 716.0, 669.0, 683.0, 691.0, 680.0, 675.0, 730.0, 729.0, 677.0, 663.0, 694.0, 661.0, 712.0, 686.0, 678.0, 691.0, 714.0, 635.0, 647.0, 678.0, 660.0, 711.0, 694.0, 678.0, 721.0, 723.0, 673.0, 703.0, 638.0, 653.0, 693.0, 695.0, 682.0, 694.0, 681.0, 682.0, 674.0, 674.0, 675.0, 681.0, 630.0, 710.0, 635.0, 685.0, 658.0, 665.0, 672.0, 657.0, 683.0, 621.0, 649.0, 650.0, 709.0, 655.0, 661.0, 675.0, 687.0, 693.0, 685.0, 715.0, 653.0, 664.0, 682.0, 655.0, 675.0, 690.0, 676.0, 613.0, 636.0, 637.0, 743.0, 679.0, 657.0, 676.0, 737.0, 651.0, 646.0, 681.0, 678.0, 657.0, 674.0, 732.0, 701.0, 683.0, 660.0, 652.0, 678.0, 618.0, 685.0, 693.0, 681.0, 684.0, 671.0, 713.0, 723.0, 642.0, 646.0, 692.0, 676.0, 698.0, 701.0, 704.0, 660.0, 651.0, 676.0, 679.0, 685.0, 661.0, 649.0, 675.0, 704.0, 706.0, 652.0, 643.0, 701.0, 696.0, 700.0, 710.0, 657.0, 692.0]
  out "CH2 (molecular) smoothed":dbl[](array[numeric])=[23.608421052631577, 11.858421052631577, 7.147894736842102, 7.713684210526313, 5.266315789473682, 4.463684210526313, 5.924210526315786, 7.108421052631576, 6.950526315789471, 8.81894736842105, 8.095263157894733, 5.726842105263155, 7.608421052631577, 7.9636842105263135, 10.674210526315786, 13.08210526315789, 13.858421052631574, 17.095263157894735, 18.134736842105262, 17.38473684210526, 19.01631578947368, 19.082105263157892, 19.43736842105263, 20.24, 19.70052631578947, 16.29263157894737, 15.62157894736842, 17.81894736842105, 19.18736842105263, 22.22684210526316, 23.595263157894735, 21.161052631578944, 20.529473684210522, 21.292631578947365, 21.424210526315786, 24.042631578947365, 25.832105263157892, 24.634736842105262, 23.226842105263156, 24.25315789473684, 22.161052631578944, 22.674210526315786, 22.31894736842105, 18.345263157894735, 16.805789473684207, 16.029473684210522, 15.437368421052629, 15.397894736842101, 15.055789473684207, 14.187368421052629, 12.792631578947367, 13.50315789473684, 14.042631578947367, 14.029473684210524, 15.200526315789471, 11.463684210526313, 7.8847368421052595, 6.766315789473682, 3.6478947368421024, 5.674210526315786, 7.450526315789471, 6.06894736842105, 8.108421052631577, 9.055789473684207, 9.779473684210522, 11.779473684210522, 9.13473684210526, 8.411052631578944, 6.345263157894734, 3.7926315789473657, 5.661052631578945, 6.542631578947366, 7.713684210526312, 7.582105263157892, 7.9636842105263135, 5.608421052631575, 3.989999999999997, 4.253157894736839, 4.6873684210526285, 4.608421052631575, 4.489999999999997, 5.739999999999997, 1.0821052631578918, 1.6347368421052602, 1.38473684210526, -1.4047368421052662, 1.5163157894736812, 1.582105263157892, 1.31894736842105, 1.8715789473684183, 2.3715789473684183, 0.7794736842105235, 1.0689473684210498, 0.12157894736841834, -1.4442105263157925, -0.6284210526315819, -2.3521052631578976, -1.654736842105266, 0.5163157894736814, -0.8126315789473713, -2.023157894736845, -0.4573684210526343, -2.286315789473687, -0.06263157894737126, 2.226842105263155, 1.871578947368418, 2.1478947368421024, 0.8452631578947339, 3.1610526315789444, 3.8847368421052604, 4.95052631578947, 6.161052631578944, 5.766315789473682, 5.726842105263155, 7.279473684210524, 9.555789473684207, 15.108421052631577, 22.476842105263156, 29.647894736842105, 38.80578947368421, 43.81894736842105, 52.253157894736844, 61.411052631578954, 68.59526315789473, 77.0821052631579, 78.99, 77.21368421052631, 75.81894736842105, 71.18736842105262, 68.25315789473684, 64.46368421052632, 56.76631578947369, 53.397894736842105, 45.51631578947368, 38.647894736842105, 35.22684210526315, 26.818947368421046, 23.674210526315786, 19.687368421052625, 16.239999999999995, 14.358421052631577, 11.766315789473682, 13.595263157894735, 13.332105263157892, 15.976842105263156, 20.12157894736842, 20.726842105263156, 21.134736842105262, 17.884736842105262, 11.18736842105263, 9.042631578947365, 3.2926315789473657, 1.2399999999999975, 3.1478947368421024, 1.0821052631578918, 2.5426315789473657, 2.8978947368421024, 1.3847368421052604, 1.0557894736842077, 1.739999999999997, 1.8978947368421022, 2.279473684210523, 2.371578947368418, 1.8978947368421024, 2.1478947368421024, 1.0952631578947338, 0.8189473684210498, 1.8847368421052602, 1.2663157894736812, -0.6810526315789502, 1.8847368421052604, 1.226842105263155, 2.8715789473684183, 3.3715789473684183, -0.2994736842105292, -0.49684210526316075, -1.7600000000000025, -2.8257894736842135, -1.5889473684210556, -4.61526315789474, -4.667894736842108, -2.8389473684210556, -5.154736842105266, -1.891578947368424, -3.325789473684213, -2.9442105263157923, -2.8126315789473715, -2.2336842105263193, -1.5889473684210556, -4.18105263157895, -3.7731578947368454, -4.1152631578947405, -3.4442105263157927, -0.08894736842105555, -1.9968421052631609, -2.6810526315789502, -3.7073684210526343, -6.588947368421056, -2.404736842105266, -1.6810526315789502, -2.0363157894736874, -0.6942105263157923, -1.4178947368421082, -2.2205263157894763, -0.5889473684210554, 0.6347368421052603, 1.0689473684210498, -0.2600000000000027, -1.1415789473684237, -1.9836842105263184, -2.2073684210526343, -0.5494736842105292, 0.5426315789473656, 2.8978947368421024, 0.04263157894736569, 0.23999999999999694, -1.6284210526315819, -1.2336842105263188, 0.9373684210526287, 0.43736842105262885, 0.5163157894736814, -3.878421052631582, -4.549473684210529, -4.404736842105266, -3.852105263157898, -3.4310526315789502, -2.746842105263161, -6.023157894736846, -6.220526315789477, -4.404736842105266, -4.667894736842109, -2.6942105263157923, -3.036315789473687, -2.562631578947371, -3.2205263157894763, -1.1678947368421082, -0.49684210526316086, -0.22052631578947657, -1.0626315789473713, -3.1810526315789502, -5.628421052631582, -8.786315789473687, -6.417894736842108, -4.733684210526318, -2.312631578947371, -2.1152631578947396, -4.049473684210529, -4.352105263157897, -2.996842105263161, -1.5363157894736872, -2.2336842105263184, -2.3521052631578976, -3.6152631578947396, -3.996842105263161, -3.825789473684213, -5.43105263157895, -5.2863157894736865, -4.049473684210529, -1.9836842105263186, -1.2205263157894766, -1.904736842105266, -1.523157894736845, -1.010000000000003, 1.7794736842105234, 4.042631578947366, 3.2663157894736816, 2.4242105263157865, 0.4899999999999971, -2.9310526315789502, -4.233684210526318, -4.694210526315793, -5.246842105263161, -4.628421052631582, -1.4442105263157923, -1.6942105263157923, -1.273157894736845, 0.05578947368420767, -2.1284210526315817, -1.023157894736845, -0.33894736842105555, -3.4573684210526348, -3.2731578947368454, -4.944210526315793, -4.483684210526319, -3.7073684210526343, -3.3784210526315817, -5.023157894736845, -6.957368421052634, -5.18105263157895, -5.391578947368424, -1.023157894736845, -1.4047368421052662, -1.6678947368421082, -1.6415789473684241, -3.3915789473684237, -1.8652631578947396, -0.9705263157894766, -1.6678947368421082, -3.3389473684210556, -4.628421052631582, -3.220526315789477, -3.1942105263157927, -2.3257894736842135, -3.6152631578947396, -5.194210526315793, -6.0889473684210556, -6.207368421052635, -4.0100000000000025, -3.7863157894736874, -2.1810526315789502, -0.5626315789473713, -2.1415789473684237, -4.3126315789473715, -4.286315789473687, -5.707368421052634, -7.167894736842108, -8.312631578947371, -8.602105263157899, -9.878421052631582, -5.970526315789477, -2.470526315789477, -3.417894736842108, -1.1942105263157925, -2.9442105263157923, -2.68105263157895, -4.43105263157895, -5.970526315789477, -4.654736842105266, -6.207368421052634, -5.207368421052634, -3.1547368421052657, -2.6547368421052657, -1.3784210526315814, 1.0821052631578922, -0.15473684210526606, -0.20736842105263453, 2.358421052631576, 2.0689473684210498, 1.239999999999997, -1.0363157894736872, -4.11526315789474, -5.536315789473687, -4.023157894736845, -3.720526315789477, -3.825789473684213, -2.2336842105263184, -2.7336842105263184, -2.4573684210526343, -2.2336842105263184, -2.1547368421052657, -0.22052631578947635, 1.450526315789471, 0.20052631578947078, -0.510000000000003, -1.4310526315789502, -0.8915789473684241, -0.4442105263157924, -1.1284210526315819, -2.3915789473684237, -4.68105263157895, -5.0100000000000025, -4.141578947368424, -2.9968421052631604, -2.7336842105263184, -3.36526315789474, -2.378421052631582, -4.11526315789474, -4.641578947368425, -1.6810526315789502, -1.7994736842105294, -2.5363157894736874, -1.010000000000003, -3.8126315789473715, -4.773157894736845, -2.733684210526319, -4.628421052631582, -2.4573684210526348, -3.1810526315789502, -4.18105263157895, -2.799473684210529, -3.7994736842105294, -1.786315789473687, 0.2136842105263128, -0.773157894736845, -1.2994736842105292, -0.10210526315789759, 0.25315789473683914, 1.9110526315789444, 1.8715789473684181, -2.010000000000003, -3.6547368421052666, -3.3389473684210556, -1.5757894736842135, 0.3847368421052602, 1.1610526315789444, 1.2531578947368391, -0.8915789473684239, -1.3389473684210556, -3.2205263157894763, -2.404736842105266, -1.2205263157894763, -0.8652631578947397, 0.43736842105262874, -2.2336842105263184, -4.3389473684210556, -5.023157894736846, -5.6152631578947405, -5.3126315789473715, -1.786315789473687, 0.9768421052631552, 1.6873684210526285, 2.582105263157892, 1.608421052631576, -0.49684210526316075, -0.18105263157895024, -0.22052631578947657, -1.273157894736845, -0.07578947368421352, -1.036315789473687, -0.8652631578947397, 2.3584210526315763, 2.06894736842105, 2.726842105263155, 1.305789473684208, -0.4573684210526343, -1.4573684210526343, -2.6284210526315817, -1.799473684210529, -1.6678947368421082, -2.1810526315789502, -1.4442105263157923, -1.7336842105263188, -1.8257894736842135, -1.9442105263157923, -2.6415789473684237, 0.27947368421052343, -1.812631578947371, 0.055789473684207724, 1.2663157894736816, -2.904736842105266, 0.13473684210526016, -1.1284210526315817, -1.141578947368424, 0.45052631578947094, -2.2336842105263184, -3.4442105263157923, -2.4310526315789502, -3.4573684210526343, -2.6021052631578976, -1.391578947368424, -1.4836842105263188, -0.9573684210526345, -1.036315789473687, -2.273157894736845, -3.220526315789477, -2.746842105263161, -2.010000000000003, 0.38473684210526027, 0.7794736842105234, 0.09526315789473405, 0.12157894736841839, -1.5757894736842135, -2.9178947368421078, -1.0757894736842133, -3.325789473684213, -1.43105263157895, -0.7073684210526343, -5.18105263157895, -1.3521052631578978, -3.049473684210529, -4.128421052631582, -1.904736842105266, -3.3784210526315817, -1.3389473684210553, 0.8452631578947339, 1.4373684210526287, 0.5821052631578918, -1.8652631578947396, -2.470526315789477, -0.2863157894736872, 1.1478947368421024, 0.7136842105263126, 0.13473684210526005, -1.1021052631578976, -0.7863157894736872, -0.04947368421052922, -0.2336842105263186, 1.0031578947368391, 0.0031578947368391813, 0.5294736842105233, 0.7794736842105232, 0.6742105263157866, 1.2531578947368391, 0.5163157894736814, 0.1742105263157866, -2.246842105263161, -5.825789473684213, -3.0363157894736874, -2.049473684210529, 0.4505263157894711, 2.489999999999997, 0.8978947368421023, -0.7205263157894765, -2.023157894736845, -0.27315789473684493, -1.3389473684210553, -0.7468421052631609, 0.09526315789473394, 0.5163157894736812, 2.3057894736842073, 3.0952631578947343, -0.8257894736842131, -3.8126315789473715, -4.970526315789476, -5.18105263157895, -0.2994736842105292, 1.9110526315789444, 3.3847368421052604, 2.7531578947368396, 0.5821052631578918, -0.7468421052631606, -4.628421052631582, -3.7205263157894763, -4.273157894736845, -5.2863157894736865, -1.6152631578947398, -1.61526315789474, -1.1810526315789502, 0.7794736842105233, -1.3521052631578976, -2.1021052631578976, -1.9705263157894766, -0.8784210526315819, 1.1742105263157867, 1.3452631578947343, 1.6742105263157867, 1.345263157894734, -0.40473684210526606, 0.9242105263157866, 1.489999999999997, 0.595263157894734, 2.029473684210523, 1.7794736842105237, 3.2663157894736816, 3.6610526315789444, 3.9636842105263126, 4.424210526315787, 1.108421052631576, 0.5952631578947342, -0.010000000000002729, -2.246842105263161, -2.6021052631578976, -4.325789473684213, -6.010000000000003, -5.312631578947371]
  out "CH 2 Bin Readings":dbl[](array[numeric])=[447.0, 397.0, 404.0, 399.0, 396.0, 365.0, 395.0, 415.0, 394.0, 432.0, 392.0, 409.0, 402.0, 404.0, 385.0, 407.0, 354.0, 372.0, 379.0, 442.0, 388.0, 380.0, 421.0, 431.0, 429.0, 391.0, 412.0, 399.0, 410.0, 398.0, 406.0, 426.0, 411.0, 410.0, 421.0, 365.0, 402.0, 431.0, 426.0, 437.0, 394.0, 411.0, 393.0, 406.0, 406.0, 412.0, 352.0, 411.0, 425.0, 403.0, 432.0, 427.0, 389.0, 411.0, 421.0, 367.0, 445.0, 393.0, 417.0, 424.0, 422.0, 387.0, 386.0, 359.0, 384.0, 415.0, 434.0, 354.0, 434.0, 394.0, 373.0, 401.0, 420.0, 419.0, 394.0, 429.0, 399.0, 411.0, 384.0, 405.0, 409.0, 393.0, 399.0, 423.0, 426.0, 396.0, 418.0, 387.0, 412.0, 417.0, 398.0, 432.0, 391.0, 412.0, 428.0, 369.0, 409.0, 343.0, 416.0, 394.0, 412.0, 370.0, 406.0, 372.0, 449.0, 403.0, 435.0, 403.0, 393.0, 438.0, 423.0, 389.0, 391.0, 362.0, 418.0, 390.0, 412.0, 420.0, 381.0, 448.0, 425.0, 438.0, 476.0, 533.0, 530.0, 529.0, 522.0, 520.0, 476.0, 515.0, 471.0, 470.0, 469.0, 447.0, 462.0, 427.0, 416.0, 453.0, 400.0, 425.0, 431.0, 398.0, 416.0, 426.0, 387.0, 386.0, 371.0, 438.0, 423.0, 400.0, 387.0, 415.0, 395.0, 417.0, 417.0, 436.0, 399.0, 396.0, 373.0, 388.0, 406.0, 387.0, 393.0, 373.0, 409.0, 419.0, 409.0, 406.0, 388.0, 362.0, 406.0, 406.0, 421.0, 385.0, 366.0, 358.0, 417.0, 411.0, 381.0, 387.0, 399.0, 407.0, 423.0, 368.0, 426.0, 360.0, 399.0, 377.0, 377.0, 407.0, 435.0, 380.0, 416.0, 411.0, 394.0, 424.0, 401.0, 385.0, 394.0, 388.0, 359.0, 381.0, 411.0, 392.0, 407.0, 409.0, 376.0, 387.0, 375.0, 393.0, 431.0, 411.0, 387.0, 409.0, 364.0, 387.0, 398.0, 366.0, 413.0, 369.0, 363.0, 394.0, 364.0, 391.0, 372.0, 423.0, 366.0, 400.0, 403.0, 390.0, 401.0, 409.0, 391.0, 355.0, 406.0, 378.0, 404.0, 412.0, 390.0, 416.0, 421.0, 353.0, 420.0, 382.0, 429.0, 417.0, 394.0, 339.0, 393.0, 369.0, 415.0, 394.0, 436.0, 400.0, 416.0, 371.0, 426.0, 381.0, 383.0, 390.0, 390.0, 394.0, 371.0, 397.0, 414.0, 411.0, 371.0, 398.0, 397.0, 379.0, 391.0, 368.0, 372.0, 391.0, 373.0, 405.0, 374.0, 383.0, 376.0, 414.0, 349.0, 390.0, 400.0, 353.0, 393.0, 387.0, 383.0, 378.0, 381.0, 385.0, 368.0, 373.0, 385.0, 383.0, 391.0, 411.0, 422.0, 382.0, 374.0, 417.0, 385.0, 403.0, 408.0, 399.0, 398.0, 419.0, 381.0, 399.0, 389.0, 400.0, 405.0, 408.0, 370.0, 391.0, 391.0, 366.0, 425.0, 403.0, 382.0, 354.0, 407.0, 373.0, 370.0, 433.0, 417.0, 373.0, 403.0, 384.0, 407.0, 385.0, 392.0, 415.0, 388.0, 402.0, 406.0, 391.0, 399.0, 395.0, 393.0, 408.0, 381.0, 386.0, 383.0, 400.0, 435.0, 436.0, 378.0, 416.0, 377.0, 370.0, 383.0, 397.0, 390.0, 427.0, 391.0, 400.0, 362.0, 401.0, 414.0, 421.0, 401.0, 389.0, 388.0, 402.0, 372.0, 385.0, 373.0, 391.0, 407.0, 399.0, 369.0, 375.0, 398.0, 389.0, 377.0, 393.0, 381.0, 368.0, 340.0, 404.0, 369.0, 382.0, 374.0, 394.0, 374.0, 417.0, 391.0, 384.0, 408.0, 397.0, 381.0, 420.0, 403.0, 397.0, 414.0, 404.0, 421.0, 398.0, 433.0, 383.0, 376.0, 406.0, 351.0, 391.0, 413.0, 386.0, 357.0, 344.0, 404.0, 415.0, 383.0, 380.0, 400.0, 400.0, 394.0, 379.0, 338.0, 416.0, 387.0, 397.0, 397.0, 401.0, 388.0, 373.0, 403.0, 363.0, 381.0, 376.0, 366.0, 429.0, 379.0, 394.0, 391.0, 431.0, 399.0, 403.0, 402.0, 397.0, 417.0, 396.0, 391.0, 400.0, 396.0, 390.0, 371.0, 400.0, 436.0, 364.0, 383.0, 403.0, 420.0, 385.0, 413.0, 418.0, 397.0, 423.0, 389.0, 366.0, 411.0, 378.0, 362.0, 373.0, 391.0, 408.0, 370.0, 383.0, 406.0, 364.0, 387.0, 394.0, 389.0, 379.0, 406.0, 368.0, 373.0, 391.0, 381.0, 376.0, 368.0, 394.0, 411.0, 390.0, 380.0, 370.0, 407.0, 367.0, 372.0, 415.0, 431.0, 391.0, 403.0, 385.0, 416.0, 409.0, 383.0, 389.0, 374.0, 398.0, 402.0, 420.0, 415.0, 382.0, 394.0, 407.0, 389.0, 391.0, 406.0, 378.0, 378.0, 357.0, 371.0, 370.0, 428.0, 414.0, 390.0, 385.0, 397.0, 398.0, 408.0, 404.0, 390.0, 394.0, 384.0, 388.0, 392.0, 408.0, 343.0, 407.0, 396.0, 408.0, 383.0, 412.0, 394.0, 426.0, 387.0, 355.0, 409.0, 423.0, 404.0, 343.0, 395.0, 359.0, 397.0, 395.0, 366.0, 368.0, 378.0, 359.0, 417.0, 361.0, 370.0, 363.0, 450.0, 370.0, 395.0, 405.0, 383.0, 400.0, 467.0]
  in  "stop":bool
  in  "Reset Average":bool=TRUE
  in  "Save Data?":bool=TRUE
  in  "Collect Data?":bool=TRUE
  in  "ILX Address":i32=6 min=0 step=1
  in  "Lambda On DBR Current":dbl=171.13999999999868
  in  "Lambda Off DBR Current":dbl=172.9499999999997
  in  "Tab Control":T2(tab)=enum."OD"
  out "NRB plot":cluster{"Y":dbl[], "Y":dbl[]}[](graph)
  in  "background length":i32=25
  out "Correction":cluster{"Y":dbl[], "Y":dbl[]}[](graph)
  in  "dead time":dbl=3.7e-08
  out "Optical Depth":cluster{"Y":dbl[], "Y":dbl[]}[](graph) caption="XY Graph"
  out "CH1 RingBuffer long":dbl[][](array[numeric])
  out "CH1 RingBuffer short":dbl[][](array[numeric])
  in  "Weather":T3(tab)=enum."Pulse Energy (Micro Joule)"
  out "Temperature (C)":dbl(graph)=14.848290598290603
  out "Pressure (mb)":dbl(graph)=836.7032967032967
  out "Relative Humdity (%)":dbl(graph)=75.49297924297925
  out "Pulse Energy (Micro Joule)":T4(graph)={"Online Pulse Energy"=5.272677142857142, "Pulse Energy Offline"=5.267898571428572}
  out "?":cluster{"mean":dbl, "mean":dbl}(graph)={"mean"=22591.529576478828, "mean"=189916.69583479175}
  out "Index":i32=199
  out "CH1 (WV off) smooth L":dbl[](array[numeric])=[51.25333333333333, 48.361666666666665, 48.953333333333326, 50.411666666666655, 51.55333333333332, 53.219999999999985, 54.261666666666656, 56.41166666666665, 58.75333333333333, 61.394999999999996, 65.14499999999998, 68.91999999999999, 73.88666666666666, 78.66166666666665, 83.61166666666665, 87.63666666666664, 90.97833333333332, 96.35333333333332, 101.71166666666664, 106.48666666666665, 111.96166666666666, 114.06166666666667, 117.48666666666666, 120.26166666666667, 122.38666666666666, 125.67833333333333, 128.095, 131.62833333333333, 134.67833333333334, 137.74500000000003, 139.47833333333335, 141.21166666666667, 141.80333333333334, 142.37, 144.07833333333335, 145.51166666666668, 146.80333333333334, 145.51166666666666, 142.08666666666667, 136.645, 129.86166666666668, 128.64499999999998, 128.93666666666667, 130.9033333333333, 135.21166666666664, 134.36166666666665, 132.22833333333332, 129.02833333333334, 122.01166666666668, 114.43666666666667, 105.86999999999999, 97.27, 90.57833333333332, 87.62833333333332, 84.92833333333331, 84.01166666666664, 84.00333333333332, 81.75333333333332, 80.96999999999998, 77.70333333333332, 76.04499999999999, 74.11999999999998, 72.14499999999998, 71.87833333333333, 71.945, 72.76999999999998, 73.03666666666666, 72.16999999999999, 71.11166666666665, 71.81166666666665, 73.37833333333332, 74.59499999999998, 74.36166666666665, 71.98666666666665, 69.78666666666665, 67.27833333333332, 64.56166666666667, 61.603333333333325, 57.96166666666666, 53.769999999999996, 47.92833333333333, 43.40333333333333, 38.00333333333334, 34.06166666666667, 32.145, 30.328333333333337, 27.845000000000006, 28.170000000000005, 27.086666666666673, 26.153333333333336, 26.120000000000005, 23.503333333333337, 22.061666666666667, 19.278333333333336, 17.828333333333333, 17.53666666666667, 17.278333333333336, 17.71166666666667, 18.03666666666667, 17.520000000000003, 18.545, 18.378333333333334, 18.33666666666667, 19.520000000000003, 19.703333333333337, 20.645000000000003, 22.45333333333334, 23.570000000000007, 26.63666666666667, 34.986666666666665, 48.019999999999996, 71.12833333333332, 107.66999999999999, 157.34499999999997, 231.9783333333333, 335.695, 479.75333333333333, 669.595, 892.8200000000002, 1139.1866666666667, 1388.1200000000001, 1626.5366666666669, 1841.4450000000002, 2012.9783333333335, 2126.0283333333336, 2170.7783333333336, 2153.536666666667, 2096.7616666666668, 2026.2783333333336, 1949.2616666666668, 1863.6200000000003, 1765.8200000000002, 1649.0866666666668, 1520.3783333333336, 1381.611666666667, 1232.8700000000001, 1077.17, 920.8283333333334, 783.5783333333335, 678.6116666666668, 612.7783333333335, 582.9200000000002, 572.8866666666669, 572.4616666666669, 568.8866666666669, 555.9950000000001, 536.6700000000001, 512.8366666666667, 484.60333333333335, 454.68666666666667, 422.96999999999997, 387.12833333333333, 350.695, 317.295, 287.1283333333333, 257.8283333333333, 228.74499999999998, 198.31999999999994, 168.42833333333328, 141.5033333333333, 119.67833333333331, 100.2533333333333, 83.64499999999998, 68.90333333333332, 54.26999999999999, 43.33666666666666, 32.88666666666667, 25.470000000000002, 19.245, 13.728333333333333, 10.436666666666666, 5.97, 4.586666666666666, 3.3783333333333334, 2.2033333333333336, 1.8866666666666672, 0.6700000000000004, 0.8033333333333337, 0.3533333333333336, 0.38666666666666705, 0.086666666666667, -1.4299999999999997, -1.4299999999999997, -0.7049999999999996, -0.20499999999999963, 0.4116666666666669, 0.6283333333333336, -0.08833333333333304, -0.20499999999999968, -0.2549999999999997, -0.9549999999999997, -0.3216666666666664, 0.48666666666666697, 0.7783333333333335, 1.3283333333333336, 1.5450000000000004, 1.286666666666667, 0.7116666666666671, 0.5200000000000004, -0.5216666666666663, -0.5299999999999996, 0.4950000000000003, 0.4700000000000003, -0.029999999999999694, -1.1216666666666664, -1.7466666666666664, -1.513333333333333, -1.1799999999999997, -0.4299999999999997, 0.6700000000000004, -0.6466666666666663, -0.21333333333333288, -0.6549999999999996, -1.4549999999999996, -0.6299999999999997, -1.6466666666666663, -1.4549999999999996, -1.2966666666666664, -0.8216666666666663, -0.12166666666666637, -0.12999999999999967, -0.6133333333333331, -1.4549999999999996, -1.113333333333333, -0.9049999999999997, -0.40499999999999975, 0.19500000000000028, -0.10499999999999976, -0.1216666666666664, -0.4299999999999997, -1.0549999999999997, -1.6716666666666664, -1.438333333333333, -1.4049999999999998, -1.288333333333333, 0.086666666666667, -0.05499999999999966, 0.07000000000000031, 0.11166666666666691, -0.30499999999999977, -0.6133333333333331, 0.011666666666667047, -0.19666666666666643, -0.21333333333333304, 0.08666666666666695, -1.0799999999999998, -0.6966666666666663, -1.0883333333333332, -0.9049999999999997, 0.2366666666666669, 0.20333333333333364, 0.136666666666667, -0.5216666666666664, -1.3299999999999998, -0.4966666666666665, -0.14666666666666645, 0.3700000000000002, 0.6116666666666669, 0.06166666666666694, 0.8950000000000002, 0.5200000000000002, 0.411666666666667, 1.0283333333333335, 0.6366666666666669, 1.4950000000000003, 0.9200000000000004, 0.028333333333333655, -1.1716666666666664, -1.3883333333333332, -1.0299999999999998, -0.813333333333333, 0.10333333333333361, -0.6716666666666664, -0.4049999999999997, -0.21333333333333307, -0.07166666666666635, -0.07166666666666638, -0.9716666666666665, -1.0216666666666663, -1.0966666666666665, -0.2966666666666664, 0.911666666666667, 1.5283333333333338, 0.9033333333333337, 0.22000000000000033, -0.5049999999999997, -1.0466666666666664, -0.15499999999999964, 0.04500000000000026, -0.13833333333333303, 0.036666666666666986, -0.8966666666666664, 0.24500000000000033, 0.35333333333333367, -0.488333333333333, 0.25333333333333363, -0.6049999999999998, -0.22166666666666646, 0.311666666666667, 0.6033333333333336, 0.49500000000000033, 0.28666666666666696, 0.003333333333333688, 0.21166666666666695, -0.0633333333333331, 0.6950000000000003, 0.40333333333333354, -0.0633333333333331, -0.08833333333333307, -0.1549999999999998, 0.936666666666667, 0.8033333333333337, 0.8616666666666669, 0.48666666666666697, 0.13666666666666694, -0.12999999999999973, 0.4450000000000003, 0.811666666666667, 0.7950000000000003, 1.5200000000000002, 0.5700000000000003, 0.1450000000000003, -0.09666666666666633, 0.4450000000000005, 1.2450000000000006, 1.0783333333333338, 1.2783333333333338, 0.2783333333333336, -0.2716666666666664, 0.04500000000000032, -0.7133333333333329, -0.23833333333333295, -0.313333333333333, -0.07999999999999968, 0.8866666666666669, -0.22166666666666635, 0.12000000000000033, 0.36166666666666697, 0.37833333333333363, 1.1783333333333337, 0.9616666666666669, -0.17999999999999977, -0.12166666666666637, -0.5716666666666663, -0.0966666666666664, 0.686666666666667, 0.2783333333333336, -0.3966666666666664, -0.1549999999999997, -0.2549999999999997, 0.47000000000000025, 1.2783333333333338, 0.3950000000000002, -0.05499999999999977, -0.5299999999999997, -0.7216666666666663, -0.4799999999999997, 0.24500000000000027, 0.02833333333333364, 0.5700000000000003, 0.17833333333333368, -0.20499999999999968, -0.2299999999999997, -1.5716666666666663, -0.8466666666666663, -1.4466666666666663, -1.3966666666666663, 0.086666666666667, -0.17166666666666633, -0.7133333333333329, -1.0716666666666663, -1.738333333333333, -1.8049999999999997, -0.6299999999999997, -0.3966666666666664, 0.6783333333333337, 0.9783333333333336, 0.7533333333333336, 0.9533333333333336, 0.16166666666666696, -0.838333333333333, -0.5466666666666664, -0.688333333333333, -1.463333333333333, -0.37166666666666637, -0.438333333333333, 0.561666666666667, 1.286666666666667, 1.186666666666667, 1.1450000000000005, 0.5116666666666669, 0.6116666666666669, 0.7700000000000002, -0.17999999999999983, -0.3799999999999998, -0.4633333333333331, -0.5049999999999997, -0.06333333333333308, -0.3133333333333331, -0.5216666666666664, -0.45499999999999974, 0.07833333333333364, 0.8783333333333336, 0.2950000000000004, -0.1716666666666663, -1.0299999999999998, -1.8299999999999996, -1.3633333333333328, -1.2299999999999995, -0.6383333333333331, 0.18666666666666687, 0.29500000000000026, 0.2533333333333336, 0.686666666666667, 0.2200000000000003, 0.261666666666667, 0.8700000000000003, 0.9783333333333337, 1.1950000000000003, 1.0033333333333336, 0.8033333333333337, 0.9616666666666669, 0.3700000000000003, 0.6366666666666669, -0.22999999999999976, -0.8799999999999997, -0.5049999999999997, -0.2716666666666664, 0.03666666666666696, -0.15499999999999975, -0.5799999999999997, -0.6549999999999996, -0.6799999999999997, -0.021666666666666334, 0.04500000000000029, -0.12166666666666638, 0.17833333333333362, -0.4216666666666664, -0.7966666666666664, 0.028333333333333655, -0.029999999999999694, 1.3783333333333339, 1.6200000000000003, 0.3533333333333337, -0.15499999999999964, -2.03, -1.638333333333333, -1.338333333333333, -0.5216666666666665, 0.38666666666666694, 0.5866666666666669, 1.0950000000000004, 0.38666666666666694, -0.413333333333333, -1.3966666666666665, -1.3799999999999997, -0.9883333333333331, 0.12000000000000027, 0.3033333333333337, 0.0033333333333336115, -0.0549999999999997, -0.49666666666666637, 0.6116666666666669, 0.5283333333333335, 0.5950000000000002, 0.8616666666666668, 0.5450000000000003, 1.2366666666666668, 1.07, 0.8200000000000003, 0.6700000000000004, 0.3200000000000003, 0.7866666666666668, -0.12166666666666637, -0.48833333333333306, -0.6299999999999997, -1.5216666666666665, 0.16166666666666696, 0.5533333333333337, 0.6783333333333337, 0.39500000000000024, -0.6133333333333331, -0.6716666666666664, -0.8299999999999996, -0.37999999999999967, -0.004999999999999699, -0.13833333333333303, 0.2950000000000003, 0.36166666666666697, -0.14666666666666633, -0.4049999999999997, -1.5883333333333332, -1.6049999999999998, -1.1049999999999998, -1.1216666666666664, -0.4299999999999997, 0.2283333333333336, -0.1466666666666664, 0.5533333333333337, -0.07166666666666632, 0.18666666666666698, -0.05499999999999966, -0.688333333333333, 0.12000000000000027, -0.2716666666666664, 0.10333333333333361, 0.12833333333333358, -0.313333333333333, -0.06333333333333291, 0.8283333333333337, 0.5033333333333337, 1.561666666666667, 1.311666666666667, 0.3283333333333336, 1.2533333333333336, 0.6450000000000002, 0.2783333333333336, 0.7116666666666669, 0.9450000000000003, 0.2533333333333336, 0.6533333333333335, -0.12999999999999973, -1.0716666666666663, -0.29666666666666636, -0.813333333333333, -0.663333333333333, -0.513333333333333, -0.9549999999999997, -0.688333333333333, -0.26333333333333303, 0.9533333333333336, 2.0533333333333337, 1.82, 0.9450000000000002, 0.13666666666666702, 0.14500000000000046, -0.4549999999999996, 0.6366666666666669, -0.39666666666666633, -0.9883333333333332, -0.6966666666666663, -1.238333333333333, -0.22166666666666632, -0.688333333333333, 0.19500000000000034, 0.29500000000000026, 0.07833333333333364, 0.311666666666667, 0.4700000000000003, 0.836666666666667, 0.7533333333333336, -0.029999999999999694, 0.27833333333333365, 0.311666666666667, -0.813333333333333]
  out "CH1  Bin Readings":dbl[](array[numeric])=[148.0, 153.0, 135.0, 116.0, 121.0, 144.0, 150.0, 143.0, 133.0, 138.0, 147.0, 165.0, 184.0, 140.0, 155.0, 172.0, 165.0, 181.0, 175.0, 175.0, 218.0, 180.0, 185.0, 202.0, 201.0, 210.0, 211.0, 218.0, 208.0, 220.0, 211.0, 227.0, 219.0, 210.0, 230.0, 235.0, 226.0, 244.0, 217.0, 237.0, 220.0, 222.0, 182.0, 205.0, 200.0, 232.0, 221.0, 212.0, 233.0, 234.0, 231.0, 203.0, 190.0, 195.0, 196.0, 182.0, 165.0, 176.0, 157.0, 177.0, 166.0, 168.0, 177.0, 156.0, 178.0, 145.0, 160.0, 138.0, 164.0, 179.0, 138.0, 153.0, 195.0, 166.0, 158.0, 146.0, 149.0, 151.0, 193.0, 150.0, 140.0, 157.0, 132.0, 122.0, 154.0, 118.0, 127.0, 99.0, 117.0, 125.0, 138.0, 121.0, 105.0, 93.0, 96.0, 103.0, 99.0, 95.0, 123.0, 96.0, 91.0, 87.0, 99.0, 122.0, 93.0, 98.0, 84.0, 100.0, 101.0, 124.0, 105.0, 124.0, 146.0, 234.0, 330.0, 442.0, 581.0, 689.0, 1016.0, 1248.0, 1618.0, 2114.0, 2643.0, 3190.0, 3666.0, 3862.0, 3731.0, 3523.0, 3177.0, 3041.0, 2723.0, 2565.0, 2310.0, 1914.0, 1488.0, 1233.0, 1018.0, 878.0, 734.0, 670.0, 530.0, 507.0, 522.0, 560.0, 579.0, 526.0, 501.0, 509.0, 435.0, 390.0, 329.0, 295.0, 306.0, 345.0, 342.0, 338.0, 352.0, 268.0, 227.0, 210.0, 190.0, 178.0, 151.0, 127.0, 119.0, 80.0, 92.0, 81.0, 78.0, 85.0, 72.0, 85.0, 94.0, 81.0, 73.0, 66.0, 77.0, 74.0, 73.0, 70.0, 90.0, 77.0, 72.0, 82.0, 63.0, 90.0, 88.0, 89.0, 96.0, 72.0, 79.0, 102.0, 81.0, 82.0, 93.0, 88.0, 77.0, 78.0, 90.0, 79.0, 73.0, 90.0, 85.0, 69.0, 83.0, 93.0, 90.0, 81.0, 82.0, 84.0, 69.0, 87.0, 57.0, 63.0, 78.0, 76.0, 86.0, 90.0, 71.0, 77.0, 75.0, 83.0, 70.0, 76.0, 77.0, 81.0, 79.0, 97.0, 73.0, 80.0, 102.0, 83.0, 90.0, 81.0, 100.0, 92.0, 73.0, 97.0, 84.0, 77.0, 82.0, 84.0, 80.0, 79.0, 81.0, 95.0, 71.0, 97.0, 64.0, 61.0, 63.0, 81.0, 85.0, 82.0, 76.0, 82.0, 72.0, 88.0, 76.0, 74.0, 79.0, 80.0, 86.0, 74.0, 85.0, 74.0, 104.0, 89.0, 83.0, 86.0, 79.0, 86.0, 78.0, 83.0, 82.0, 77.0, 83.0, 79.0, 88.0, 89.0, 68.0, 83.0, 84.0, 92.0, 71.0, 82.0, 84.0, 70.0, 77.0, 83.0, 86.0, 76.0, 70.0, 96.0, 70.0, 71.0, 85.0, 59.0, 91.0, 74.0, 67.0, 100.0, 78.0, 53.0, 89.0, 91.0, 102.0, 76.0, 88.0, 83.0, 80.0, 74.0, 89.0, 84.0, 103.0, 79.0, 69.0, 70.0, 74.0, 100.0, 100.0, 81.0, 92.0, 76.0, 84.0, 86.0, 80.0, 83.0, 75.0, 73.0, 77.0, 78.0, 73.0, 77.0, 88.0, 81.0, 75.0, 81.0, 88.0, 90.0, 86.0, 83.0, 73.0, 77.0, 87.0, 88.0, 84.0, 97.0, 83.0, 76.0, 85.0, 86.0, 94.0, 80.0, 71.0, 69.0, 97.0, 84.0, 98.0, 90.0, 84.0, 75.0, 72.0, 79.0, 80.0, 69.0, 85.0, 70.0, 77.0, 77.0, 77.0, 72.0, 76.0, 82.0, 63.0, 79.0, 79.0, 88.0, 58.0, 88.0, 90.0, 87.0, 75.0, 76.0, 86.0, 81.0, 87.0, 95.0, 76.0, 82.0, 82.0, 84.0, 82.0, 77.0, 81.0, 89.0, 80.0, 81.0, 91.0, 86.0, 92.0, 83.0, 72.0, 75.0, 74.0, 74.0, 68.0, 71.0, 89.0, 85.0, 90.0, 75.0, 84.0, 78.0, 85.0, 78.0, 93.0, 85.0, 73.0, 96.0, 75.0, 78.0, 87.0, 80.0, 73.0, 76.0, 99.0, 84.0, 64.0, 93.0, 90.0, 90.0, 83.0, 64.0, 85.0, 83.0, 94.0, 78.0, 82.0, 83.0, 76.0, 83.0, 83.0, 81.0, 107.0, 91.0, 83.0, 78.0, 89.0, 86.0, 91.0, 84.0, 89.0, 94.0, 74.0, 78.0, 65.0, 88.0, 83.0, 95.0, 88.0, 87.0, 87.0, 88.0, 80.0, 86.0, 98.0, 70.0, 78.0, 70.0, 90.0, 75.0, 90.0, 83.0, 92.0, 87.0, 78.0, 76.0, 86.0, 95.0, 82.0, 73.0, 80.0, 63.0, 77.0, 93.0, 74.0, 88.0, 95.0, 70.0, 81.0, 64.0, 81.0, 95.0, 81.0, 92.0, 82.0, 81.0, 74.0, 87.0, 75.0, 82.0, 87.0, 96.0, 80.0, 70.0, 94.0, 89.0, 75.0, 78.0, 70.0, 86.0, 107.0, 100.0, 86.0, 82.0, 106.0, 78.0, 74.0, 75.0, 61.0, 82.0, 88.0, 68.0, 87.0, 90.0, 90.0, 80.0, 68.0, 97.0, 73.0, 81.0, 64.0, 72.0, 70.0, 85.0, 83.0, 84.0, 80.0, 80.0, 76.0, 85.0, 83.0, 71.0, 83.0, 93.0, 83.0, 81.0, 72.0, 98.0, 87.0, 86.0, 94.0, 77.0, 83.0, 78.0, 70.0, 58.0, 77.0]
  out "CH1 (WV off) smooth S":dbl[](array[numeric])=[57.43644444444443, 54.665611111111104, 55.3406111111111, 58.097555555555545, 60.376722222222206, 63.398944444444425, 65.19755555555554, 67.00172222222218, 69.67672222222218, 71.92811111111106, 75.61283333333327, 80.0336666666666, 84.04755555555549, 89.10172222222215, 94.99477777777773, 100.65033333333328, 107.3267222222222, 114.08922222222219, 120.31561111111108, 126.40172222222219, 132.1989444444444, 136.7003333333333, 141.43505555555552, 146.0739444444444, 150.65727777777772, 156.27811111111106, 161.59338888888885, 166.87255555555552, 171.2058888888889, 174.58505555555553, 177.48366666666666, 178.0656111111111, 178.33366666666666, 177.38088888888888, 174.92811111111112, 171.817, 167.0503333333333, 161.18783333333332, 154.7989444444444, 149.0100555555555, 143.60866666666664, 139.55588888888886, 137.53366666666665, 136.18644444444442, 135.38505555555554, 133.8989444444444, 130.29199999999997, 125.91561111111108, 118.78922222222221, 110.77116666666663, 103.24616666666661, 96.00033333333327, 91.34477777777771, 87.68783333333326, 84.34477777777772, 81.99199999999995, 79.98783333333328, 78.3739444444444, 76.93922222222218, 75.35449999999996, 74.03088888888885, 73.16005555555552, 72.08505555555553, 71.1767222222222, 70.39338888888886, 69.79755555555553, 69.72672222222221, 69.28644444444441, 68.61283333333331, 68.21977777777775, 67.99477777777776, 67.6267222222222, 66.47533333333331, 65.19338888888886, 62.828111111111085, 59.29061111111109, 56.003111111111096, 51.33088888888888, 46.698944444444436, 43.36144444444445, 39.93644444444445, 37.519777777777776, 35.57116666666667, 33.66977777777778, 32.20311111111111, 31.053111111111114, 29.153111111111116, 28.62116666666667, 27.88088888888889, 27.082277777777776, 27.50727777777778, 26.529500000000002, 25.928111111111114, 25.32394444444445, 24.61283333333334, 24.4183888888889, 23.844777777777786, 23.04616666666667, 21.84894444444445, 20.45727777777778, 19.28227777777778, 17.962833333333332, 17.685055555555554, 17.329499999999996, 17.668388888888888, 17.858666666666664, 18.076722222222223, 18.617, 18.755888888888887, 20.119777777777777, 21.84477777777778, 25.26005555555556, 31.992, 41.31838888888887, 55.27672222222216, 74.3336666666666, 100.13783333333328, 134.7267222222222, 176.7378333333334, 225.52950000000016, 278.8850555555557, 335.30866666666685, 395.9781111111113, 461.86422222222234, 539.2447777777778, 643.1392222222222, 793.3628333333331, 1016.9225555555552, 1320.1767222222215, 1681.1128333333327, 2058.282277777777, 2387.766999999999, 2618.658666666666, 2716.333666666666, 2665.70311111111, 2489.1600555555547, 2225.401722222221, 1927.2156111111099, 1647.4378333333327, 1416.1683888888883, 1242.1697777777774, 1120.6045, 1030.7933888888886, 956.0572777777777, 884.553111111111, 807.6919999999999, 729.0322777777776, 647.3961666666667, 565.7850555555556, 487.817, 414.90727777777784, 351.5253333333335, 297.8836666666668, 253.443388888889, 216.57672222222223, 184.8128333333333, 157.2364444444444, 132.98088888888884, 110.5531111111111, 90.46005555555554, 72.71005555555556, 57.14616666666666, 45.14616666666666, 34.964222222222226, 26.70033333333333, 19.96977777777778, 14.597555555555553, 10.679499999999999, 7.507277777777779, 5.265611111111112, 3.8322777777777786, 2.4433888888888897, 1.7475555555555558, 1.368388888888889, 0.7392222222222224, 0.4795000000000001, 0.023944444444444574, -0.08855555555555547, -0.11216666666666658, -0.14688888888888882, -0.05661111111111103, -0.41355555555555545, -0.3649444444444443, -0.19272222222222213, -0.07744444444444433, -0.29827777777777764, -0.481611111111111, -0.5121666666666665, -0.5010555555555555, -0.23855555555555535, -0.5093888888888887, -0.4329999999999999, -0.5454999999999998, -0.2774444444444444, 0.28227777777777785, 0.10450000000000005, -0.12327777777777782, -0.2455, -0.5913333333333333, -0.7038333333333332, -0.25244444444444436, -0.369111111111111, -0.19827777777777778, -0.47883333333333333, -0.8774444444444445, -0.9107777777777777, -1.1843888888888887, -0.7857777777777776, -0.45799999999999974, -0.23994444444444432, -0.3454999999999999, -0.0746666666666666, -0.14966666666666667, -0.3941111111111111, -0.16911111111111093, -0.4024444444444442, -0.4496666666666664, -0.10244444444444423, -0.119111111111111, 0.08922222222222238, 0.2392222222222224, -0.05661111111111096, -0.032999999999999696, -0.23299999999999974, -0.5371666666666665, -0.18299999999999966, 0.09755555555555573, 0.21561111111111125, 0.532277777777778, 0.45311111111111124, -0.10661111111111088, -0.6177222222222221, -0.5982777777777776, -0.7968888888888888, -0.29827777777777775, 0.19616666666666677, 0.20588888888888898, 0.255888888888889, 0.47811111111111115, 0.48227777777777786, 0.5322777777777778, 0.5003333333333334, -0.045499999999999874, 0.10450000000000012, 0.06700000000000014, -0.4121666666666666, -0.433, -1.0024444444444442, -1.3691111111111112, -0.7329999999999998, -0.6399444444444442, -0.34272222222222204, -0.2899444444444443, -0.3468888888888887, -0.09133333333333338, -0.2607777777777779, -0.2302222222222223, -0.4621666666666667, -0.7538333333333332, -0.6246666666666665, -0.5621666666666666, -0.42188888888888876, -0.2732777777777776, -0.25522222222222213, 0.1128333333333334, -0.01911111111111105, -0.023277777777777717, 0.04616666666666668, -0.14133333333333326, -0.17188888888888887, -0.12188888888888885, -0.056611111111111015, -0.5746666666666667, -0.5107777777777777, -0.32744444444444426, -0.5010555555555554, -0.29272222222222205, -0.24549999999999988, -0.5927222222222222, -0.5579999999999999, -0.5843888888888887, -0.32188888888888867, 0.11977777777777796, 0.26561111111111124, 0.2989444444444445, 0.0572777777777778, -0.43716666666666665, -0.358, -0.1649444444444444, -0.27049999999999996, -0.11216666666666662, -0.4343888888888888, -0.2510555555555555, 0.0058888888888889435, -0.1955, -0.2080000000000001, -0.38994444444444454, -0.24550000000000002, -0.2441111111111111, 0.030888888888888938, -0.29966666666666664, -0.5774444444444444, -0.33022222222222225, -0.3496666666666667, 0.008666666666666704, 0.20866666666666672, -0.26355555555555527, -0.08994444444444416, -0.19411111111111085, -0.039944444444444116, 0.4836666666666668, 0.008666666666666822, -0.17049999999999987, -0.30799999999999994, -0.2899444444444444, -0.255222222222222, -0.105222222222222, -0.38577777777777755, -0.5010555555555554, -0.17466666666666655, -0.17744444444444432, 0.1753333333333334, -0.042722222222222134, 0.05450000000000005, 0.08088888888888893, -0.14966666666666661, 0.09200000000000005, -0.08299999999999991, -0.20938888888888865, -0.3066111111111109, -0.3468888888888887, -0.14549999999999985, 0.42533333333333334, 0.3864444444444446, 0.7503333333333335, 0.5281111111111113, -0.09827777777777758, 0.3864444444444446, -0.13299999999999987, -0.2510555555555555, 0.07394444444444453, -0.29827777777777775, 0.1558888888888889, 0.22116666666666673, 0.14061111111111116, -0.041333333333333305, -0.030222222222222123, -0.19133333333333322, 0.0656111111111112, 0.3350555555555557, -0.06633333333333326, 0.02533333333333343, -0.48022222222222216, -0.5218888888888888, -0.3954999999999999, -0.1913333333333333, -0.03161111111111099, -0.056611111111111, 0.06422222222222233, -0.28161111111111103, -0.1482777777777777, -0.3871666666666665, -0.9510555555555554, -1.0149444444444442, -1.1843888888888885, -0.8593888888888886, -0.29549999999999965, 0.2961666666666669, 0.8836666666666668, 0.4586666666666669, 0.2489444444444446, -0.29688888888888876, -0.8288333333333332, -0.5913333333333333, -0.5163333333333333, -0.46633333333333327, -0.3760555555555554, -0.49827777777777765, -0.3371666666666666, -0.05938888888888881, -0.4093888888888887, -0.1843888888888887, -0.7357777777777776, -1.0843888888888886, -0.7302222222222222, -0.5579999999999999, 0.11005555555555557, 0.24616666666666673, 0.2642222222222223, 0.08227777777777787, -0.22466666666666657, -0.09827777777777766, -0.20383333333333323, -0.17744444444444438, -0.42466666666666675, -0.421888888888889, -0.11216666666666675, 0.13227777777777772, 0.530888888888889, 0.32811111111111124, 0.04061111111111129, -0.29688888888888876, -0.23299999999999982, -0.21911111111111098, -0.28994444444444434, -0.6996666666666667, -0.6746666666666666, -0.8482777777777777, -0.8468888888888888, -0.30661111111111106, -0.3843888888888889, -0.2649444444444444, 0.1864444444444444, 0.20866666666666672, 0.330888888888889, 0.4933888888888891, 0.1614444444444447, 0.12255555555555571, -0.08577777777777768, -0.2857777777777778, -0.09272222222222223, -0.06494444444444446, -0.06633333333333334, 0.40033333333333343, 0.03783333333333344, -0.5468888888888888, -0.6413333333333331, -0.8371666666666665, -0.7427222222222221, -0.2038333333333333, 0.003111111111111245, 0.11422222222222235, 0.1892222222222224, 0.10588888888888906, -0.23022222222222216, -0.31633333333333324, -0.14688888888888868, -0.42188888888888865, -0.26216666666666644, -0.3482777777777775, -0.48022222222222205, 0.14477777777777792, 0.27811111111111125, 0.26422222222222247, 0.11561111111111133, -0.3913333333333332, -0.43994444444444436, -0.5288333333333333, 0.01144444444444448, 0.5475555555555556, 0.7156111111111112, 1.0378333333333334, 0.7072777777777778, 0.0892222222222222, -0.28994444444444445, -0.4538333333333333, -0.4718888888888889, 0.028111111111111003, 0.11005555555555552, -0.05800000000000008, 0.15172222222222223, -0.18299999999999977, -0.13022222222222207, -0.044111111111111004, -0.48716666666666664, -0.5899444444444444, -0.4538333333333332, -0.0010555555555554208, 0.11005555555555568, 0.49616666666666676, 0.13088888888888905, -0.18299999999999983, -0.5454999999999999, -0.7649444444444443, -0.37049999999999994, -0.5510555555555554, -0.3774444444444443, -0.16355555555555543, -0.14966666666666653, -0.01772222222222214, 0.26422222222222236, 0.10172222222222234, -0.08994444444444433, -0.07327777777777768, 0.05311111111111129, -0.003833333333333161, 0.12672222222222237, 0.15172222222222237, -0.04272222222222211, 0.018388888888889, -0.1552222222222221, -0.3135555555555554, -0.2454999999999999, -0.244111111111111, -0.17744444444444435, -0.09827777777777769, -0.21633333333333324, -0.08161111111111105, -0.0746666666666666, -0.1371666666666666, 0.00033333333333326887, -0.49549999999999994, -0.4052222222222222, -0.4802222222222221, -0.42605555555555535, -0.18855555555555537, -0.4010555555555554, -0.4635555555555554, -0.6663333333333332, -0.4260555555555555, -0.07744444444444443, 0.0920000000000001, 0.2961666666666669, 0.2670000000000002, 0.23644444444444473, 0.17950000000000033, -0.049666666666666456, 0.028111111111111323, -0.2649444444444442, -0.3274444444444443, -0.131611111111111, -0.33716666666666667, -0.3941111111111111, -0.14688888888888887, -0.020500000000000018, -0.34133333333333316, -0.09549999999999978, -0.2829999999999997, -0.4607777777777774, 0.08922222222222248, 0.2045000000000003, 0.4295000000000002, 0.47672222222222244, 0.0572777777777779, -0.06772222222222213, -0.1496666666666666, -0.319111111111111, 0.10311111111111121, -0.10522222222222215, -0.3663333333333333, -0.19411111111111098, -0.2552222222222221, -0.06355555555555534, 0.15311111111111136, 0.2725555555555558, 0.47533333333333355, 0.5517222222222224, 0.8420000000000003, 0.40033333333333354, 0.34061111111111136, 0.18088888888888913, -0.2996666666666664, -0.06077777777777764, -0.5982777777777777, -0.7607777777777778]
  out "CH0 (WV on) smoothed":dbl[](array[numeric])=[40.85315789473683, 35.78736842105262, 34.839999999999996, 33.168947368421044, 30.695263157894736, 30.80052631578947, 29.45842105263157, 31.61631578947368, 33.024210526315784, 34.774210526315784, 36.16894736842105, 35.51105263157895, 36.60315789473684, 36.40578947368421, 37.30052631578947, 38.10315789473684, 38.774210526315784, 41.668947368421044, 43.35315789473684, 44.98473684210526, 46.524210526315784, 45.11631578947368, 44.15578947368421, 43.65578947368421, 42.45842105263158, 42.94526315789473, 44.4978947368421, 45.616315789473674, 47.07684210526315, 48.95842105263158, 49.37947368421052, 49.35315789473683, 50.24789473684209, 47.68210526315789, 46.80052631578946, 47.64263157894736, 46.26105263157894, 46.33999999999999, 45.48473684210526, 41.76105263157894, 37.642631578947366, 36.85315789473684, 34.682105263157894, 34.866315789473674, 37.339999999999996, 36.20842105263158, 35.73473684210526, 34.524210526315784, 31.287368421052626, 27.589999999999996, 25.484736842105264, 22.958421052631575, 20.997894736842103, 20.642631578947366, 20.800526315789472, 21.576842105263154, 21.747894736842103, 21.31368421052631, 19.392631578947366, 17.66894736842105, 16.45842105263158, 16.418947368421048, 15.695263157894734, 15.05052631578947, 15.879473684210524, 14.629473684210526, 14.221578947368421, 14.34, 13.826842105263157, 13.682105263157894, 14.234736842105262, 13.747894736842106, 12.866315789473685, 12.721578947368421, 13.024210526315787, 12.98473684210526, 11.813684210526313, 10.945263157894734, 8.747894736842104, 7.392631578947367, 5.800526315789473, 5.747894736842105, 5.695263157894736, 5.09, 5.550526315789474, 4.484736842105263, 4.024210526315789, 3.1294736842105264, 3.142631578947368, 2.511052631578947, 3.6426315789473684, 3.761052631578947, 3.221578947368421, 3.234736842105263, 0.06368421052631557, -0.7126315789473687, -0.6600000000000004, -0.6731578947368425, 1.6689473684210523, 1.5110526315789472, 2.3005263157894733, 2.603157894736842, 2.392631578947368, 3.3399999999999994, 2.2873684210526313, 2.9321052631578945, 1.4321052631578943, 2.1821052631578945, 3.445263157894737, 4.9321052631578945, 8.813684210526315, 13.247894736842103, 20.945263157894736, 31.353157894736842, 47.971578947368414, 70.8136842105263, 99.41894736842104, 133.16894736842104, 169.37947368421052, 205.2084210526316, 242.56368421052633, 279.761052631579, 315.24789473684217, 344.8136842105264, 363.68210526315795, 369.70842105263165, 361.90578947368425, 348.4584210526316, 330.3005263157895, 314.0242105263158, 295.7478947368421, 276.4978947368421, 252.33999999999997, 224.74789473684208, 197.2215789473684, 169.4978947368421, 146.62947368421052, 124.30052631578947, 106.9057894736842, 93.57684210526315, 84.76105263157895, 82.09, 83.23473684210526, 84.36631578947367, 86.48473684210526, 85.56368421052632, 83.4321052631579, 81.10315789473685, 76.16894736842106, 72.30052631578948, 65.69526315789474, 58.03736842105263, 50.72157894736842, 44.11631578947369, 40.142631578947366, 37.721578947368414, 34.45842105263157, 30.20842105263157, 25.9978947368421, 21.537368421052626, 18.30052631578947, 14.366315789473683, 11.392631578947366, 8.85315789473684, 8.142631578947366, 7.721578947368419, 5.892631578947367, 4.800526315789472, 1.3005263157894733, 0.5505263157894735, 1.2084210526315788, -0.0021052631578949432, 1.3005263157894733, 0.3531578947368418, -0.9757894736842108, -0.05473684210526347, -1.515263157894737, -0.7915789473684213, -0.2521052631578949, -0.17315789473684223, 0.08999999999999964, -0.054736842105263445, -1.2257894736842108, -1.502105263157895, -1.0415789473684214, -0.8047368421052636, 0.31368421052631545, -0.2652631578947372, 0.6689473684210523, 0.08999999999999969, -0.3573684210526319, 0.6294736842105261, -0.08105263157894763, -0.06789473684210559, -0.6205263157894739, -0.8968421052631583, -1.1468421052631583, -0.8442105263157899, 0.2347368421052628, -1.0678947368421057, -0.3968421052631582, -1.2784210526315793, -0.6994736842105267, -0.10736842105263195, -1.6994736842105267, -1.581052631578948, -3.107368421052632, -2.84421052631579, -0.988947368421053, -0.6863157894736845, 0.16894736842105232, 0.2873684210526313, -0.752105263157895, 0.011052631578947092, 0.08999999999999975, 0.35315789473684184, 0.5110526315789471, 1.5110526315789472, 1.4584210526315786, 0.9978947368421048, 1.3399999999999999, 0.4057894736842102, -0.16000000000000034, -0.08105263157894771, -0.8968421052631583, -1.3178947368421057, -0.22578947368421087, -0.10736842105263192, -0.2389473684210529, -0.3705263157894739, -1.1600000000000004, -2.0152631578947373, -1.7521052631578948, -2.0415789473684214, -2.1994736842105267, -1.5284210526315791, -0.6994736842105267, -0.3836842105263161, 0.08999999999999969, 0.26105263157894704, -0.7915789473684214, -0.6994736842105267, -1.1863157894736847, -2.554736842105264, -1.765263157894737, -1.475789473684211, -0.988947368421053, -0.31789473684210556, 0.8399999999999996, 1.5373684210526313, 1.3136842105263156, 1.7478947368421052, -0.5152631578947373, -1.9231578947368426, -1.5810526315789477, -0.5810526315789478, 0.3531578947368416, -0.3178947368421057, -1.1600000000000004, -2.2126315789473687, -2.673157894736842, -1.9231578947368424, -2.4757894736842108, -2.081052631578948, -0.7784210526315793, -0.8178947368421056, -0.12052631578947404, 0.7084210526315786, 0.5636842105263155, 1.5373684210526313, 0.5242105263157892, -0.13368421052631607, -1.396842105263158, -1.252105263157895, -1.146842105263158, -1.9363157894736847, -1.5678947368421057, -1.9100000000000004, -0.8968421052631582, -0.9231578947368424, -0.870526315789474, -1.8178947368421057, -2.6994736842105267, -1.7915789473684216, -1.817894736842106, -1.081052631578948, 0.22157894736842065, -0.502105263157895, 0.379473684210526, -0.26526315789473714, -0.10736842105263189, -0.13368421052631613, -0.7784210526315792, -0.6336842105263161, -1.646842105263158, -0.27842105263157935, -0.9363157894736847, -0.13368421052631624, -0.9494736842105267, -1.370526315789474, -0.5678947368421055, -1.6073684210526318, -0.9231578947368424, -1.4494736842105267, -1.2126315789473687, -1.2652631578947373, -1.2126315789473687, -1.0415789473684214, -1.4363157894736847, -1.9494736842105267, -1.7126315789473687, -2.857368421052632, -3.0284210526315793, -1.370526315789474, -1.9626315789473687, -0.8178947368421056, -0.8047368421052634, -1.5678947368421055, -0.620526315789474, -0.8178947368421057, -0.4626315789473688, -0.738947368421053, -0.7652631578947372, -0.7784210526315792, -2.09421052631579, -2.304736842105264, -3.0284210526315793, -3.41, -2.581052631578948, -2.6731578947368426, -0.8178947368421057, -0.8836842105263161, -0.988947368421053, -0.5284210526315792, -0.8836842105263162, -0.5021052631578949, 1.9321052631578945, 2.1689473684210525, 1.8663157894736842, 1.4189473684210525, -0.22578947368421087, -0.7257894736842109, -2.4757894736842108, -2.4100000000000006, -2.5942105263157895, -1.9231578947368424, -1.7126315789473687, -1.738947368421053, -2.1731578947368426, -1.5415789473684214, -0.4626315789473688, -0.6994736842105267, -0.8573684210526319, -1.6994736842105267, -2.0152631578947373, -0.8310526315789477, 0.6557894736842103, 0.49789473684210495, 0.7478947368421048, -0.988947368421053, -2.3968421052631586, -1.6073684210526318, -1.0942105263157897, 0.9057894736842103, 1.392631578947368, 0.7873684210526313, -0.22578947368421087, -0.48894736842105296, -1.120526315789474, -1.502105263157895, -1.1863157894736847, -2.4363157894736847, -2.0021052631578953, -1.5810526315789477, -2.2389473684210532, -1.3968421052631583, -1.581052631578948, -0.8047368421052636, 0.11631578947368387, -0.041578947368421396, 0.3005263157894734, -0.6468421052631581, -0.6468421052631582, -0.8047368421052634, -1.7126315789473687, -0.4626315789473687, -0.9494736842105267, -1.4889473684210528, -1.1994736842105267, -1.962631578947369, -1.1600000000000004, 0.1689473684210523, 1.1689473684210523, 0.8268421052631575, 0.11631578947368382, -1.1731578947368424, -1.870526315789474, -1.3178947368421055, -1.0810526315789477, -0.015263157894737145, 0.5505263157894734, 0.1689473684210523, 0.18210526315789438, -0.5810526315789477, -1.015263157894737, -1.396842105263158, -0.7652631578947373, -0.6731578947368424, -0.5810526315789477, -0.43631578947368455, -1.146842105263158, -0.5415789473684213, 0.06368421052631545, -0.5415789473684214, -0.1468421052631582, -0.5547368421052635, -1.5152631578947373, -0.3442105263157898, 0.0768421052631576, -0.6336842105263161, -0.8178947368421056, -1.252105263157895, -1.857368421052632, -1.107368421052632, -0.9100000000000004, -1.4626315789473687, -1.6994736842105267, -2.120526315789474, -2.4757894736842108, -2.633684210526316, -2.5152631578947373, -2.2521052631578953, -1.883684210526316, -0.8705263157894741, -0.06789473684210567, -0.27842105263157935, 0.524210526315789, 0.5505263157894733, -0.3178947368421057, -0.8968421052631581, -1.252105263157895, -0.3310526315789477, -0.4626315789473688, 0.4715789473684207, -0.5152631578947371, -1.515263157894737, -1.1600000000000004, -1.6863157894736847, -1.2389473684210528, -2.146842105263158, -1.5678947368421057, -1.002105263157895, 0.35315789473684184, 0.4847368421052628, -0.6468421052631582, -0.6336842105263161, -1.4626315789473687, -1.107368421052632, -0.5942105263157899, -1.633684210526316, -2.002105263157895, -2.107368421052632, -1.9494736842105267, -1.5547368421052634, -1.4100000000000006, -0.8968421052631581, -0.9363157894736844, -1.1863157894736847, -1.265263157894737, -2.396842105263158, -3.91, -2.502105263157895, -2.8968421052631586, -2.5678947368421055, -1.462631578947369, -2.857368421052632, -2.2915789473684214, -1.7784210526315791, -1.9626315789473687, -0.5678947368421055, -0.7784210526315792, -0.8968421052631582, -0.05473684210526353, -1.9363157894736844, -2.081052631578948, -2.3442105263157895, -1.9889473684210528, -0.34421052631578986, 1.011052631578947, 0.8399999999999995, 0.011052631578946898, -0.5810526315789478, -2.107368421052632, -1.9363157894736847, -2.4231578947368426, -2.2784210526315793, -1.0415789473684214, -0.5942105263157899, -1.5678947368421055, -0.4626315789473687, -1.0810526315789475, -2.9231578947368426, -1.6600000000000008, -2.331052631578948, -1.8310526315789482, 0.3268421052631576, -0.488947368421053, -0.6994736842105267, -1.1468421052631583, -1.0547368421052636, -0.18631578947368455, 0.4452631578947365, 0.8005263157894733, -0.19947368421052658, -0.0021052631578949432, -1.370526315789474, -1.633684210526316, -1.0810526315789477, -0.620526315789474, 0.5899999999999996, 0.36631578947368393, -0.04157894736842138, -0.3047368421052634, -1.002105263157895, -0.9231578947368424, -0.7915789473684214, -1.870526315789474, -0.9626315789473687, -1.265263157894737, -0.6336842105263161, 0.011052631578947036, -0.9231578947368424, -0.42315789473684245, -0.22578947368421093, 0.9452631578947366, 0.36631578947368393, -0.6863157894736847, -1.896842105263158, -2.5547368421052634, -1.396842105263158, -0.041578947368421326, 0.142631578947368, -0.00210526315789503, 0.774210526315789, 0.6821052631578943, 0.9847368421052628, 0.7478947368421048, 0.247894736842105, 0.8663157894736839, 0.7084210526315786, 0.9715789473684208, 0.12947368421052596, -0.3178947368421056, 0.22157894736842068, 0.03736842105263122]
  out "CH 0 Bin Readings":dbl[](array[numeric])=[139.0, 122.0, 123.0, 104.0, 107.0, 136.0, 99.0, 110.0, 122.0, 122.0, 107.0, 120.0, 107.0, 129.0, 120.0, 135.0, 126.0, 96.0, 136.0, 118.0, 116.0, 105.0, 141.0, 119.0, 98.0, 122.0, 145.0, 146.0, 133.0, 126.0, 133.0, 134.0, 126.0, 136.0, 132.0, 123.0, 142.0, 135.0, 133.0, 133.0, 136.0, 134.0, 134.0, 145.0, 121.0, 111.0, 125.0, 114.0, 111.0, 113.0, 112.0, 112.0, 111.0, 113.0, 116.0, 96.0, 91.0, 113.0, 88.0, 97.0, 101.0, 95.0, 102.0, 106.0, 90.0, 101.0, 107.0, 95.0, 82.0, 85.0, 92.0, 89.0, 97.0, 93.0, 95.0, 96.0, 97.0, 94.0, 91.0, 100.0, 108.0, 80.0, 83.0, 102.0, 72.0, 80.0, 81.0, 107.0, 82.0, 87.0, 84.0, 70.0, 94.0, 91.0, 91.0, 83.0, 90.0, 86.0, 85.0, 91.0, 78.0, 85.0, 81.0, 85.0, 87.0, 81.0, 90.0, 81.0, 87.0, 78.0, 81.0, 82.0, 99.0, 102.0, 121.0, 136.0, 153.0, 188.0, 219.0, 291.0, 308.0, 407.0, 531.0, 597.0, 630.0, 676.0, 708.0, 592.0, 554.0, 553.0, 513.0, 499.0, 458.0, 357.0, 317.0, 261.0, 208.0, 224.0, 207.0, 164.0, 147.0, 152.0, 160.0, 178.0, 143.0, 176.0, 134.0, 121.0, 132.0, 126.0, 125.0, 117.0, 112.0, 118.0, 127.0, 144.0, 128.0, 109.0, 100.0, 82.0, 102.0, 97.0, 95.0, 71.0, 95.0, 89.0, 77.0, 67.0, 75.0, 73.0, 79.0, 84.0, 104.0, 89.0, 88.0, 84.0, 90.0, 69.0, 78.0, 83.0, 92.0, 83.0, 82.0, 88.0, 75.0, 72.0, 73.0, 89.0, 76.0, 79.0, 82.0, 86.0, 64.0, 92.0, 87.0, 75.0, 88.0, 97.0, 86.0, 75.0, 80.0, 92.0, 64.0, 68.0, 70.0, 97.0, 72.0, 93.0, 89.0, 76.0, 98.0, 80.0, 74.0, 94.0, 85.0, 86.0, 94.0, 109.0, 80.0, 102.0, 79.0, 90.0, 91.0, 89.0, 77.0, 82.0, 85.0, 76.0, 85.0, 68.0, 79.0, 69.0, 82.0, 80.0, 82.0, 86.0, 72.0, 80.0, 106.0, 79.0, 77.0, 80.0, 82.0, 94.0, 90.0, 73.0, 86.0, 90.0, 65.0, 69.0, 68.0, 90.0, 83.0, 100.0, 93.0, 92.0, 76.0, 71.0, 80.0, 77.0, 85.0, 89.0, 104.0, 104.0, 74.0, 80.0, 79.0, 65.0, 67.0, 73.0, 84.0, 89.0, 88.0, 80.0, 106.0, 81.0, 74.0, 75.0, 73.0, 92.0, 72.0, 84.0, 66.0, 95.0, 77.0, 91.0, 81.0, 85.0, 81.0, 75.0, 80.0, 77.0, 89.0, 81.0, 81.0, 87.0, 76.0, 86.0, 91.0, 81.0, 84.0, 82.0, 66.0, 86.0, 81.0, 92.0, 87.0, 85.0, 70.0, 84.0, 81.0, 93.0, 80.0, 73.0, 83.0, 72.0, 99.0, 90.0, 73.0, 83.0, 91.0, 89.0, 81.0, 97.0, 81.0, 87.0, 82.0, 78.0, 76.0, 88.0, 72.0, 95.0, 74.0, 90.0, 62.0, 88.0, 74.0, 74.0, 88.0, 87.0, 89.0, 87.0, 88.0, 98.0, 84.0, 87.0, 84.0, 90.0, 69.0, 84.0, 91.0, 73.0, 78.0, 87.0, 89.0, 76.0, 82.0, 80.0, 81.0, 73.0, 74.0, 74.0, 81.0, 92.0, 66.0, 95.0, 80.0, 92.0, 80.0, 89.0, 79.0, 91.0, 88.0, 86.0, 105.0, 89.0, 92.0, 85.0, 73.0, 72.0, 80.0, 82.0, 102.0, 80.0, 92.0, 75.0, 85.0, 85.0, 94.0, 78.0, 85.0, 64.0, 75.0, 60.0, 94.0, 88.0, 79.0, 79.0, 85.0, 95.0, 93.0, 64.0, 83.0, 82.0, 71.0, 78.0, 81.0, 86.0, 76.0, 87.0, 75.0, 69.0, 98.0, 95.0, 83.0, 74.0, 78.0, 69.0, 91.0, 71.0, 91.0, 71.0, 79.0, 90.0, 78.0, 92.0, 85.0, 89.0, 75.0, 80.0, 65.0, 82.0, 79.0, 93.0, 78.0, 75.0, 96.0, 87.0, 78.0, 88.0, 71.0, 97.0, 84.0, 79.0, 86.0, 78.0, 79.0, 68.0, 82.0, 83.0, 82.0, 68.0, 95.0, 85.0, 84.0, 70.0, 98.0, 63.0, 68.0, 71.0, 90.0, 71.0, 81.0, 78.0, 89.0, 93.0, 63.0, 75.0, 59.0, 81.0, 77.0, 70.0, 78.0, 80.0, 71.0, 94.0, 86.0, 85.0, 82.0, 85.0, 83.0, 83.0, 89.0, 97.0, 74.0, 87.0, 80.0, 78.0, 89.0, 85.0, 85.0, 84.0, 98.0, 59.0, 75.0, 70.0, 73.0, 79.0, 86.0, 90.0, 80.0, 85.0, 71.0, 69.0, 79.0, 84.0, 91.0, 77.0, 84.0, 83.0, 89.0, 95.0, 79.0, 86.0, 80.0, 78.0, 94.0, 76.0, 70.0, 95.0, 73.0, 70.0, 71.0, 83.0, 91.0, 89.0, 87.0, 85.0, 88.0, 86.0, 79.0, 79.0, 81.0, 72.0, 56.0, 77.0, 85.0, 65.0, 87.0, 84.0, 85.0, 70.0, 86.0, 98.0, 78.0, 78.0, 99.0, 71.0, 83.0, 71.0, 87.0, 70.0, 83.0, 83.0, 77.0, 88.0, 82.0, 82.0, 89.0]
  out "Range Corrected Altitude Array":dbl[](array[numeric])=[1406.25, 5625.0, 12656.25, 22500.0, 35156.25, 50625.0, 68906.25, 90000.0, 113906.25, 140625.0, 170156.25, 202500.0, 237656.25, 275625.0, 316406.25, 360000.0, 406406.25, 455625.0, 507656.25, 562500.0, 620156.25, 680625.0, 743906.25, 810000.0, 878906.25, 950625.0, 1025156.25, 1102500.0, 1182656.25, 1265625.0, 1351406.25, 1440000.0, 1531406.25, 1625625.0, 1722656.25, 1822500.0, 1925156.25, 2030625.0, 2138906.25, 2250000.0, 2363906.25, 2480625.0, 2600156.25, 2722500.0, 2847656.25, 2975625.0, 3106406.25, 3240000.0, 3376406.25, 3515625.0, 3657656.25, 3802500.0, 3950156.25, 4100625.0, 4253906.25, 4410000.0, 4568906.25, 4730625.0, 4895156.25, 5062500.0, 5232656.25, 5405625.0, 5581406.25, 5760000.0, 5941406.25, 6125625.0, 6312656.25, 6502500.0, 6695156.25, 6890625.0, 7088906.25, 7290000.0, 7493906.25, 7700625.0, 7910156.25, 8122500.0, 8337656.25, 8555625.0, 8776406.25, 9000000.0, 9226406.25, 9455625.0, 9687656.25, 9922500.0, 10160156.25, 10400625.0, 10643906.25, 10890000.0, 11138906.25, 11390625.0, 11645156.25, 11902500.0, 12162656.25, 12425625.0, 12691406.25, 12960000.0, 13231406.25, 13505625.0, 13782656.25, 14062500.0, 14345156.25, 14630625.0, 14918906.25, 15210000.0, 15503906.25, 15800625.0, 16100156.25, 16402500.0, 16707656.25, 17015625.0, 17326406.25, 17640000.0, 17956406.25, 18275625.0, 18597656.25, 18922500.0, 19250156.25, 19580625.0, 19913906.25, 20250000.0, 20588906.25, 20930625.0, 21275156.25, 21622500.0, 21972656.25, 22325625.0, 22681406.25, 23040000.0, 23401406.25, 23765625.0, 24132656.25, 24502500.0, 24875156.25, 25250625.0, 25628906.25, 26010000.0, 26393906.25, 26780625.0, 27170156.25, 27562500.0, 27957656.25, 28355625.0, 28756406.25, 29160000.0, 29566406.25, 29975625.0, 30387656.25, 30802500.0, 31220156.25, 31640625.0, 32063906.25, 32490000.0, 32918906.25, 33350625.0, 33785156.25, 34222500.0, 34662656.25, 35105625.0, 35551406.25, 36000000.0, 36451406.25, 36905625.0, 37362656.25, 37822500.0, 38285156.25, 38750625.0, 39218906.25, 39690000.0, 40163906.25, 40640625.0, 41120156.25, 41602500.0, 42087656.25, 42575625.0, 43066406.25, 43560000.0, 44056406.25, 44555625.0, 45057656.25, 45562500.0, 46070156.25, 46580625.0, 47093906.25, 47610000.0, 48128906.25, 48650625.0, 49175156.25, 49702500.0, 50232656.25, 50765625.0, 51301406.25, 51840000.0, 52381406.25, 52925625.0, 53472656.25, 54022500.0, 54575156.25, 55130625.0, 55688906.25, 56250000.0, 56813906.25, 57380625.0, 57950156.25, 58522500.0, 59097656.25, 59675625.0, 60256406.25, 60840000.0, 61426406.25, 62015625.0, 62607656.25, 63202500.0, 63800156.25, 64400625.0, 65003906.25, 65610000.0, 66218906.25, 66830625.0, 67445156.25, 68062500.0, 68682656.25, 69305625.0, 69931406.25, 70560000.0, 71191406.25, 71825625.0, 72462656.25, 73102500.0, 73745156.25, 74390625.0, 75038906.25, 75690000.0, 76343906.25, 77000625.0, 77660156.25, 78322500.0, 78987656.25, 79655625.0, 80326406.25, 81000000.0, 81676406.25, 82355625.0, 83037656.25, 83722500.0, 84410156.25, 85100625.0, 85793906.25, 86490000.0, 87188906.25, 87890625.0, 88595156.25, 89302500.0, 90012656.25, 90725625.0, 91441406.25, 92160000.0, 92881406.25, 93605625.0, 94332656.25, 95062500.0, 95795156.25, 96530625.0, 97268906.25, 98010000.0, 98753906.25, 99500625.0, 100250156.25, 101002500.0, 101757656.25, 102515625.0, 103276406.25, 104040000.0, 104806406.25, 105575625.0, 106347656.25, 107122500.0, 107900156.25, 108680625.0, 109463906.25, 110250000.0, 111038906.25, 111830625.0, 112625156.25, 113422500.0, 114222656.25, 115025625.0, 115831406.25, 116640000.0, 117451406.25, 118265625.0, 119082656.25, 119902500.0, 120725156.25, 121550625.0, 122378906.25, 123210000.0, 124043906.25, 124880625.0, 125720156.25, 126562500.0, 127407656.25, 128255625.0, 129106406.25, 129960000.0, 130816406.25, 131675625.0, 132537656.25, 133402500.0, 134270156.25, 135140625.0, 136013906.25, 136890000.0, 137768906.25, 138650625.0, 139535156.25, 140422500.0, 141312656.25, 142205625.0, 143101406.25, 144000000.0, 144901406.25, 145805625.0, 146712656.25, 147622500.0, 148535156.25, 149450625.0, 150368906.25, 151290000.0, 152213906.25, 153140625.0, 154070156.25, 155002500.0, 155937656.25, 156875625.0, 157816406.25, 158760000.0, 159706406.25, 160655625.0, 161607656.25, 162562500.0, 163520156.25, 164480625.0, 165443906.25, 166410000.0, 167378906.25, 168350625.0, 169325156.25, 170302500.0, 171282656.25, 172265625.0, 173251406.25, 174240000.0, 175231406.25, 176225625.0, 177222656.25, 178222500.0, 179225156.25, 180230625.0, 181238906.25, 182250000.0, 183263906.25, 184280625.0, 185300156.25, 186322500.0, 187347656.25, 188375625.0, 189406406.25, 190440000.0, 191476406.25, 192515625.0, 193557656.25, 194602500.0, 195650156.25, 196700625.0, 197753906.25, 198810000.0, 199868906.25, 200930625.0, 201995156.25, 203062500.0, 204132656.25, 205205625.0, 206281406.25, 207360000.0, 208441406.25, 209525625.0, 210612656.25, 211702500.0, 212795156.25, 213890625.0, 214988906.25, 216090000.0, 217193906.25, 218300625.0, 219410156.25, 220522500.0, 221637656.25, 222755625.0, 223876406.25, 225000000.0, 226126406.25, 227255625.0, 228387656.25, 229522500.0, 230660156.25, 231800625.0, 232943906.25, 234090000.0, 235238906.25, 236390625.0, 237545156.25, 238702500.0, 239862656.25, 241025625.0, 242191406.25, 243360000.0, 244531406.25, 245705625.0, 246882656.25, 248062500.0, 249245156.25, 250430625.0, 251618906.25, 252810000.0, 254003906.25, 255200625.0, 256400156.25, 257602500.0, 258807656.25, 260015625.0, 261226406.25, 262440000.0, 263656406.25, 264875625.0, 266097656.25, 267322500.0, 268550156.25, 269780625.0, 271013906.25, 272250000.0, 273488906.25, 274730625.0, 275975156.25, 277222500.0, 278472656.25, 279725625.0, 280981406.25, 282240000.0, 283501406.25, 284765625.0, 286032656.25, 287302500.0, 288575156.25, 289850625.0, 291128906.25, 292410000.0, 293693906.25, 294980625.0, 296270156.25, 297562500.0, 298857656.25, 300155625.0, 301456406.25, 302760000.0, 304066406.25, 305375625.0, 306687656.25, 308002500.0, 309320156.25, 310640625.0, 311963906.25, 313290000.0, 314618906.25, 315950625.0, 317285156.25, 318622500.0, 319962656.25, 321305625.0, 322651406.25, 324000000.0, 325351406.25, 326705625.0, 328062656.25, 329422500.0, 330785156.25, 332150625.0, 333518906.25, 334890000.0, 336263906.25, 337640625.0, 339020156.25, 340402500.0, 341787656.25, 343175625.0, 344566406.25, 345960000.0, 347356406.25, 348755625.0, 350157656.25, 351562500.0, 352970156.25, 354380625.0, 355793906.25, 357210000.0, 358628906.25, 360050625.0, 361475156.25, 362902500.0, 364332656.25, 365765625.0, 367201406.25, 368640000.0, 370081406.25, 371525625.0, 372972656.25, 374422500.0, 375875156.25, 377330625.0, 378788906.25, 380250000.0, 381713906.25, 383180625.0, 384650156.25, 386122500.0, 387597656.25, 389075625.0, 390556406.25, 392040000.0, 393526406.25, 395015625.0, 396507656.25, 398002500.0, 399500156.25, 401000625.0, 402503906.25, 404010000.0, 405518906.25, 407030625.0, 408545156.25, 410062500.0, 411582656.25, 413105625.0, 414631406.25, 416160000.0, 417691406.25, 419225625.0, 420762656.25, 422302500.0, 423845156.25, 425390625.0, 426938906.25, 428490000.0, 430043906.25, 431600625.0, 433160156.25, 434722500.0, 436287656.25, 437855625.0, 439426406.25, 441000000.0]
  out "Altitude Array (km)":dbl[](array[numeric])=[0.0375, 0.075, 0.11249999999999999, 0.15, 0.1875, 0.225, 0.26249999999999996, 0.3, 0.33749999999999997, 0.37499999999999994, 0.4125, 0.44999999999999996, 0.48749999999999993, 0.525, 0.5625, 0.6, 0.6375, 0.6749999999999999, 0.7124999999999999, 0.75, 0.7875, 0.825, 0.8624999999999999, 0.8999999999999999, 0.9374999999999999, 0.975, 1.0125, 1.05, 1.0875000000000001, 1.125, 1.1625, 1.2, 1.2375, 1.2750000000000001, 1.3125, 1.35, 1.3875, 1.425, 1.4625000000000001, 1.5, 1.5375, 1.575, 1.6125, 1.6500000000000001, 1.6875, 1.725, 1.7625, 1.8, 1.8375, 1.875, 1.9125, 1.95, 1.9875, 2.025, 2.0625, 2.1, 2.1375, 2.175, 2.2125, 2.25, 2.2875, 2.325, 2.3625, 2.4, 2.4375, 2.475, 2.5125, 2.55, 2.5875, 2.625, 2.6625, 2.7, 2.7375, 2.775, 2.8125, 2.85, 2.8875, 2.925, 2.9625, 3.0, 3.0375, 3.075, 3.1125, 3.15, 3.1875, 3.225, 3.2625, 3.3, 3.3375, 3.375, 3.4125, 3.45, 3.4875, 3.525, 3.5625, 3.6, 3.6374999999999997, 3.675, 3.7125, 3.75, 3.7875, 3.8249999999999997, 3.8625, 3.9, 3.9375, 3.975, 4.012499999999999, 4.05, 4.0874999999999995, 4.124999999999999, 4.1625, 4.199999999999999, 4.2375, 4.2749999999999995, 4.312499999999999, 4.35, 4.387499999999999, 4.425, 4.4624999999999995, 4.499999999999999, 4.5375, 4.574999999999999, 4.6125, 4.6499999999999995, 4.687499999999999, 4.725, 4.762499999999999, 4.8, 4.8374999999999995, 4.874999999999999, 4.9125, 4.949999999999999, 4.9875, 5.0249999999999995, 5.062499999999999, 5.1, 5.137499999999999, 5.175, 5.2124999999999995, 5.249999999999999, 5.2875, 5.324999999999999, 5.3625, 5.3999999999999995, 5.437499999999999, 5.475, 5.512499999999999, 5.55, 5.5874999999999995, 5.624999999999999, 5.6625, 5.699999999999999, 5.7375, 5.7749999999999995, 5.812499999999999, 5.85, 5.887499999999999, 5.925, 5.9624999999999995, 5.999999999999999, 6.0375, 6.074999999999999, 6.1125, 6.1499999999999995, 6.187499999999999, 6.225, 6.262499999999999, 6.3, 6.3374999999999995, 6.374999999999999, 6.4125, 6.449999999999999, 6.4875, 6.5249999999999995, 6.562499999999999, 6.6, 6.637499999999999, 6.675, 6.7124999999999995, 6.749999999999999, 6.7875, 6.824999999999999, 6.8625, 6.8999999999999995, 6.937499999999999, 6.975, 7.012499999999999, 7.05, 7.0874999999999995, 7.124999999999999, 7.1625, 7.199999999999999, 7.237499999999999, 7.2749999999999995, 7.312499999999999, 7.35, 7.387499999999999, 7.424999999999999, 7.4624999999999995, 7.499999999999999, 7.5375, 7.574999999999999, 7.612499999999999, 7.6499999999999995, 7.687499999999999, 7.725, 7.762499999999999, 7.799999999999999, 7.8374999999999995, 7.874999999999999, 7.9125, 7.949999999999999, 7.987499999999999, 8.025, 8.0625, 8.1, 8.1375, 8.174999999999999, 8.212499999999999, 8.25, 8.2875, 8.325, 8.362499999999999, 8.399999999999999, 8.4375, 8.475, 8.5125, 8.549999999999999, 8.587499999999999, 8.625, 8.6625, 8.7, 8.737499999999999, 8.774999999999999, 8.8125, 8.85, 8.8875, 8.924999999999999, 8.962499999999999, 9.0, 9.0375, 9.075, 9.112499999999999, 9.149999999999999, 9.1875, 9.225, 9.2625, 9.299999999999999, 9.337499999999999, 9.375, 9.4125, 9.45, 9.487499999999999, 9.524999999999999, 9.5625, 9.6, 9.6375, 9.674999999999999, 9.712499999999999, 9.75, 9.7875, 9.825, 9.862499999999999, 9.899999999999999, 9.9375, 9.975, 10.0125, 10.049999999999999, 10.087499999999999, 10.125, 10.1625, 10.2, 10.237499999999999, 10.274999999999999, 10.3125, 10.35, 10.3875, 10.424999999999999, 10.462499999999999, 10.5, 10.5375, 10.575, 10.612499999999999, 10.649999999999999, 10.6875, 10.725, 10.7625, 10.799999999999999, 10.837499999999999, 10.875, 10.9125, 10.95, 10.987499999999999, 11.024999999999999, 11.0625, 11.1, 11.1375, 11.174999999999999, 11.212499999999999, 11.25, 11.2875, 11.325, 11.362499999999999, 11.399999999999999, 11.4375, 11.475, 11.5125, 11.549999999999999, 11.587499999999999, 11.625, 11.6625, 11.7, 11.737499999999999, 11.774999999999999, 11.8125, 11.85, 11.8875, 11.924999999999999, 11.962499999999999, 12.0, 12.0375, 12.075, 12.112499999999999, 12.149999999999999, 12.1875, 12.225, 12.2625, 12.299999999999999, 12.337499999999999, 12.375, 12.4125, 12.45, 12.487499999999999, 12.524999999999999, 12.5625, 12.6, 12.6375, 12.674999999999999, 12.712499999999999, 12.75, 12.7875, 12.825, 12.862499999999999, 12.899999999999999, 12.9375, 12.975, 13.0125, 13.049999999999999, 13.087499999999999, 13.125, 13.1625, 13.2, 13.237499999999999, 13.274999999999999, 13.3125, 13.35, 13.3875, 13.424999999999999, 13.462499999999999, 13.5, 13.5375, 13.575, 13.612499999999999, 13.649999999999999, 13.6875, 13.725, 13.7625, 13.799999999999999, 13.837499999999999, 13.875, 13.9125, 13.95, 13.987499999999999, 14.024999999999999, 14.0625, 14.1, 14.1375, 14.174999999999999, 14.212499999999999, 14.25, 14.2875, 14.325, 14.362499999999999, 14.399999999999999, 14.437499999999998, 14.475, 14.5125, 14.549999999999999, 14.587499999999999, 14.624999999999998, 14.6625, 14.7, 14.737499999999999, 14.774999999999999, 14.812499999999998, 14.85, 14.8875, 14.924999999999999, 14.962499999999999, 14.999999999999998, 15.0375, 15.075, 15.112499999999999, 15.149999999999999, 15.187499999999998, 15.225, 15.2625, 15.299999999999999, 15.337499999999999, 15.374999999999998, 15.4125, 15.45, 15.487499999999999, 15.524999999999999, 15.562499999999998, 15.6, 15.6375, 15.674999999999999, 15.712499999999999, 15.749999999999998, 15.7875, 15.825, 15.862499999999999, 15.899999999999999, 15.937499999999998, 15.975, 16.0125, 16.05, 16.087500000000002, 16.125, 16.1625, 16.2, 16.2375, 16.275000000000002, 16.3125, 16.35, 16.3875, 16.425, 16.462500000000002, 16.5, 16.5375, 16.575, 16.6125, 16.650000000000002, 16.6875, 16.725, 16.7625, 16.8, 16.837500000000002, 16.875, 16.9125, 16.95, 16.9875, 17.025000000000002, 17.0625, 17.1, 17.1375, 17.175, 17.212500000000002, 17.25, 17.2875, 17.325, 17.3625, 17.400000000000002, 17.4375, 17.475, 17.5125, 17.55, 17.587500000000002, 17.625, 17.6625, 17.7, 17.7375, 17.775000000000002, 17.8125, 17.85, 17.8875, 17.925, 17.962500000000002, 18.0, 18.0375, 18.075, 18.1125, 18.150000000000002, 18.1875, 18.225, 18.2625, 18.3, 18.337500000000002, 18.375, 18.4125, 18.45, 18.4875, 18.525000000000002, 18.5625, 18.6, 18.6375, 18.675, 18.712500000000002, 18.75, 18.7875, 18.825, 18.8625, 18.900000000000002, 18.9375, 18.975, 19.0125, 19.05, 19.087500000000002, 19.125, 19.1625, 19.2, 19.2375, 19.275000000000002, 19.3125, 19.35, 19.3875, 19.425, 19.462500000000002, 19.5, 19.5375, 19.575, 19.6125, 19.650000000000002, 19.6875, 19.725, 19.7625, 19.8, 19.837500000000002, 19.875, 19.9125, 19.95, 19.9875, 20.025000000000002, 20.0625, 20.1, 20.1375, 20.175, 20.212500000000002, 20.25, 20.2875, 20.325, 20.3625, 20.400000000000002, 20.4375, 20.475, 20.5125, 20.55, 20.587500000000002, 20.625, 20.6625, 20.7, 20.7375, 20.775000000000002, 20.8125, 20.85, 20.8875, 20.925, 20.962500000000002, 21.0]
  out "Offline Pulse Energy":dbl=5.278258571428572
  out "Online Pulse Energy":dbl=5.272677142857142
  in  "Instrument Control":T5(tab)
  in  "Device In":refnum<visa-resource-name>="GPIB0::10::INSTR"
  in  "Settings":T6={"Module"=enum."WV Online TEC", "WV Online TEC"=23.195000000000437, "WV Online LD"=0.175, "WV Offline TEC"=29.654250000000104, "WV Offline LD"=0.17, "WV Etalon TEC"=28.0, "HSRL Etalon TEC"=25.954, "HSRL TEC"=14.334749999999692, "HSRL LD"=0.16} {"HSRL LD" min=0.0 max=0.18 step=0.001 format="%.3p"; "HSRL TEC" min=14.0 max=28.0 step=0.1 format="%.3g"; "WV Offline LD" min=0.0 max=0.18 step=0.001 format="%.3p"; "WV Online LD" min=0.0 max=0.18 step=0.001 format="%.3p"; "HSRL Etalon TEC" format="%.2g"; "WV Etalon TEC" format="%.2g"; "WV Offline TEC" min=16.0 max=30.0 step=0.1 format="%.3g"; "WV Online TEC" min=14.0 max=28.0 step=0.1 format="%.3g"}
  out "Readings":T7={"Pro8000"=TRUE, "WV OnLine TEC"=23.200861, "WV Online TEC"=TRUE, "WV Online LD"=0.17513673, "WV Online LD"=TRUE, "WV Offline TEC"=29.6676273, "WV Offline TEC"=TRUE, "WV Offline LD"=0.170396492, "WV Offline LD"=TRUE, "WV EtalonTEC"=28.2536545, "WV Etalon TEC"=TRUE, "HSRL Etalon TEC"=25.9546051, "HSRL Etalon TEC"=TRUE, "HSRL TEC"=14.3448429, "HSRL TEC "=TRUE, "HSRL LD"=0.160277352, "HSRL LD"=TRUE} {"HSRL LD" format="%.3p"; "HSRL TEC" format="%.3g"; "WV Offline LD" format="%.3p"; "WV Online LD" format="%.3p"; "HSRL Etalon TEC" format="%.3g"; "WV EtalonTEC" format="%.3g"; "WV Offline TEC" format="%.3g"; "WV OnLine TEC" format="%.3g"}
  in  "Pulse B Polarity":enum32{"Low", "High"}(ring)=enum."High"
  in  "Pulse A Delay(ns)":u32=1040 min=80 max=327600
  in  "Pulse B Delay(ns)":u32=170000 min=80 max=327600 step=1
  in  "Accumulation Delay(ns)":u32=10 min=10 max=1270 step=1
  in  "Sync Pulse Polarity":enum32{"Low", "High"}(ring)=enum."High"
  in  "Pulse A Polarity":enum32{"Low", "High"}(ring)=enum."High"
  in  "Number of Bins":u32=560 min=2 max=4095 step=1
  in  "Number of Accumulates":u32=14285 min=1 max=32767 step=1
  in  "Time Resolution Per Bin(ns)":u32=250 min=5 max=1063 step=1
  out "AMCS_Profile":i32=6265
  in  "WV Online Set (nm)":dbl=828.198 format="%.5f"
  out "WV Online Read (nm)":dbl=828.1979656628873 format="%.5f"
  out "WV Offline Read (nm)":dbl=828.2977247592468 format="%.5f"
  in  "WV Offline Set (nm)":dbl=828.29765 format="%.5f"
  in  "Bristol In":i32=5
  out "Bristol Out":i32
  out "Online_Diff":dbl=-3.433711265188322e-05 format="%#_3e"
  out "Oflline_Diff":dbl=7.475924678601586e-05 format="%#_3e"
  out "WV Online Locked":bool=TRUE
  out "WV Oflline Locked":bool=TRUE
  in  "calculate absorption cross sections":bool
  in  "Online_Tol":dbl=7.5e-05 format="%#_15g"
  in  "Cancel online":bool
  in  "Offline_Tol":dbl=7.5e-05 format="%#_15g"
  in  "Cancel Offline":bool
  in  "temp step size":dbl=0.00025 format="%#_6p"
  in  "HSRL_Tol":dbl=7.5e-05 format="%#_15g"
  out "HSRL_Diff":dbl=-3.035596193967649e-05 format="%#_3e"
  in  "Cancel HSRL":bool
  out "HSRL Locked":bool=TRUE
  out "HSRL Read (nm)":dbl=780.2460896440381 format="%.5f"
  in  "HSRL Set (nm)":dbl=780.24612 format="%#.5f"
  in  "Smoothing Range":dbl=150.0
  in  "Total DIAL Integration Time (Minutes)":i32=3
  in  "Data Reads (number of loops)":i32=1
  in  "Total Aerosol Integration Time (Minutes)":dbl=0.5
  in  "Scalar Wait Time":u32
  out "Smoothed Bins":dbl=4.0
  in  "NewportIn":string
  in  "logging":bool
  out "Newport Device Key":string="1918-R 15120"
  in  "SampleSize":i32=2
  out "NewportRef":refnum<k24>
  in  "Switch Comm Port":refnum<visa-resource-name>="COM3"
  out "FF_On_Ref":refnum<file>
  out "FF_On_Ptr":i64=2318336 format="%.2p"
  out "FF_Off_Ref":refnum<file>
  out "FF_Off_Ptr":i64=2318336 format="%.2p"
  out "NF_On_Ref":refnum<file>
  out "NF_On_Ptr":i64=2318336 format="%.2p"
  out "NF_Off_Ref":refnum<file>
  out "NF_Off_Ptr":i64=2318336 format="%.2p"
  out "DataOpen":bool=TRUE
  out "File Path_Far Field (out)":string="C:\\Users\\H2ODial\\Desktop\\SharedTeleWVData\\170508FF\\22"
  out "File Path_Near Field (out)":string="C:\\Users\\H2ODial\\Desktop\\SharedTeleWVData\\170508NF\\22"
  in  "Data File DIR (in)":string="C:\\Users\\H2ODial\\Desktop\\SharedTeleWVData\\"
  out "TRHP":T8={"Temp C"=14.848290598290603, "RelH %"=75.49297924297925, "Press hPa"=836.7032967032967, "AbH g/m^3"=9.416971916971917}
  in  "WS visa":refnum<visa-resource-name>="COM6"
  in  "WS_On/Off":bool=TRUE
  in  "bins":u32=560 min=2 max=4095 step=1
  out "y offset":u32=10
  in  "ns scale":u32=250
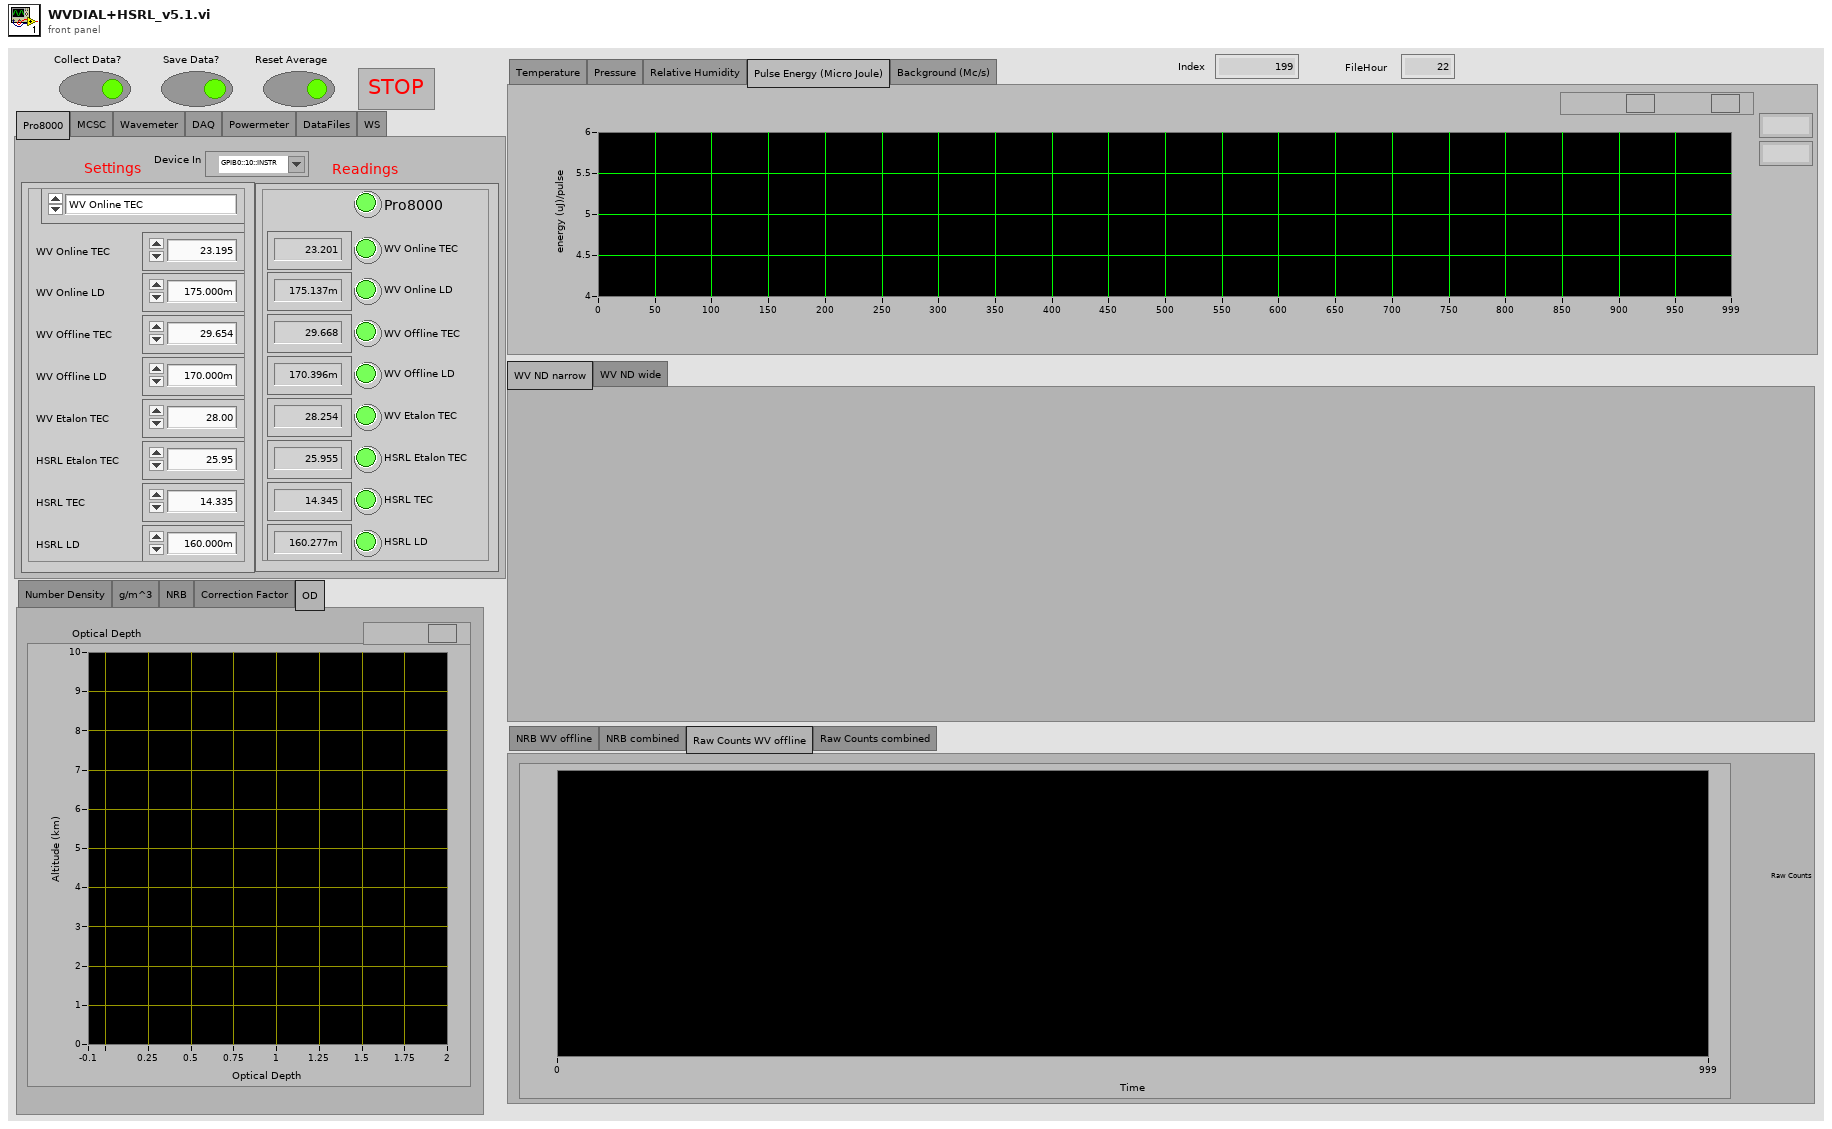
[diagram p1: front panel]
types:
  T1 = enum32{"NRB WV offline", "NRB combined", "Raw Counts WV offline", "Raw Counts combined"}
  T2 = enum32{"Number Density", "g/m^3", "NRB", "Correction Factor", "OD"}
  T3 = enum32{"Temperature", "Pressure", "Relative Humidity", "Pulse Energy (Micro Joule)", "Background (Mc/s)"}
  T4 = cluster{"Online Pulse Energy":dbl, "Pulse Energy Offline":dbl}
  T5 = enum32{"Pro8000", "MCSC", "Wavemeter", "DAQ", "Powermeter", "DataFiles", "WS"}
  T6 = cluster{"Module":enum16{"WV Online TEC", "WV Online LD", "WV Offline TEC", "WV Offline LD", "WV Etalon TEC", "HSRL Etalon TEC", "HSRL TEC", "HSRL LD"}, "WV Online TEC":dbl, "WV Online LD":dbl, "WV Offline TEC":dbl, "WV Offline LD":dbl, "WV Etalon TEC":dbl, "HSRL Etalon TEC":dbl, "HSRL TEC":dbl, "HSRL LD":dbl}
  T7 = cluster{"Pro8000":bool, "WV OnLine TEC":dbl, "WV Online TEC":bool, "WV Online LD":dbl, "WV Online LD":bool, "WV Offline TEC":dbl, "WV Offline TEC":bool, "WV Offline LD":dbl, "WV Offline LD":bool, "WV EtalonTEC":dbl, "WV Etalon TEC":bool, "HSRL Etalon TEC":dbl, "HSRL Etalon TEC":bool, "HSRL TEC":dbl, "HSRL TEC ":bool, "HSRL LD":dbl, "HSRL LD":bool}
  T8 = cluster{"Temp C":dbl, "RelH %":dbl, "Press hPa":dbl, "AbH g/m^3":dbl}
  T9 = enum16{"Open_TL", "Close_TL", "Verify_ID", "TEC_Sensor", "SET", "READ", "ON", "OFF", "Set_Limits", "Read_Limits", "Enable_Status", "Read_Status"}
  T10 = enum16{"Initialize ILX", "Set ON T", "Set Off T", "Set ON I", "Set Off I", "Set On Lim", "Set Off Lim", "Read ILX", "TEC ON/OFF", "LASER ON/OFF", "Status?", "ILX OFF"}
  T11 = enum16{"open", "replace", "create", "open or create", "replace or create", "replace or create with confirmation"}
  T12 = enum16{"WV Online TEC", "WV Online LD", "WV Offline TEC", "WV Offline LD", "WV Etalon TEC", "HSRL Etalon TEC", "HSRL TEC", "HSRL LD"}
  T13 = cluster{"Temp":dbl, "RelH":dbl, "Press":dbl, "AbH":dbl}
  T14 = typedef "LVDateTimeRec.ctl" = cluster{"fractional second":dbl, "second":i32, "minute":i32, "hour":i32, "day of month":i32, "month":i32, "year":i32, "day of week":i32, "day of year":i32, "DST":i32}
  T15 = cluster{"Online Pulse Energy":dbl, "Offline Pulse Energy":dbl}
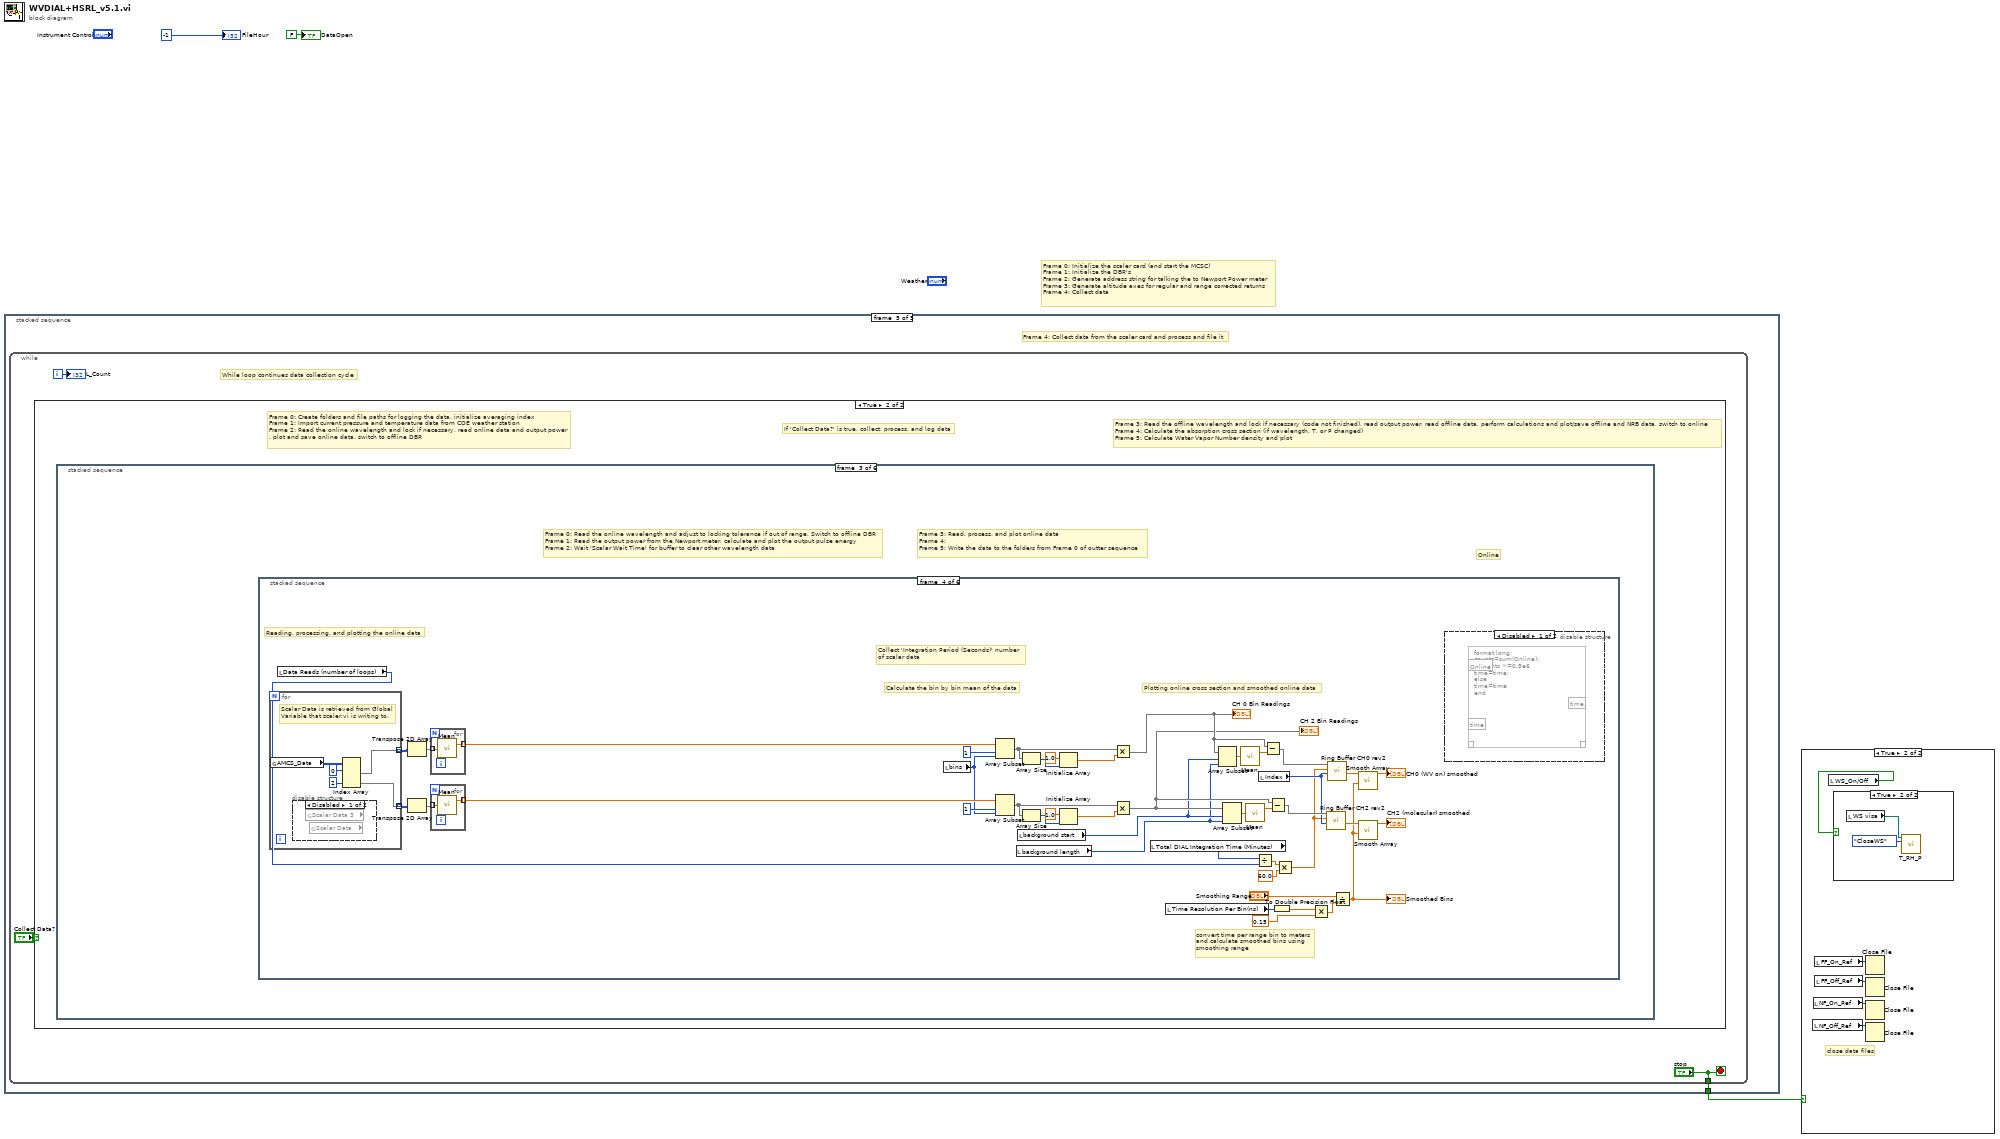
[diagram p0: block diagram]
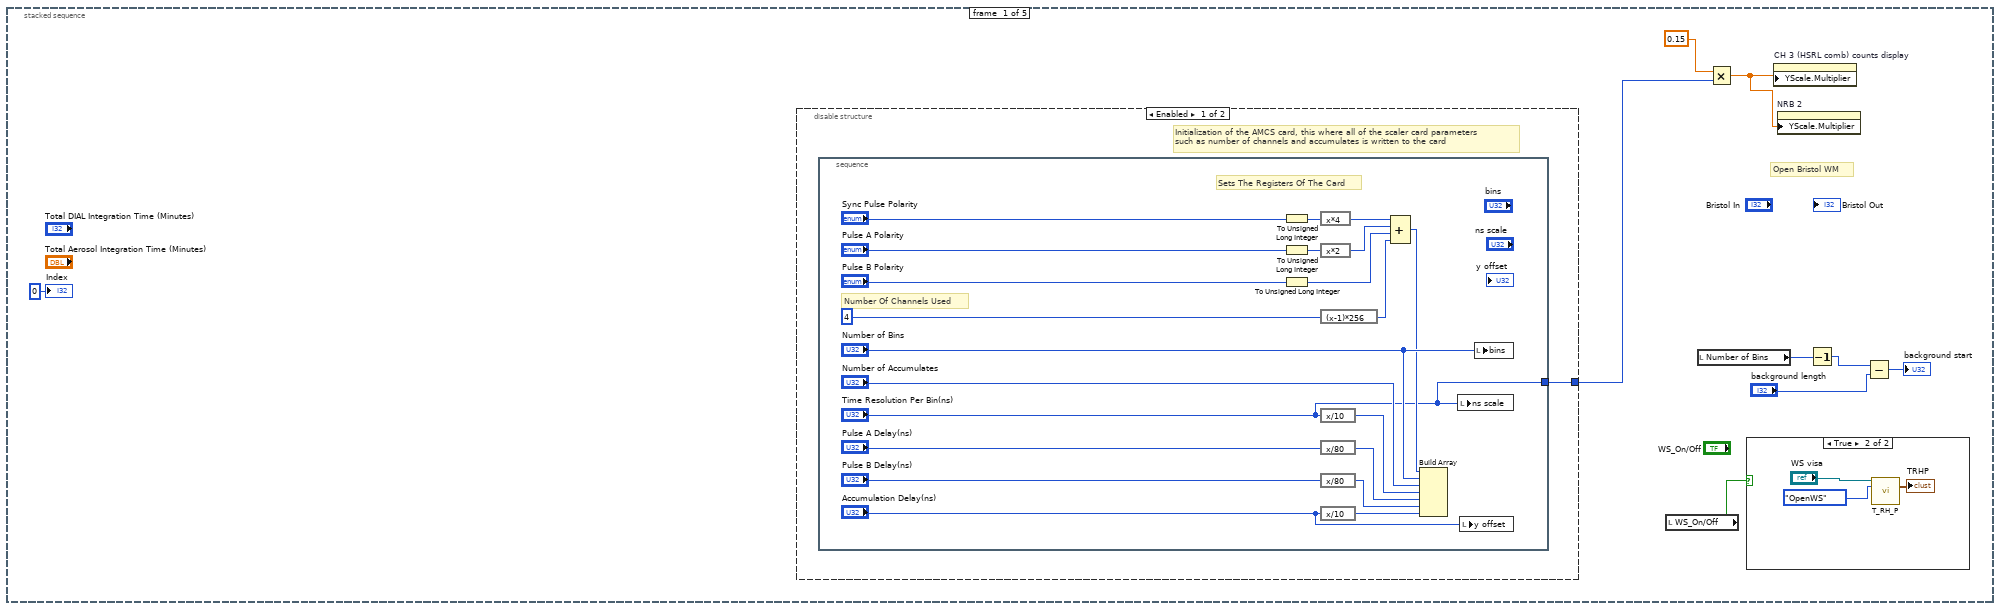
[diagram p4: hidden frame]
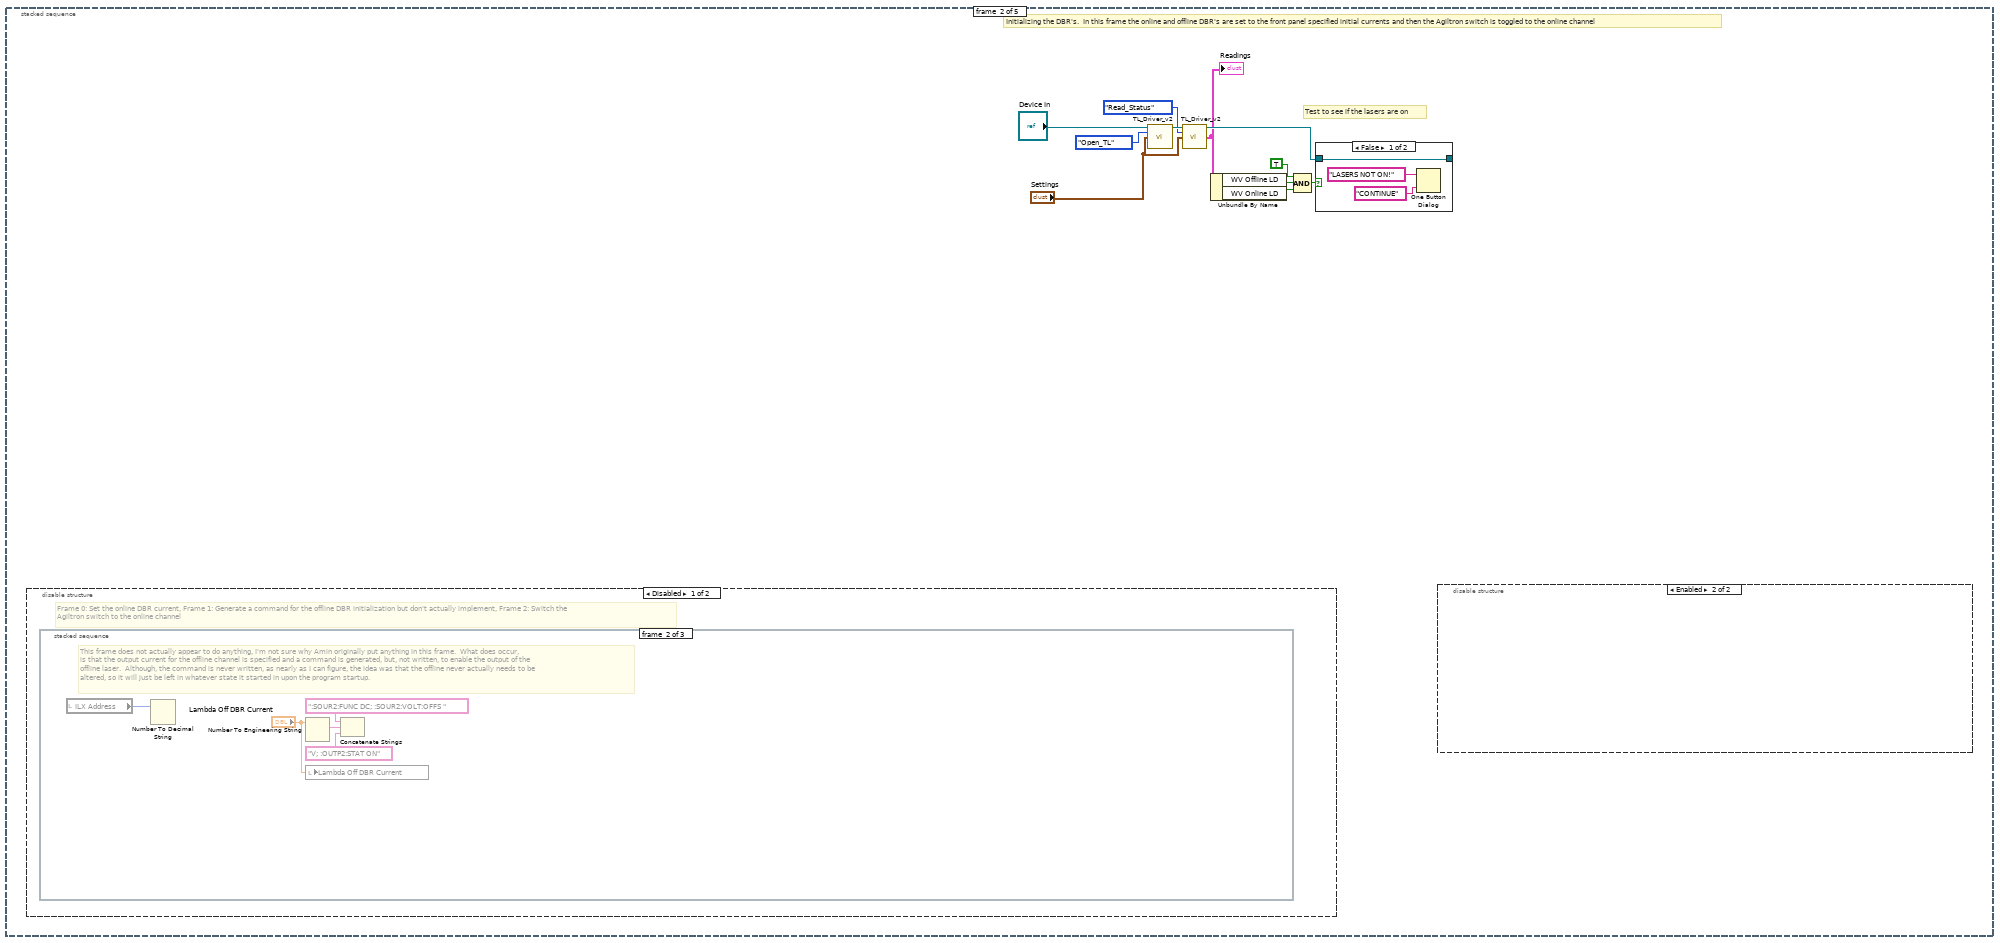
[diagram p7: hidden frame]
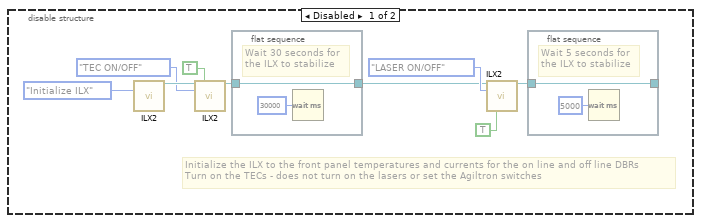
[diagram p9: hidden frame]
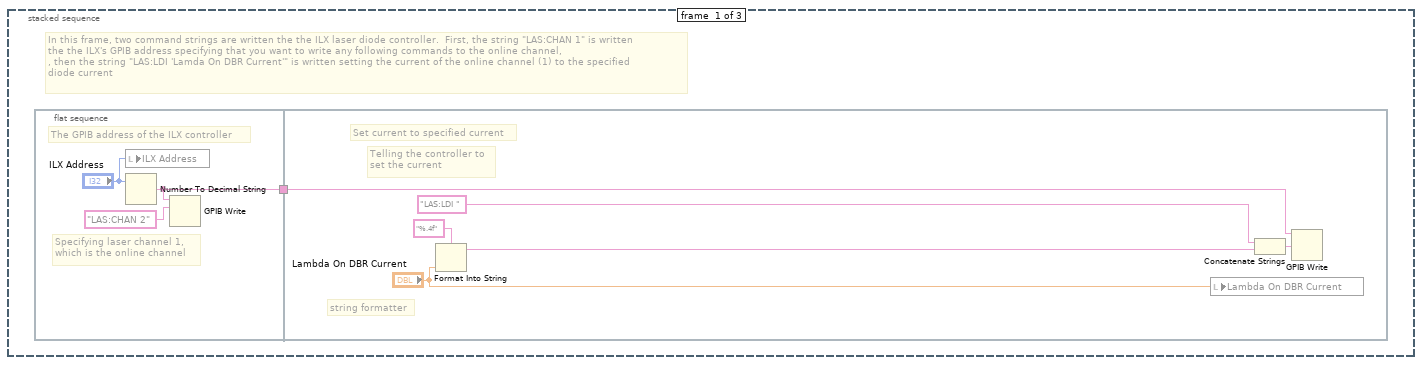
[diagram p10: hidden frame]
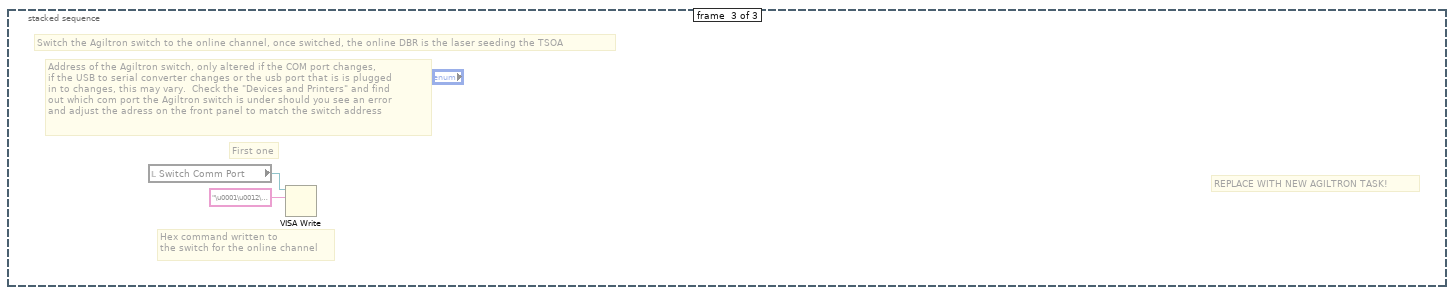
[diagram p11: hidden frame]
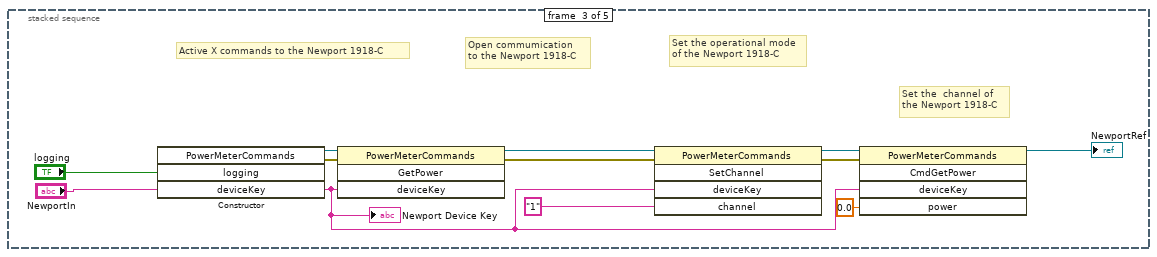
[diagram p13: hidden frame]
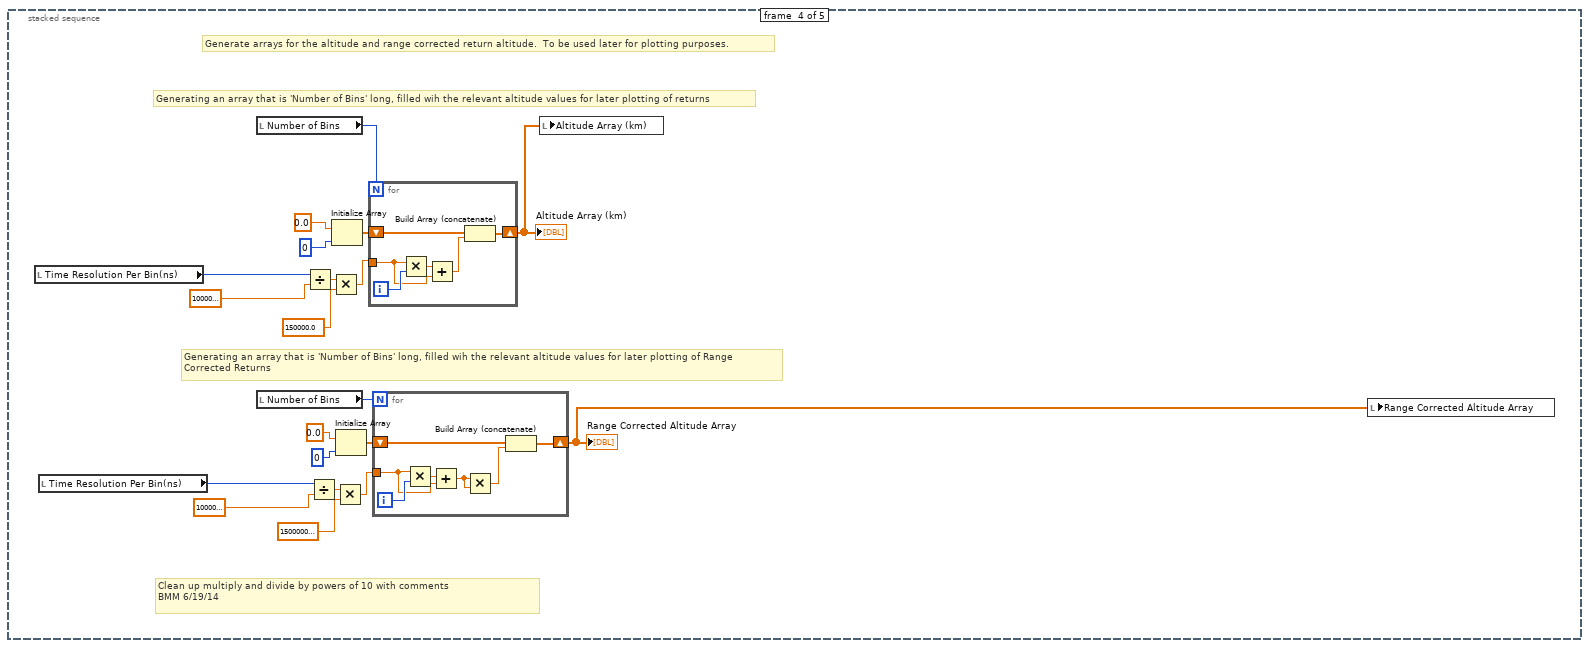
[diagram p14: hidden frame]
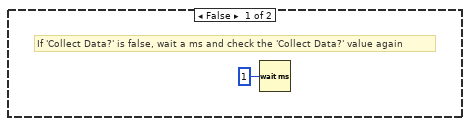
[diagram p15: hidden frame]
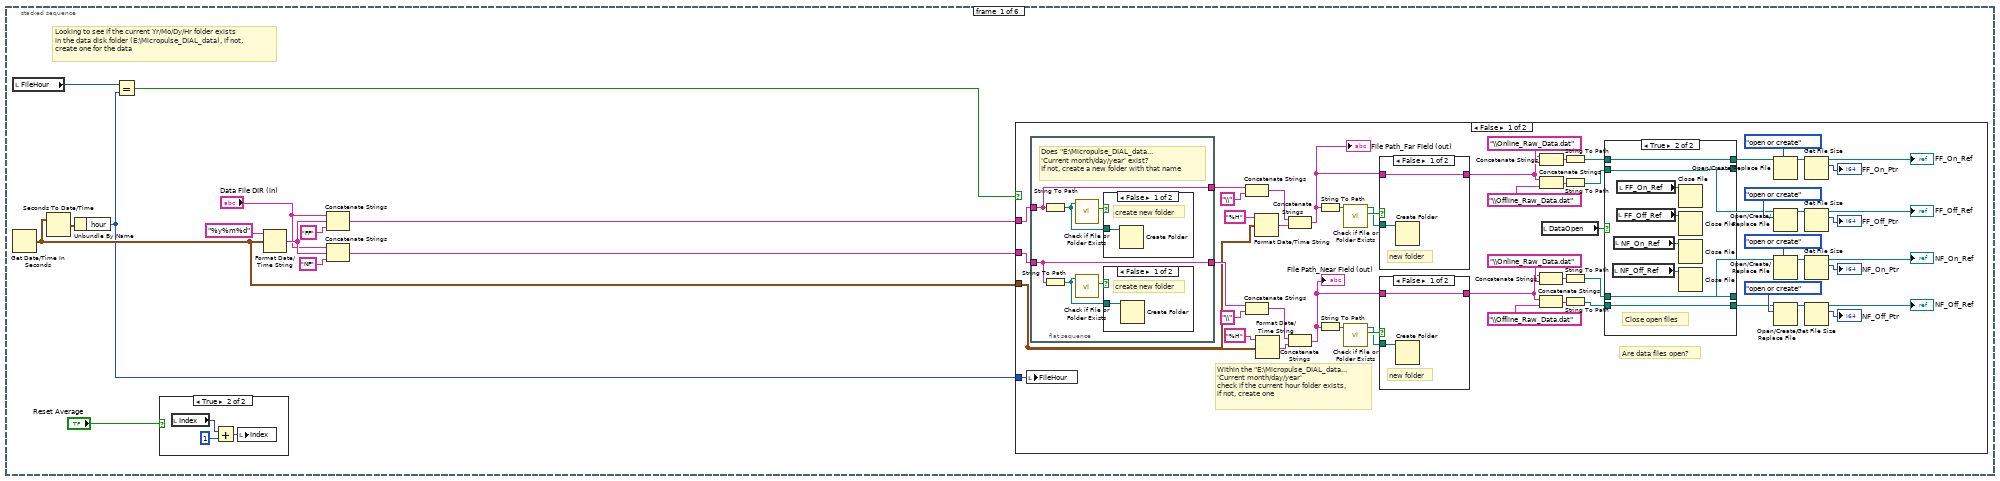
[diagram p16: hidden frame]
diagram:
  # "Frame 0: Initialize the scaler card (and start the MCSC)\nFrame 1: Initialize the DBR's\nFrame 2: Generate address string for talking the to Newport Power meter\nFrame 3: Generate altitude axes for regular and range corrected returns\nFrame 4: Collect data"
  n1 = stacked-sequence {
    tunnel: [_ _ _ _ w128] -> w3
    frame #0 {
      # "Open Bristol WM"
      n2 = disable-structure shown="Enabled" {
        disable-tunnel: [w16 _] -> w5
        frame Enabled {
          # "Initialization of the AMCS card, this where all of the scaler card parameters\nsuch as number of channels and accumulates is written to the card"
          n3 = stacked-sequence {
            tunnel: ["Time Resolution Per Bin(ns)"] -> w16
            frame #0 {
              # "Sets The Registers Of The Card"
              # "Number Of Channels Used"
              n4 = To Unsigned Long Integer(number="Sync Pulse Polarity") -> (unsigned 32bit integer=w18:u32)
              n5 = To Unsigned Long Integer(number="Pulse A Polarity") -> (unsigned 32bit integer=w22:u32)
              n6 = To Unsigned Long Integer(number="Pulse B Polarity") -> (unsigned 32bit integer=w20:u32)
              n7 = expression code="x*4"(w18) -> (w27:u32)
              n8 = expression code="x*2"(w22) -> (w26:u32)
              n9 = expression code="(x-1)*256"(u32 4 ("Number of Channels Used")) -> (w25:u32)
              n10 = expression code="x/10"("Time Resolution Per Bin(ns)") -> (w28:u32)
              n11 = expression code="x/80"("Pulse A Delay(ns)") -> (w35:u32)
              n12 = expression code="x/80"("Pulse B Delay(ns)") -> (w37:u32)
              n13 = expression code="x/10"("Accumulation Delay(ns)") -> (w36:u32)
              n14 = Compound Arithmetic op=ADD(w27, w26, w20, w25) -> (w24:u32)
              n15 = Build Array(w24, "Number of Bins", "Number of Accumulates", w28, w35, w37, w36) -> ()  [unwired: 1 out]
              n16 = local write "ns scale"("Time Resolution Per Bin(ns)") -> ()
              n17 = local write "y offset"("Accumulation Delay(ns)") -> ()
              n18 = local write "bins"("Number of Bins") -> ()
            }
          }
        }
        frame Disabled {
        }
      }
      n19 = local read "WS_On/Off"() -> (w7:bool)
      n20 = local read "Number of Bins"() -> (w11:u32)
      n21 = Multiply(x=0.15, y=w5) -> (x*y=w4:dbl)
      n22 = case shown="True" w7 {
        frame False {
        }
        frame True {
          n23 = call "T_RH_P.vi"("VISA in"="WS visa", "WS_Commands"=enum16{"OpenWS", "ReadTRHP", "CloseWS"}."OpenWS") -> ("TRHP"=→"TRHP":T13)  [unwired: 11 in, 2 out]
        }
      }
      n24 = property on="CH 3 (HSRL comb) counts display" class="IntChart (strict)"("YScale.Multiplier"=w4) -> ()  [unwired: 2 in, 2 out]
      n25 = property on="NRB 2" class="IntChart (strict)"("YScale.Multiplier"=w4) -> ()  [unwired: 2 in, 2 out]
      n26 = Decrement(x=w11) -> (x-1=w10:u32)
      n27 = Subtract(x=w10, y="background length") -> (x-y=→"background start":u32)
      "Index" <- 0 ("Index")
    }
    frame #1 {
      # "Test to see if the lasers are on"
      # "Initializing the DBR's.  In this frame the online and offline DBR's are set to the front panel specified initial currents and then the Agiltron switch is toggled to the online channel"
      n28 = disable-structure shown="Disabled" {
        frame Disabled {
          # "Frame 0: Set the online DBR current, Frame 1: Generate a command for the offline DBR initialization but don't actually implement, Frame 2: Switch the \nAgiltron switch to the online channel"
          n29 = stacked-sequence {
            frame #0 {
              # "In this frame, two command strings are written the the ILX laser diode controller.  First, the string \"LAS:CHAN 1\" is written\nthe the ILX's GPIB address specifying that you want to write any following commands to the online channel,\n, then the string \"LAS:LDI 'Lamda On DBR Current'\" is written setting the current of the online channel (1) to the specified \ndiode current"
              n30 = flat-sequence {
                tunnel: [w68] -> w66
                tunnel: w66 -> [w70]
                frame #0 {
                  # "The GPIB address of the ILX controller"
                  # "Specifying laser channel 1,\nwhich is the online channel"
                  n31 = local write "ILX Address"("ILX Address") -> ()
                  n32 = Number To Decimal String(number="ILX Address") -> (decimal integer string=w68:string)  [unwired: 1 in]
                  n33 = GPIB Write(0:w68, 1:"LAS:CHAN 2") -> ()  [unwired: 3 in, 2 out]
                }
                frame #1 {
                  # "Telling the controller to\nset the current"
                  # "string formatter"
                  # "Set current to specified current"
                  n34 = Format Into String(format string="%.4f" ("Format String"), "Lambda On DBR Current") -> (resulting string=w73:string)  [unwired: 2 in, 1 out]
                  n35 = local write "Lambda On DBR Current"("Lambda On DBR Current") -> ()
                  n36 = Concatenate Strings("LAS:LDI ", w73) -> (w74:string)
                  n37 = GPIB Write(0:w70, 1:w74) -> ()  [unwired: 3 in, 2 out]
                }
              }
            }
            frame #1 {
              # "This frame does not actually appear to do anything, I'm not sure why Amin originally put anything in this frame.  What does occur, \nis that the output current for the offline channel is specified and a command is generated, but, not written, to enable the output of the\noffline laser.  Although, the command is never written, as nearly as I can figure, the idea was that the offline never actually needs to be \naltered, so it will just be left in whatever state it started in upon the program startup."
              n38 = local read "ILX Address"() -> (w76:i32)
              n39 = Number To Decimal String(number=w76) -> ()  [unwired: 1 in, 1 out]
              n40 = Number To Engineering String(4:"Lambda Off DBR Current") -> (0:w80:string)  [unwired: 3 in]
              n41 = local write "Lambda Off DBR Current"("Lambda Off DBR Current") -> ()
              n42 = Concatenate Strings(":SOUR2:FUNC DC; :SOUR2:VOLT:OFFS ", w80, "V; :OUTP2:STAT ON") -> ()  [unwired: 1 out]
            }
            frame #2 {
              # "REPLACE WITH NEW AGILTRON TASK!"
              # "First one"
              # "Address of the Agiltron switch, only altered if the COM port changes,\nif the USB to serial converter changes or the usb port that is is plugged\nin to changes, this may vary.  Check the \"Devices and Printers\" and find \nout which com port the Agiltron switch is under should you see an error \nand adjust the adress on the front panel to match the switch address"
              # "Hex command written to \nthe switch for the online channel"
              # "Switch the Agiltron switch to the online channel, once switched, the online DBR is the laser seeding the TSOA"
              n43 = local read "Switch Comm Port"() -> (w81:refnum<visa-resource-name>)
              n44 = VISA Write(VISA resource name=w81, write buffer="\u0001\u0012\u0000\u0002") -> ()  [unwired: 1 in, 3 out]
            }
          }
        }
        frame Enabled {
        }
      }
      n45 = call "TL_Driver_v2.vi"("Device In"="Device In", "Commands"=T9."Open_TL", "Settings"="Settings") -> ("Device Out"=w46:refnum<visa-resource-name>)  [unwired: 9 in, 3 out]
      n46 = call "TL_Driver_v2.vi"("Device In"=w46, "Commands"=T9."Read_Status", "Settings"="Settings") -> ("Device Out"=w44:refnum<visa-resource-name>, "Readings"=w38:T7)  [unwired: 9 in, 2 out]
      "Readings" <- w38
      n47 = Unbundle By Name(w38) -> ("WV Offline LD"=w41:bool, "WV Online LD"=w42:bool)
      n48 = Compound Arithmetic op=AND(TRUE, w41, w42) -> (w40:bool)
      n49 = case shown="False" w40 {
        tunnel: w44 -> [w49 w52]
        tunnel: [w49 w52] -> _
        frame False {
          n50 = One Button Dialog(message="LASERS NOT ON!", button name ("OK")="CONTINUE") -> ()  [unwired: 1 out]
        }
        frame True {
        }
      }
      n51 = disable-structure shown="Enabled" {
        frame Disabled {
          # "Initialize the ILX to the front panel temperatures and currents for the on line and off line DBRs\nTurn on the TECs - does not turn on the lasers or set the Agiltron switches"
          n52 = call "ILX2.vi"("ILX Command"=T10."Initialize ILX") -> ("Device Out"=w60:refnum<visa-resource-name>)  [unwired: 10 in, 4 out]
          n53 = call "ILX2.vi"("Device In"=w60, "TEC Control"=TRUE, "ILX Command"=T10."TEC ON/OFF") -> ("Device Out"=w57:refnum<visa-resource-name>)  [unwired: 8 in, 4 out]
          n54 = flat-sequence {
            tunnel: w57 -> [w64]
            tunnel: [w64] -> w54
            frame #0 {
              # "Wait 30 seconds for\nthe ILX to stabilize"
              n55 = Wait (ms)(milliseconds to wait=u32 30000) -> ()  [unwired: 1 out]
            }
          }
          n56 = call "ILX2.vi"("Device In"=w54, "ILX Command"=T10."LASER ON/OFF", "Laser Control"=TRUE ("TEC Control")) -> ("Device Out"=w53:refnum<visa-resource-name>)  [unwired: 8 in, 4 out]
          n57 = flat-sequence {
            tunnel: w53 -> [w62]
            tunnel: [w62] -> _
            frame #0 {
              # "Wait 5 seconds for\nthe ILX to stabilize"
              n58 = Wait (ms)(milliseconds to wait=u32 5000) -> ()  [unwired: 1 out]
            }
          }
        }
        frame Enabled {
        }
      }
    }
    frame #2 {
      # "Active X commands to the Newport 1918-C"
      # "Set the  channel of\nthe Newport 1918-C"
      # "Set the operational mode\nof the Newport 1918-C"
      # "Open commumication\nto the Newport 1918-C"
      n59 = constructor class="PowerMeterCommands"("logging"="logging", "deviceKey"="NewportIn") -> (reference out=w94:refnum<k24>, error out=w91:errorcluster, "deviceKey"=w86:string)  [unwired: 3 in, 2 out]
      "Newport Device Key" <- w86
      n60 = invoke class="PowerMeterCommands" method="GetPower"(reference=w94, error in=w91, "deviceKey"=w86) -> (reference out=w93:refnum<k24>, error out=w90:errorcluster)  [unwired: 1 in, 2 out]
      n61 = invoke class="PowerMeterCommands" method="SetChannel"(reference=w93, error in=w90, "deviceKey"=w86, "channel"="1") -> (reference out=w87:refnum<k24>, error out=w89:errorcluster)  [unwired: 1 in, 3 out]
      n62 = invoke class="PowerMeterCommands" method="CmdGetPower"(reference=w87, error in=w89, "deviceKey"=w86, "power"=sgl 0.0) -> (reference out=→"NewportRef":refnum<k24>)  [unwired: 1 in, 4 out]
    }
    frame #3 {
      # "Clean up multiply and divide by powers of 10 with comments\nBMM 6/19/14"
      # "Generating an array that is 'Number of Bins' long, filled wih the relevant altitude values for later plotting of Range \nCorrected Returns"
      # "Generating an array that is 'Number of Bins' long, filled wih the relevant altitude values for later plotting of returns"
      # "Generate arrays for the altitude and range corrected return altitude.  To be used later for plotting purposes."
      n63 = local read "Time Resolution Per Bin(ns)"() -> (w107:u32)
      n64 = local read "Time Resolution Per Bin(ns)"() -> (w97:u32)
      n65 = local read "Number of Bins"() -> (w110:u32)
      n66 = local read "Number of Bins"() -> (w100:u32)
      n67 = Divide(x=w107, y=1000000000.0) -> (x/y=w105:dbl)
      n68 = Divide(x=w97, y=1000000000.0) -> (x/y=w95:dbl)
      n69 = Multiply(x=w105, y=150000.0) -> (x*y=w108:dbl)
      n70 = Initialize Array(0.0, 0) -> (w113:dbl[])
      n71 = Multiply(x=w95, y=150000000.0) -> (x*y=w98:dbl)
      n72 = Initialize Array(0.0, 0) -> (w103:dbl[])
      n73 = for {
        N: w110 -> [_]
        shift-right: [w126] -> w111
        shift-left: w113 -> [w127]
        tunnel: w108 -> [w123]
        i -> [w125]
        n74 = Multiply(x=w123, y=w125) -> (x*y=w124:dbl)
        n75 = Add(x=w124, y=w123) -> (x+y=w122:dbl)
        n76 = Build Array (concatenate)(w127, w122) -> (w126:dbl[])
      }
      "Altitude Array (km)" <- w111
      n77 = for {
        N: w100 -> [_]
        shift-right: [w120] -> w101
        shift-left: w103 -> [w121]
        tunnel: w98 -> [w116]
        i -> [w119]
        n78 = Multiply(x=w116, y=w119) -> (x*y=w117:dbl)
        n79 = Add(x=w117, y=w116) -> (x+y=w115:dbl)
        n80 = Multiply(x=w115, y=w115) -> (x*y=w118:dbl)
        n81 = Build Array (concatenate)(w121, w118) -> (w120:dbl[])
      }
      "Range Corrected Altitude Array" <- w101
      n82 = local write "Altitude Array (km)"(w111) -> ()
      n83 = local write "Range Corrected Altitude Array"(w101) -> ()
    }
    frame #4 {
      # "Frame 4: Collect data from the scaler card and process and file it"
      n84 = while {
        tunnel: ["stop"] -> w128
        i -> [w129]
        stop <- "stop" stop-if-true
        # "While loop continues data collection cycle"
        n85 = case shown="True" "Collect Data?" {
          frame False {
            # "If 'Collect Data?' is false, wait a ms and check the 'Collect Data?' value again"
            n86 = Wait (ms)(milliseconds to wait=u32 1) -> ()  [unwired: 1 out]
          }
          frame True {
            # "Frame 3: Read the offline wavelength and lock if necessary (code not finished), read output power, read offline data, perform calculations and plot/save offline and NRB data, switch to online\nFrame 4: Calculate the absorption cross section (if wavelength, T, or P changed)\nFrame 5: Calculate Water Vapor Number density and plot"
            # "Frame 0: Create folders and file paths for logging the data, initialize averaging index\nFrame 1: Import current pressure and temperature data from COE weather station\nFrame 2: Read the online wavelength and lock if necessary, read online data and output power\n, plot and save online data, switch to offline DBR"
            # "If 'Collect Data?' is true, collect, process, and log data"
            n87 = stacked-sequence {
              frame #0 {
                # "Looking to see if the current Yr/Mo/Dy/Hr folder exists\nin the data disk folder (E:\\Micropulse_DIAL_data), if not,\ncreate one for the data"
                n88 = local read "FileHour"() -> (w142:i32)
                n89 = Get Date/Time In Seconds() -> (seconds since 1Jan1904=w134:timestamp)
                n90 = Seconds To Date/Time(time stamp (now)=w134) -> (date time rec=w144:T14)  [unwired: 1 in]
                n91 = Unbundle By Name(w144) -> ("hour"=w133:i32)
                n92 = Equal?(x=w142, y=w133) -> (x = y?=w143:bool)
                n93 = case shown="True" "Reset Average" {
                  frame False {
                    n94 = local write "Index"(0 ("Index")) -> ()
                  }
                  frame True {
                    n95 = local read "Index"() -> (w232:i32)
                    n96 = Add(x=w232, y=1) -> (x+y=w231:i32)
                    n97 = local write "Index"(w231) -> ()
                  }
                }
                n98 = Format Date/Time String(time format string (%c)="%y%m%d", seconds (now)=w134) -> (date/time string=w138:string)  [unwired: 1 in]
                n99 = Concatenate Strings("Data File DIR (in)", w138, "FF" ("string")) -> (w140:string)
                n100 = Concatenate Strings("Data File DIR (in)", w138, "NF" ("string")) -> (w135:string)
                n101 = case shown="False" w143 {
                  tunnel: w140 -> [w202 _]
                  tunnel: w135 -> [w201 _]
                  tunnel: w134 -> [w188 _]
                  tunnel: w133 -> [w164 _]
                  frame False {
                    # "Are data files open?"
                    # "Within the \"E:\\Micropulse_DIAL_data...\n'Current month/day/year' \ncheck if the current hour folder exists,\nif not, create one"
                    n102 = local write "FileHour"(w164) -> ()
                    n103 = flat-sequence {
                      tunnel: [w222] -> w189
                      tunnel: w202 -> [w221]
                      tunnel: w201 -> [w222]
                      tunnel: [w221] -> w190
                      frame #0 {
                        # "Does \"E:\\Micropulse_DIAL_data...\n'Current month/day/year' exist?\nIf not, create a new folder with that name"
                        n104 = String To Path(string=w221) -> (path=w226:path)
                        n105 = String To Path(string=w222) -> (path=w224:path)
                        n106 = call <vilib>:"Check if File or Folder Exists.vi"("path"=w226) -> ("file or folder exists?"=w225:bool)  [unwired: 8 in, 2 out]
                        n107 = call <vilib>:"Check if File or Folder Exists.vi"("path"=w224) -> ("file or folder exists?"=w223:bool)  [unwired: 8 in, 2 out]
                        n108 = case shown="False" w225 {
                          tunnel: w226 -> [w228 _]
                          frame False {
                            # "create new folder"
                            n109 = Create Folder(path (use dialog)=w228) -> ()  [unwired: 2 in, 3 out]
                          }
                          frame True {
                            # "Folder exists\ndo nothing"
                          }
                        }
                        n110 = case shown="False" w223 {
                          tunnel: w224 -> [w227 _]
                          frame False {
                            # "create new folder"
                            n111 = Create Folder(path (use dialog)=w227) -> ()  [unwired: 2 in, 3 out]
                          }
                          frame True {
                            # "Folder exists\ndo nothing"
                          }
                        }
                      }
                    }
                    n112 = Concatenate Strings(w190, "\\" ("string")) -> (w197:string)
                    n113 = Concatenate Strings(w189, "\\" ("string")) -> (w192:string)
                    n114 = Format Date/Time String(time format string (%c)="%H", seconds (now)=w188) -> (date/time string=w200:string)  [unwired: 1 in]
                    n115 = Format Date/Time String(time format string (%c)="%H", seconds (now)=w188) -> (date/time string=w195:string)  [unwired: 1 in]
                    n116 = Concatenate Strings(w197, w200) -> (w160:string)
                    "File Path_Far Field (out)" <- w160
                    n117 = Concatenate Strings(w192, w195) -> (w161:string)
                    "File Path_Near Field (out)" <- w161
                    n118 = String To Path(string=w160) -> (path=w198:path)
                    n119 = String To Path(string=w161) -> (path=w193:path)
                    n120 = call <vilib>:"Check if File or Folder Exists.vi"("path"=w198) -> ("file or folder exists?"=w187:bool, "dup path"=w185:path)  [unwired: 8 in, 1 out]
                    n121 = call <vilib>:"Check if File or Folder Exists.vi"("path"=w193) -> ("file or folder exists?"=w186:bool, "dup path"=w184:path)  [unwired: 8 in, 1 out]
                    n122 = case shown="False" w187 {
                      tunnel: w185 -> [w219 _]
                      tunnel: w160 -> [w218 w220]
                      tunnel: [w218 w220] -> w158
                      frame False {
                        # "new folder"
                        n123 = Create Folder(path (use dialog)=w219) -> ()  [unwired: 2 in, 3 out]
                      }
                      frame True {
                        # "Folder exists\ndo nothing"
                      }
                    }
                    n124 = case shown="False" w186 {
                      tunnel: w184 -> [w216 _]
                      tunnel: w161 -> [w215 w217]
                      tunnel: [w215 w217] -> w159
                      frame False {
                        # "new folder"
                        n125 = Create Folder(path (use dialog)=w216) -> ()  [unwired: 2 in, 3 out]
                      }
                      frame True {
                        # "Folder exists\ndo nothing"
                      }
                    }
                    n126 = Concatenate Strings(w159, "\\Online_Raw_Data.dat" ("string")) -> (w178:string)
                    n127 = Concatenate Strings(w159, "\\Offline_Raw_Data.dat" ("string")) -> (w177:string)
                    n128 = Concatenate Strings(w158, "\\Online_Raw_Data.dat" ("string")) -> (w183:string)
                    n129 = Concatenate Strings(w158, "\\Offline_Raw_Data.dat" ("string")) -> (w182:string)
                    n130 = local read "DataOpen"() -> (w175:bool)
                    n131 = String To Path(string=w183) -> (path=w174:path)
                    n132 = String To Path(string=w182) -> (path=w173:path)
                    n133 = String To Path(string=w178) -> (path=w172:path)
                    n134 = String To Path(string=w177) -> (path=w171:path)
                    n135 = case shown="True" w175 {
                      tunnel: w174 -> [w206 w210]
                      tunnel: [w206 w210] -> w168
                      tunnel: w173 -> [w205 w209]
                      tunnel: [w205 w209] -> w167
                      tunnel: w172 -> [w204 w208]
                      tunnel: [w204 w208] -> w166
                      tunnel: [w203 w207] -> w165
                      tunnel: w171 -> [w203 w207]
                      frame False {
                        # "No files open\ndo nothing"
                      }
                      frame True {
                        # "Close open files"
                        n136 = local read "NF_Off_Ref"() -> (w212:refnum<file>)
                        n137 = local read "NF_On_Ref"() -> (w211:refnum<file>)
                        n138 = local read "FF_Off_Ref"() -> (w214:refnum<file>)
                        n139 = local read "FF_On_Ref"() -> (w213:refnum<file>)
                        n140 = Close File(refnum=w213) -> ()  [unwired: 1 in, 2 out]
                        n141 = Close File(refnum=w214) -> ()  [unwired: 1 in, 2 out]
                        n142 = Close File(refnum=w211) -> ()  [unwired: 1 in, 2 out]
                        n143 = Close File(refnum=w212) -> ()  [unwired: 1 in, 2 out]
                      }
                    }
                    n144 = Open/Create/Replace File(file path (use dialog)=w168, operation (0:open)=T11."open or create") -> (refnum out=w154:refnum<file>)  [unwired: 4 in, 2 out]
                    n145 = Open/Create/Replace File(file path (use dialog)=w167, operation (0:open)=T11."open or create") -> (refnum out=w155:refnum<file>)  [unwired: 4 in, 2 out]
                    n146 = Open/Create/Replace File(file path (use dialog)=w166, operation (0:open)=T11."open or create") -> (refnum out=w156:refnum<file>)  [unwired: 4 in, 2 out]
                    n147 = Open/Create/Replace File(file path (use dialog)=w165, operation (0:open)=T11."open or create") -> (refnum out=w157:refnum<file>)  [unwired: 4 in, 2 out]
                    n148 = Get File Size(file=w154) -> (refnum out=→"FF_On_Ref":refnum<file>, size (in bytes)=→"FF_On_Ptr":i64)  [unwired: 1 in, 1 out]
                    n149 = Get File Size(file=w155) -> (refnum out=→"FF_Off_Ref":refnum<file>, size (in bytes)=→"FF_Off_Ptr":i64)  [unwired: 1 in, 1 out]
                    n150 = Get File Size(file=w156) -> (refnum out=→"NF_On_Ref":refnum<file>, size (in bytes)=→"NF_On_Ptr":i64)  [unwired: 1 in, 1 out]
                    n151 = Get File Size(file=w157) -> (refnum out=→"NF_Off_Ref":refnum<file>, size (in bytes)=→"NF_Off_Ptr":i64)  [unwired: 1 in, 1 out]
                  }
                  frame True {
                    # "Don't need to do anything!"
                  }
                }
              }
              frame #1 {
                # "Writing and plotting retrieved\nweather parameters"
                # "Matlab script goes online and retrieves most recent press, temp, and relative humidity data \nfrom the weather station on the roof of Cobleigh"
                # "Importing the current weather conditions from the COE weather station"
                n152 = disable-structure shown="Disabled" {
                  frame Disabled {
                    n153 = script code="%try\n%s=urlread('http://www.coe.montana.edu/ee/weather/mostCurrentCSV.php');\n%amin=textscan(s,'%s %s %s %s %s %s %s %s %s %s %s %s %s');\n%data=amin{1}{2};\n%[test remain]=strtok(data,',');\n%remain=str2num(remain);\n%press=remain(3)./1000;\n%temp=remain(5);\n%RH=remain(7);\n%catch\npress=.850;\ntemp=20;\nRH=40;\n%end"() -> ()  [unwired: 1 in, 4 out]
                  }
                  frame Enabled {
                  }
                }
                n154 = local read "WS_On/Off"() -> (w233:bool)
                n155 = case shown="True" w233 {
                  frame False {
                  }
                  frame True {
                    n156 = local read "WS visa"() -> (w238:refnum<visa-resource-name>)
                    n157 = call "T_RH_P.vi"("VISA in"=w238, "WS_Commands"=enum16{"OpenWS", "ReadTRHP", "CloseWS"}."ReadTRHP") -> ("TRHP"=w234:T13)  [unwired: 11 in, 2 out]
                    n158 = local write "TRHP"(w234) -> ()
                    n159 = Unbundle By Name(w234) -> ("Temp"=→"Temperature (C)":dbl, "RelH"=→"Relative Humdity (%)":dbl, "Press"=→"Pressure (mb)":dbl)
                  }
                }
              }
              frame #2 {
                # "Frame 3: Read, process, and plot online data\nFrame 4:\nFrame 5: Write the data to the folders from Frame 0 of outter sequence"
                # "Frame 0: Read the online wavelength and adjust to locking tolerance if out of range, Switch to offline DBR\nFrame 1: Read the output power from the Newport meter, calculate and plot the output pulse energy\nFrame 2: Wait 'Scalar Wait Time' for buffer to clear other wavelength data"
                # "Online"
                n160 = stacked-sequence {
                  frame #0 {
                    # "Read the online wavelength and continue adjusting the online DBR if outside the wavelength tolerance\nuntil it is within tolerance"
                    n161 = while {
                      i -> [w241]
                      stop <- w240 stop-if-true
                      # "Frame 2: Decrement DBR current if above tolerance\nFrame 3: Increment DBR current if below tolerance"
                      # "Frame 0: Read the current wavelength from the wavemeter\nFrame 1: Calculate the difference between desired and actual wavelength"
                      # "Continue reading and adjusting online DBR current until within locking tolerance"
                      n162 = stacked-sequence {
                        tunnel: w241 -> [w243 _ _ _ _]
                        tunnel: [_ _ w259 _ _] -> w240
                        frame #0 {
                          n163 = Equal To 0?(x=w243) -> (x = 0?=w242:bool)
                          n164 = case shown="True" w242 {
                            frame False {
                            }
                            frame True {
                              # "Set the wavemeter switch to WV Online"
                              n165 = flat-sequence {
                                frame #0 {
                                n166 = Build Array(FALSE ("Boolean")) -> (w246:bool[])
                                n167 = call-poly <vilib>:"DAQmx Write.vi"("task/channels in"=refnum<k21> "BristolWM", "data"=w246) -> ()  [unwired: 11 in, 3 out]
                                }
                                frame #1 {
                                n168 = Build Array(FALSE ("Boolean")) -> (w249:bool[])
                                n169 = call-poly <vilib>:"DAQmx Write.vi"("task/channels in"=refnum<k21> "HSRL_WV_switch", "data"=w249) -> ()  [unwired: 11 in, 3 out]
                                }
                              }
                            }
                          }
                        }
                        frame #1 {
                          # "Reading the wavelength from the wavemeter"
                          n170 = flat-sequence {
                            tunnel: [w252] -> w251
                            tunnel: w251 -> [w255]
                            tunnel: [w254] -> w250
                            tunnel: w250 -> [w258]
                            frame #0 {
                              n171 = local read "Bristol In"() -> (w253:i32)
                              n172 = dll-call lib="C:/Users/H2ODial/Desktop/Shared Telescope WV DIAL Code/bristol/CLDevIface.dll" fn="CLOpenUSBSerialDevice"("commPort"=w253) -> ("return type"=w252:i32)  [unwired: 4 in, 2 out]
                            }
                            frame #1 {
                              n173 = dll-call lib="C:/Users/H2ODial/Desktop/Shared Telescope WV DIAL Code/bristol/CLDevIface.dll" fn="CLGetLambdaReading"("devHandle"=w255) -> ("return type"=→"WV Online Read (nm)":dbl, "devHandle"=w254:i32)  [unwired: 3 in, 2 out]
                            }
                            frame #2 {
                              n174 = dll-call lib="C:/Users/H2ODial/Desktop/Shared Telescope WV DIAL Code/bristol/CLDevIface.dll" fn="CLCloseDevice"("commPort"=w258) -> ("return type"=w257:i32)  [unwired: 4 in, 2 out]
                              n175 = local write "Bristol Out"(w257) -> ()
                            }
                          }
                        }
                        frame #2 {
                          # "If WL difference is within tolerance, stop looping, and illuminate 'Wavelength Lock Online' indicator"
                          # "Calculating the difference between the actual and desired online wavelength"
                          n176 = local read "WV Online Read (nm)"() -> (w262:dbl)
                          n177 = local read "Online_Tol"() -> (w267:dbl)
                          n178 = Multiply(x=-1.0, y=w267) -> (x*y=w268:dbl)
                          n179 = Subtract(x=w262, y="WV Online Set (nm)") -> (x-y=w263:dbl)
                          "Online_Diff" <- w263
                          n180 = Greater?(x=w263, y=w268) -> (0:w264:bool)
                          n181 = Less?(x=w263, y=w267) -> (x < y?=w265:bool)
                          n182 = And(x=w264, y=w265) -> (x .and. y?=w261:bool)
                          "WV Online Locked" <- w261
                          n183 = Or(x=w261, y="Cancel online") -> (x .or. y?=w259:bool)
                        }
                        frame #3 {
                          # "If the wavelength difference is greater that 0.0002 nm, decrement the \nDBR current by 0.01 mA"
                          n184 = local read "Online_Diff"() -> (w272:dbl)
                          n185 = Greater Or Equal?(x=w272, y="Online_Tol") -> (x >= y?=w271:bool)
                          n186 = case shown="True" w271 {
                            frame False {
                              # "Wavelength difference is not greater than 0.0002 nm, do nothing"
                            }
                            frame True {
                              # "Generating a command string\nto decrement the current"
                              # "WL difference is greater than 0.0002 nm,\ndecrement the DBR current by 0.01 mA"
                              n187 = local read "Settings"() -> (w279:T6)
                              n188 = local read "temp step size"() -> (w274:dbl)
                              n189 = Unbundle By Name(w279) -> ("WV Online TEC"=w278:dbl)
                              n190 = local read "Device In"() -> (w275:refnum<visa-resource-name>)
                              n191 = Subtract(x=w278, y=w274) -> (x-y=w277:dbl)
                              n192 = Bundle By Name(cluster=w279, "WV Online TEC"=w277, "Module"=T12."WV Online TEC") -> (w281:T6)
                              n193 = call "TL_Driver_v2.vi"("Device In"=w275, "Commands"=T9."SET", "Settings"=w281) -> ("Readings"=w280:T7)  [unwired: 9 in, 3 out]
                              n194 = local write "Settings"(w281) -> ()
                              n195 = local write "Readings"(w280) -> ()
                            }
                          }
                        }
                        frame #4 {
                          # "If WL difference is < 0.0002 nm, increment the DBR current"
                          n196 = local read "Online_Tol"() -> (w283:dbl)
                          n197 = local read "Online_Diff"() -> (w286:dbl)
                          n198 = Multiply(x=-1.0, y=w283) -> (x*y=w282:dbl)
                          n199 = Less Or Equal?(x=w286, y=w282) -> (x <= y?=w285:bool)
                          n200 = case shown="True" w285 {
                            frame False {
                              # "WL difference is no <= to -0.0002 nm, do nothing"
                            }
                            frame True {
                              # "WL difference is < -0.0002,\nincrement the DBR current by 0.01 mA"
                              # "Generating a command string\nto decrement the current"
                              n201 = local read "Settings"() -> (w295:T6)
                              n202 = local read "temp step size"() -> (w288:dbl)
                              n203 = Unbundle By Name(w295) -> ("WV Online TEC"=w292:dbl)
                              n204 = local read "Device In"() -> (w289:refnum<visa-resource-name>)
                              n205 = Add(x=w292, y=w288) -> (x+y=w291:dbl)
                              n206 = Bundle By Name(cluster=w295, "WV Online TEC"=w291, "Module"=T12."WV Online TEC") -> (w294:T6)
                              n207 = call "TL_Driver_v2.vi"("Device In"=w289, "Commands"=T9."SET", "Settings"=w294) -> ("Readings"=w293:T7)  [unwired: 9 in, 3 out]
                              n208 = local write "Settings"(w294) -> ()
                              n209 = local write "Readings"(w293) -> ()
                            }
                          }
                        }
                      }
                    }
                  }
                  frame #1 {
                    # "Converting to pulse energy, assumes 5 percent pickoff"
                    # "Reading the Newport Power meter"
                    # "Reading the output power of the laser transmitter from the Newport power meter, once read, convert to corresponding pulse energy and plot"
                    n210 = local read "Newport Device Key"() -> (w300:string)
                    n211 = local read "NewportRef"() -> (w296:refnum<k24>)
                    n212 = disable-structure shown="Enabled" {
                      frame Enabled {
                        # "Plotting the online and offling pulse energies"
                        n213 = local read "Online Pulse Energy"() -> (w311:dbl)
                        n214 = local read "Offline Pulse Energy"() -> (w310:dbl)
                        n215 = Bundle("Online Pulse Energy"=w311, "Offline Pulse Energy"=w310) -> (→"Pulse Energy (Micro Joule)":T15)  [unwired: 1 in]
                      }
                      frame Disabled {
                      }
                    }
                    n216 = Number To Decimal String(number="SampleSize") -> (decimal integer string=w298:string)  [unwired: 1 in]
                    n217 = invoke class="PowerMeterCommands" method="PerformDAQ"(reference=w296, "deviceKey"=w300, "interval"="1", "sampleSize"=w298) -> ("PerformDAQ"=w301:dbl[])  [unwired: 2 in, 5 out]
                    n218 = call-poly <vilib>:"Mean.vi"("X"=w301) -> ("mean"=w299:dbl)  [unwired: 1 out]
                    n219 = Multiply(x=w299, y=1000.0) -> (x*y=w307:dbl)
                    n220 = Divide(x=w307, y=0.05) -> (x/y=w305:dbl)
                    n221 = Divide(x=w305, y=7.0) -> (x/y=→"Online Pulse Energy":dbl)
                  }
                  frame #2 {
                    # "Wait 'Scalar Wait Time' for the next available batch of scalar card data"
                    n222 = local read "AMCS_Profile"() -> (w312:i32)
                    n223 = disable-structure shown="Disabled" {
                      frame Disabled {
                        # "Waiting 'Scalar Wait Time'"
                        n224 = Wait (ms)(milliseconds to wait="Scalar Wait Time") -> ()  [unwired: 1 out]
                      }
                      frame Enabled {
                      }
                    }
                    n225 = while {
                      tunnel: [w319] -> w313
                      tunnel: [w315] -> _
                      tunnel: w312 -> [w315]
                      stop <- w317 stop-if-true
                      n226 = global read "AMCS_Data.vi" "AMCS_Profile"() -> (w319:i32)
                      n227 = Wait (ms)(milliseconds to wait=u32 10) -> ()  [unwired: 1 out]
                      n228 = Equal?(x=w319, y=w315) -> (x = y?=w318:bool)
                      n229 = case shown="False" w318 {
                        tunnel: [TRUE FALSE] -> w317
                        frame False {
                        }
                        frame True {
                        }
                      }
                    }
                    "AMCS_Profile" <- w313
                  }
                  frame #3 {
                    # "convert time per range bin to meters\nand calculate smoothed bins using\nsmoothing range"
                    # "Plotting online cross section and smoothed online data"
                    # "Calculate the bin by bin mean of the data"
                    # "Collect 'Integration Period (Seconds)' number\nof scalar data"
                    # "Reading, processing, and plotting the online data"
                    n230 = local read "Data Reads (number of loops)"() -> (w347:i32)
                    n231 = for {
                      N: w347 -> [_]
                      tunnel: [w368] -> w359 mode=indexing
                      tunnel: [w367] -> w322 mode=indexing
                      # "Scalar Data is retrieved from Global \nVariable that scaler.vi is writing to,"
                      n232 = global read "AMCS_Data.vi" "AMCS_Data"() -> (w371:u16[][])
                      n233 = disable-structure shown="Disabled" {
                        frame Disabled {
                          n234 = global read "Scalar_Data_3.vi" "Scalar Data 3"() -> ()  [unwired: 1 out]
                          n235 = global read "Scalar_Data.vi" "Scalar Data"() -> ()  [unwired: 1 out]
                        }
                        frame Enabled {
                        }
                      }
                      n236 = Index Array(array=w371, index (row) #1=0 ("index (row)"), index (row) #2=2 ("index (row)")) -> (element #1=w368:u16[], element #2=w367:u16[])  [unwired: 2 in]
                    }
                    n237 = Transpose 2D Array(2D array=w359) -> (transposed array=w363:u16[][])
                    n238 = Transpose 2D Array(2D array=w322) -> (transposed array=w345:u16[][])
                    n239 = for {
                      tunnel: w363 -> [w373] mode=indexing
                      tunnel: [w372] -> w364 mode=indexing
                      n240 = call-poly <vilib>:"Mean.vi"("X"=w373) -> ("mean"=w372:dbl)  [unwired: 1 out]
                    }
                    n241 = for {
                      tunnel: w345 -> [w366] mode=indexing
                      tunnel: [w365] -> w346 mode=indexing
                      n242 = call-poly <vilib>:"Mean.vi"("X"=w366) -> ("mean"=w365:dbl)  [unwired: 1 out]
                    }
                    n243 = local read "bins"() -> (w339:u32)
                    n244 = Array Subset(array=w364, index=1 ("dimension size"), length=w339) -> (w351:dbl[])
                    n245 = Array Subset(array=w346, index=1 ("dimension size"), length=w339) -> (w343:dbl[])
                    n246 = local read "background length"() -> (w329:i32)
                    n247 = local read "background start"() -> (w330:u32)
                    n248 = Array Size(array=w351) -> (size(s)=w348:i32)
                    n249 = Array Size(array=w343) -> (size(s)=w340:i32)
                    n250 = Initialize Array(1.0 ("element"), w348) -> (w350:dbl[])
                    n251 = Initialize Array(1.0 ("element"), w340) -> (w342:dbl[])
                    n252 = Multiply(x=w351, y=w350) -> (x*y=w352:dbl[])
                    "CH 0 Bin Readings" <- w352
                    n253 = Multiply(x=w343, y=w342) -> (x*y=w333:dbl[])
                    "CH 2 Bin Readings" <- w333
                    n254 = local read "Total DIAL Integration Time (Minutes)"() -> (w355:i32)
                    n255 = local read "Time Resolution Per Bin(ns)"() -> (w325:u32)
                    n256 = Array Subset(array=w352, index=w330, length=w329) -> (w361:dbl[])
                    n257 = Array Subset(array=w333, index=w330, length=w329) -> (w335:dbl[])
                    n258 = call-poly <vilib>:"Mean.vi"("X"=w361) -> ("mean"=w360:dbl)  [unwired: 1 out]
                    n259 = call-poly <vilib>:"Mean.vi"("X"=w335) -> ("mean"=w336:dbl)  [unwired: 1 out]
                    n260 = Divide(x=w355, y=w347) -> (x/y=w353:dbl)
                    n261 = local read "Index"() -> (w334:i32)
                    n262 = Subtract(x=w352, y=w360) -> (x-y=w357:dbl[])
                    n263 = Subtract(x=w333, y=w336) -> (x-y=w337:dbl[])
                    n264 = To Double Precision Float(number=w325) -> (double precision float=w326:dbl)
                    n265 = Multiply(x=w353, y=60.0) -> (x*y=w331:dbl)
                    n266 = Multiply(x=w326, y=0.15) -> (x*y=w328:dbl)
                    n267 = call "Ring Buffer CH2 rev2.vi"("Index"=w334, "Profiles to Average"=w331, "Input Array"=w337) -> ("AvgArray"=w338:dbl[])  [unwired: 7 in, 1 out]
                    n268 = call "Ring Buffer CH0 rev2.vi"("Index"=w334, "Profiles to Average"=w331, "Input Array"=w357) -> ("AvgArray"=w356:dbl[])  [unwired: 7 in, 1 out]
                    n269 = Divide(x="Smoothing Range", y=w328) -> (x/y=w323:dbl)
                    "Smoothed Bins" <- w323
                    n270 = call "Smooth Arrray.vi"("smooth size"=w323, "Raw Array"=w356) -> ("Smoothed Array"=→"CH0 (WV on) smoothed":dbl[])  [unwired: 9 in]
                    n271 = call "Smooth Arrray.vi"("smooth size"=w323, "Raw Array"=w338) -> ("Smoothed Array"=→"CH2 (molecular) smoothed":dbl[])  [unwired: 9 in]
                    n272 = disable-structure shown="Disabled" {
                      frame Disabled {
                        n273 = script code="format long;\ncounts=sum(Online);\nif counts >=0.5e6\ntime=time;\nelse\ntime=time\nend"() -> ()  [unwired: 3 in, 2 out]
                      }
                      frame Enabled {
                      }
                    }
                  }
                  frame #4 {
                    # "Toggling the Agiltron switch to the offline DBR seed laser"
                    n274 = disable-structure shown="Disabled" {
                      frame Disabled {
                        n275 = flat-sequence {
                          frame #0 {
                            # "Second one"
                            # "Command the switch to switch to position 2\ncorresponding to the offline DBR"
                            # "Hex string command \ncorrespond to offline"
                            n276 = VISA Write(VISA resource name="Switch Comm Port", write buffer="\u0001\u0012\u0000\u0001") -> ()  [unwired: 1 in, 3 out]
                          }
                        }
                      }
                      frame Enabled {
                      }
                    }
                  }
                  frame #5 {
                    # "Save the recently collected online data if 'Save Data?' is true"
                    n277 = case shown="True" "Save Data?" {
                      frame False {
                        # "'Save Data?' is false, do nothing"
                      }
                      frame True {
                        # "'Save Data?' is true, save onfline data to the Data Disk"
                        # "Write only one copy of data at this time"
                        # "Retrieve Julian Date"
                        n278 = local read "Readings"() -> (w379:T7)
                        n279 = local read "Time Resolution Per Bin(ns)"() -> (w387:u32)
                        n280 = Unbundle By Name(w379) -> ("WV OnLine TEC"=w378:dbl)
                        n281 = local read "Number of Accumulates"() -> (w385:u32)
                        n282 = Unbundle By Name(w379) -> ("HSRL TEC"=w377:dbl)
                        n283 = local read "WV Online Read (nm)"() -> (w380:dbl)
                        n284 = local write "DataOpen"(TRUE ("DataOpen")) -> ()
                        n285 = local read "Number of Bins"() -> (w386:u32)
                        n286 = local read "HSRL Read (nm)"() -> (w381:dbl)
                        n287 = local read "Online Pulse Energy"() -> (w408:dbl)
                        n288 = local read "CH 0 Bin Readings"() -> (w410:dbl[])
                        n289 = To Double Precision Float(number=w387) -> (double precision float=w382:dbl)
                        n290 = To Double Precision Float(number=w386) -> (double precision float=w383:dbl)
                        n291 = To Double Precision Float(number=w385) -> (double precision float=w384:dbl)
                        n292 = local read "CH 2 Bin Readings"() -> (w407:dbl[])
                        n293 = call "Julian_Date_2.vi"() -> ("Julian Date"=w409:dbl)  [unwired: 11 in]
                        n294 = Build Array (concatenate)(w409, w380, w378, w408, w382, w383, w384, w410) -> (w402:dbl[])
                        n295 = Build Array (concatenate)(w409, w381, w377, w408, w382, w383, w384, w407) -> (w392:dbl[])
                        n296 = local read "NF_On_Ref"() -> (w390:refnum<file>)
                        n297 = local read "FF_On_Ref"() -> (w406:refnum<file>)
                        n298 = local read "NF_On_Ptr"() -> (w391:i64)
                        n299 = local read "FF_On_Ptr"() -> (w405:i64)
                        n300 = Set File Position(offset (in bytes) (0)=w405, refnum=w406) -> (refnum out=w403:refnum<file>, error out=w400:errorcluster)  [unwired: 2 in]
                        n301 = Set File Position(offset (in bytes) (0)=w391, refnum=w390) -> (refnum out=w396:refnum<file>, error out=w394:errorcluster)  [unwired: 2 in]
                        n302 = Write to Binary File(file (use dialog)=w396, data=w392, error in=w394, 5:FALSE ("prepend array or string size? (T)")) -> (refnum out=w395:refnum<file>, error out=w393:errorcluster)  [unwired: 2 in, 1 out]
                        n303 = Write to Binary File(file (use dialog)=w403, data=w402, error in=w400, 5:FALSE ("prepend array or string size? (T)")) -> (refnum out=w401:refnum<file>, error out=w399:errorcluster)  [unwired: 2 in, 1 out]
                        n304 = Get File Position(4:w393, 7:w395) -> (2:w389:i64)  [unwired: 2 out]
                        n305 = Get File Position(4:w399, 7:w401) -> (2:w398:i64)  [unwired: 2 out]
                        n306 = local write "NF_On_Ptr"(w389) -> ()
                        n307 = local write "FF_On_Ptr"(w398) -> ()
                      }
                    }
                  }
                }
              }
              frame #3 {
                # "Frame 3: Read offline data, calculate aerosol data, and plot offline and normalized relative backscatter\nFrame 4:\nFrame 5: Save the offline data and related information"
                # "Frame 0: Read the offline wavelength and lock if necessary, Switch to online DBR\nFrame 1: Read the output power from the Newport power meter\nFrame 2: Wait 'Scalar Wait Time' for buffers to clear of online contiminated data"
                # "offline"
                n308 = stacked-sequence {
                  frame #0 {
                    # "Following Locking the Offline wavelength, check and lock the HSRL 780 nm wavelength"
                    # "Every 60 data collection cycles, read the offline DBR wavelength, and if outside of wavelength tolerance, adjust DBR current until within tolerance"
                    n309 = local read "L_Count"() -> (w412:i32)
                    n310 = Quotient & Remainder(x=w412, y=60.0) -> (x-y*floor(x/y)=w413:dbl)  [unwired: 1 out]
                    n311 = Equal To 0?(x=w413) -> (x = 0?=w411:bool)
                    n312 = case shown="True" w411 {
                      frame False {
                      }
                      frame True {
                        n313 = flat-sequence {
                          frame #0 {
                            n314 = while {
                              i -> [w418]
                              stop <- w416 stop-if-true
                              # "If WL difference is within tolerance, stop looping, and illuminate 'Wavelength Lock Offline' indicator"
                              # "Frame 2: Decrement DBR if above tolerance\nFrame 3: Increment DBR if below tolerance"
                              # "Frame 0: Read the wavelength from the wavemeter\nFrame 1: Calculate the difference between desired and actual wavelength"
                              # "Continue reading and adjusting offline DBR until within locking tolerance"
                              n315 = stacked-sequence {
                                tunnel: w418 -> [w420 _ _ _ _]
                                tunnel: [_ _ w434 _ _] -> w415
                                frame #0 {
                                n316 = Equal To 0?(x=w420) -> (x = 0?=w419:bool)
                                n317 = case shown="True" w419 {
                                frame False {
                                }
                                frame True {
                                # "Set the TSOA switch to\namplify the offline wavelength"
                                n318 = Build Array(TRUE ("Boolean")) -> (w422:bool[])
                                n319 = call-poly <vilib>:"DAQmx Write.vi"("task/channels in"=refnum<k21> "BristolWM", "data"=w422) -> ()  [unwired: 11 in, 3 out]
                                n320 = Wait (ms)(milliseconds to wait=u32 3200) -> ()  [unwired: 1 out]
                                }
                                }
                                }
                                frame #1 {
                                # "Reading the wavelength from the wavemeter"
                                n321 = flat-sequence {
                                tunnel: [w427] -> w426
                                tunnel: w426 -> [w430]
                                tunnel: [w429] -> w425
                                tunnel: w425 -> [w433]
                                frame #0 {
                                n322 = local read "Bristol In"() -> (w428:i32)
                                n323 = dll-call lib="C:/Users/H2ODial/Desktop/Shared Telescope WV DIAL Code/bristol/CLDevIface.dll" fn="CLOpenUSBSerialDevice"("commPort"=w428) -> ("return type"=w427:i32)  [unwired: 4 in, 2 out]
                                }
                                frame #1 {
                                n324 = dll-call lib="C:/Users/H2ODial/Desktop/Shared Telescope WV DIAL Code/bristol/CLDevIface.dll" fn="CLGetLambdaReading"("devHandle"=w430) -> ("return type"=→"WV Offline Read (nm)":dbl, "devHandle"=w429:i32)  [unwired: 3 in, 2 out]
                                }
                                frame #2 {
                                n325 = dll-call lib="C:/Users/H2ODial/Desktop/Shared Telescope WV DIAL Code/bristol/CLDevIface.dll" fn="CLCloseDevice"("commPort"=w433) -> ("return type"=w432:i32)  [unwired: 4 in, 2 out]
                                n326 = local write "Bristol Out"(w432) -> ()
                                }
                                }
                                }
                                frame #2 {
                                # "Calculating the difference between the actual and desired online wavelength"
                                n327 = local read "Offline_Tol"() -> (w436:dbl)
                                n328 = local read "WV Offline Read (nm)"() -> (w442:dbl)
                                n329 = Multiply(x=-1.0, y=w436) -> (x*y=w435:dbl)
                                n330 = Subtract(x=w442, y="WV Offline Set (nm)") -> (x-y=w438:dbl)
                                "Oflline_Diff" <- w438
                                n331 = Greater?(x=w438, y=w435) -> (0:w439:bool)
                                n332 = Less?(x=w438, y=w436) -> (x < y?=w440:bool)
                                n333 = And(x=w439, y=w440) -> (x .and. y?=w434:bool)
                                "WV Oflline Locked" <- w434
                                n334 = case shown="True" w434 {
                                frame False {
                                }
                                frame True {
                                # "Set the Wavemeter switch to\nthe HSRL wavelength"
                                n335 = Build Array(TRUE ("Boolean")) -> (w444:bool[])
                                n336 = call-poly <vilib>:"DAQmx Write.vi"("task/channels in"=refnum<k21> "HSRL_WV_switch", "data"=w444) -> ()  [unwired: 11 in, 3 out]
                                n337 = Wait (ms)(milliseconds to wait=u32 3200) -> ()  [unwired: 1 out]
                                }
                                }
                                }
                                frame #3 {
                                # "If the wavelength difference is greater that 0.0002 nm, decrement the \nDBR current by 0.01 mA"
                                n338 = local read "Oflline_Diff"() -> (w449:dbl)
                                n339 = Greater Or Equal?(x=w449, y="Offline_Tol") -> (x >= y?=w448:bool)
                                n340 = case shown="True" w448 {
                                frame False {
                                # "Wavelength difference is not greater than 0.0002 nm, do nothing"
                                }
                                frame True {
                                # "Generating a command string\nto decrement the current"
                                n341 = local read "Settings"() -> (w456:T6)
                                n342 = Unbundle By Name(w456) -> ("WV Offline TEC"=w454:dbl)
                                n343 = Subtract(x=w454, y="temp step size") -> (x-y=w453:dbl)
                                n344 = local read "Device In"() -> (w451:refnum<visa-resource-name>)
                                n345 = Bundle By Name(cluster=w456, "WV Offline TEC"=w453, "Module"=T12."WV Offline TEC") -> (w457:T6)
                                n346 = call "TL_Driver_v2.vi"("Device In"=w451, "Commands"=T9."SET", "Settings"=w457) -> ("Readings"=w458:T7)  [unwired: 9 in, 3 out]
                                n347 = local write "Settings"(w457) -> ()
                                n348 = local write "Readings"(w458) -> ()
                                }
                                }
                                }
                                frame #4 {
                                # "If WL difference is < 0.0002 nm, increment the DBR temperature"
                                n349 = local read "Oflline_Diff"() -> (w461:dbl)
                                n350 = Less Or Equal?(x=w461, y=-0.0001) -> (x <= y?=w459:bool)
                                n351 = case shown="True" w459 {
                                frame False {
                                # "WL difference is no <= to -0.0002 nm, do nothing"
                                }
                                frame True {
                                # "Generating a command string\nto decrement the current"
                                # "WL difference is less than 0.0002 nm,\nincrement the DBR current by 0.01 mA"
                                n352 = local read "Settings"() -> (w469:T6)
                                n353 = Unbundle By Name(w469) -> ("WV Offline TEC"=w467:dbl)
                                n354 = local read "temp step size"() -> (w463:dbl)
                                n355 = Add(x=w467, y=w463) -> (x+y=w466:dbl)
                                n356 = local read "Device In"() -> (w464:refnum<visa-resource-name>)
                                n357 = Bundle By Name(cluster=w469, "WV Offline TEC"=w466, "Module"=T12."WV Offline TEC") -> (w470:T6)
                                n358 = call "TL_Driver_v2.vi"("Device In"=w464, "Commands"=T9."SET", "Settings"=w470) -> ("Readings"=w468:T7)  [unwired: 9 in, 3 out]
                                n359 = local write "Settings"(w470) -> ()
                                n360 = local write "Readings"(w468) -> ()
                                }
                                }
                                }
                              }
                              n361 = Or(x=w415, y="Cancel Offline") -> (x .or. y?=w416:bool)
                            }
                          }
                          frame #1 {
                            n362 = while {
                              i -> [w474]
                              stop <- w472 stop-if-true
                              # "If WL difference is within tolerance, stop looping, and illuminate 'Wavelength Lock Offline' indicator"
                              # "Frame 2: Decrement DBR if above tolerance\nFrame 3: Increment DBR if below tolerance"
                              # "Frame 0: Read the wavelength from the wavemeter\nFrame 1: Calculate the difference between desired and actual wavelength"
                              # "Continue reading and adjusting offline DBR until within locking tolerance"
                              n363 = stacked-sequence {
                                tunnel: w474 -> [w476 _ _ _ _]
                                tunnel: [_ _ w489 _ _] -> w471
                                frame #0 {
                                n364 = Equal To 0?(x=w476) -> (x = 0?=w475:bool)
                                n365 = case shown="True" w475 {
                                frame False {
                                }
                                frame True {
                                # "Set the Wavemeter to\nthe non HSRL wavelength"
                                n366 = Build Array(TRUE ("Boolean")) -> (w477:bool[])
                                n367 = call-poly <vilib>:"DAQmx Write.vi"("task/channels in"=refnum<k21> "HSRL_WV_switch", "data"=w477) -> ()  [unwired: 11 in, 3 out]
                                }
                                }
                                }
                                frame #1 {
                                # "Reading the wavelength from the wavemeter"
                                n368 = flat-sequence {
                                tunnel: [w482] -> w481
                                tunnel: w481 -> [w485]
                                tunnel: [w484] -> w480
                                tunnel: w480 -> [w488]
                                frame #0 {
                                n369 = local read "Bristol In"() -> (w483:i32)
                                n370 = dll-call lib="C:/Users/H2ODial/Desktop/Shared Telescope WV DIAL Code/bristol/CLDevIface.dll" fn="CLOpenUSBSerialDevice"("commPort"=w483) -> ("return type"=w482:i32)  [unwired: 4 in, 2 out]
                                }
                                frame #1 {
                                n371 = dll-call lib="C:/Users/H2ODial/Desktop/Shared Telescope WV DIAL Code/bristol/CLDevIface.dll" fn="CLGetLambdaReading"("devHandle"=w485) -> ("return type"=→"HSRL Read (nm)":dbl, "devHandle"=w484:i32)  [unwired: 3 in, 2 out]
                                }
                                frame #2 {
                                n372 = dll-call lib="C:/Users/H2ODial/Desktop/Shared Telescope WV DIAL Code/bristol/CLDevIface.dll" fn="CLCloseDevice"("commPort"=w488) -> ("return type"=w487:i32)  [unwired: 4 in, 2 out]
                                n373 = local write "Bristol Out"(w487) -> ()
                                }
                                }
                                }
                                frame #2 {
                                # "Calculating the difference between the actual and desired online wavelength"
                                n374 = local read "HSRL_Tol"() -> (w491:dbl)
                                n375 = local read "HSRL Read (nm)"() -> (w497:dbl)
                                n376 = Multiply(x=-1.0, y=w491) -> (x*y=w490:dbl)
                                n377 = Subtract(x=w497, y="HSRL Set (nm)") -> (x-y=w493:dbl)
                                "HSRL_Diff" <- w493
                                n378 = Greater?(x=w493, y=w490) -> (0:w494:bool)
                                n379 = Less?(x=w493, y=w491) -> (x < y?=w495:bool)
                                n380 = And(x=w494, y=w495) -> (x .and. y?=w489:bool)
                                "HSRL Locked" <- w489
                                n381 = case shown="True" w489 {
                                frame False {
                                }
                                frame True {
                                # "Set the Wavementer switch to WV Online"
                                n382 = Build Array(FALSE ("Boolean")) -> (w499:bool[])
                                n383 = Build Array(FALSE ("Boolean")) -> (w503:bool[])
                                n384 = call-poly <vilib>:"DAQmx Write.vi"("task/channels in"=refnum<k21> "BristolWM", "data"=w503) -> ("error out"=w498:errorcluster)  [unwired: 11 in, 2 out]
                                n385 = call-poly <vilib>:"DAQmx Write.vi"("task/channels in"=refnum<k21> "HSRL_WV_switch", "data"=w499, "error in"=w498) -> ()  [unwired: 10 in, 3 out]
                                n386 = Wait (ms)(milliseconds to wait=u32 3200) -> ()  [unwired: 1 out]
                                }
                                }
                                }
                                frame #3 {
                                # "If the wavelength difference is greater that 0.0002 nm, decrement the \nDBR current by 0.01 mA"
                                n387 = local read "HSRL_Diff"() -> (w508:dbl)
                                n388 = Greater Or Equal?(x=w508, y="HSRL_Tol") -> (x >= y?=w507:bool)
                                n389 = case shown="True" w507 {
                                frame False {
                                # "Wavelength difference is not greater than 0.0002 nm, do nothing"
                                }
                                frame True {
                                # "Generating a command string\nto decrement the current"
                                n390 = local read "Settings"() -> (w515:T6)
                                n391 = local read "temp step size"() -> (w509:dbl)
                                n392 = Unbundle By Name(w515) -> ("HSRL TEC"=w514:dbl)
                                n393 = Subtract(x=w514, y=w509) -> (x-y=w513:dbl)
                                n394 = local read "Device In"() -> (w511:refnum<visa-resource-name>)
                                n395 = Bundle By Name(cluster=w515, "HSRL TEC"=w513, "Module"=T12."HSRL TEC") -> (w516:T6)
                                n396 = call "TL_Driver_v2.vi"("Device In"=w511, "Commands"=T9."SET", "Settings"=w516) -> ("Readings"=w517:T7)  [unwired: 9 in, 3 out]
                                n397 = local write "Settings"(w516) -> ()
                                n398 = local write "Readings"(w517) -> ()
                                }
                                }
                                }
                                frame #4 {
                                # "If WL difference is < 0.0002 nm, increment the DBR temperature"
                                n399 = local read "HSRL_Diff"() -> (w520:dbl)
                                n400 = Less Or Equal?(x=w520, y=-0.0001) -> (x <= y?=w518:bool)
                                n401 = case shown="True" w518 {
                                frame False {
                                # "WL difference is no <= to -0.0002 nm, do nothing"
                                }
                                frame True {
                                # "Generating a command string\nto decrement the current"
                                # "WL difference is less than 0.0002 nm,\nincrement the DBR current by 0.01 mA"
                                n402 = local read "Settings"() -> (w528:T6)
                                n403 = local read "temp step size"() -> (w521:dbl)
                                n404 = Unbundle By Name(w528) -> ("HSRL TEC"=w526:dbl)
                                n405 = Add(x=w526, y=w521) -> (x+y=w525:dbl)
                                n406 = local read "Device In"() -> (w523:refnum<visa-resource-name>)
                                n407 = Bundle By Name(cluster=w528, "HSRL TEC"=w525, "Module"=T12."HSRL TEC") -> (w529:T6)
                                n408 = call "TL_Driver_v2.vi"("Device In"=w523, "Commands"=T9."SET", "Settings"=w529) -> ("Readings"=w527:T7)  [unwired: 9 in, 3 out]
                                n409 = local write "Settings"(w529) -> ()
                                n410 = local write "Readings"(w527) -> ()
                                }
                                }
                                }
                              }
                              n411 = Or(x=w471, y="Cancel HSRL") -> (x .or. y?=w472:bool)
                            }
                          }
                        }
                      }
                    }
                  }
                  frame #1 {
                    # "Reading the power meter"
                    # "Updating the pulse energy plot"
                    # "Converting to pulse energy"
                    # "Reading the offline output power, converting to pulse energy,  and updating the Pulse energy plot"
                    n412 = local read "SampleSize"() -> (w532:i32)
                    n413 = local read "Newport Device Key"() -> (w533:string)
                    n414 = local read "Online Pulse Energy"() -> (w539:dbl)
                    n415 = local read "Offline Pulse Energy"() -> (w538:dbl)
                    n416 = local read "NewportRef"() -> (w530:refnum<k24>)
                    n417 = Number To Decimal String(number=w532) -> (decimal integer string=w534:string)  [unwired: 1 in]
                    n418 = invoke class="PowerMeterCommands" method="PerformDAQ"(reference=w530, "deviceKey"=w533, "interval"="1", "sampleSize"=w534) -> ("PerformDAQ"=w535:dbl[])  [unwired: 2 in, 5 out]
                    n419 = Bundle("Online Pulse Energy"=w539, "Offline Pulse Energy"=w538) -> (w537:T15)  [unwired: 1 in]
                    n420 = local write "Pulse Energy (Micro Joule)"(w537) -> ()
                    n421 = call-poly <vilib>:"Mean.vi"("X"=w535) -> ("mean"=w531:dbl)  [unwired: 1 out]
                    n422 = Multiply(x=w531, y=1000.0) -> (x*y=w544:dbl)
                    n423 = Divide(x=w544, y=0.05) -> (x/y=w542:dbl)
                    n424 = Divide(x=w542, y=7.0) -> (x/y=→"Offline Pulse Energy":dbl)
                  }
                  frame #2 {
                    # "Added in the ability to interactively control the ThorLab  setting (just etalon temp for now)"
                    # "Wait 'Scalar Wait Time' for buffers to clear of online contiminated offline data"
                    n425 = disable-structure shown="Disabled" {
                      frame Disabled {
                        # "Wait 'Scalar Wait Time'"
                        n426 = local read "Scalar Wait Time"() -> (w561:u32)
                        n427 = Wait (ms)(milliseconds to wait=w561) -> ()  [unwired: 1 out]
                      }
                      frame Enabled {
                      }
                    }
                    n428 = event shown="[2] \"Settings.HSRL Etalon TEC\": Value Change" {
                      selector: _ -> [_ _ _]
                      dyn-events: _ -> [_ _ _]
                      timeout: 1 -> [_ _ _]
                      event Timeout {
                        n429 = event-data() -> ()  [unwired: 1 in, 2 out]
                      }
                      event "Settings.WV Etalon TEC": Value Change {
                        # "Generating a command string\nto update the etalon"
                        n430 = event-data() -> ()  [unwired: 1 in, 5 out]
                        n431 = local read "Settings"() -> (w551:T6)
                        n432 = Unbundle By Name(w551) -> ("WV Etalon TEC"=w553:dbl)
                        n433 = local read "Device In"() -> (w547:refnum<visa-resource-name>)
                        n434 = Bundle By Name(cluster=w551, "WV Etalon TEC"=w553, "Module"=T12."WV Etalon TEC") -> (w549:T6)
                        n435 = call "TL_Driver_v2.vi"("Device In"=w547, "Commands"=T9."SET", "Settings"=w549) -> ("Readings"=w550:T7)  [unwired: 9 in, 3 out]
                        n436 = local write "Readings"(w550) -> ()
                        n437 = local write "Settings"(w549) -> ()
                      }
                      event "Settings.HSRL Etalon TEC": Value Change {
                        # "Generating a command string\nto update the etalon"
                        n438 = event-data() -> ()  [unwired: 1 in, 5 out]
                        n439 = local read "Settings"() -> (w558:T6)
                        n440 = Unbundle By Name(w558) -> ("HSRL Etalon TEC"=w560:dbl)
                        n441 = local read "Device In"() -> (w554:refnum<visa-resource-name>)
                        n442 = Bundle By Name(cluster=w558, "HSRL Etalon TEC"=w560, "Module"=T12."HSRL Etalon TEC") -> (w556:T6)
                        n443 = call "TL_Driver_v2.vi"("Device In"=w554, "Commands"=T9."SET", "Settings"=w556) -> ("Readings"=w557:T7)  [unwired: 9 in, 3 out]
                        n444 = local write "Readings"(w557) -> ()
                        n445 = local write "Settings"(w556) -> ()
                      }
                    }
                  }
                  frame #3 {
                    w590 = 1 ("dimension size")
                    # "Read in latest scalar card data from \n'Scalar Data' global variable that \nscaler.vi is writing to, then wait 1 sec\nfor next batch of data"
                    # "Calculating/Plotting smoothed data,\ncross sections etc."
                    # "Pick off data with\nout header"
                    # "Calculate mean bin by bin mean"
                    # "Reading in 'Integration Period (Seconds)' of data"
                    # "Read the offline data from the scalar card, perform smoothing, calculate normalized relative backscatter, and plot"
                    # "Collects Data From Card,\nSends It To The Chart,\nAnd Saves A Copy As A\nFile If Option Selected On\nFront Panel"
                    n446 = for {
                      N: "Data Reads (number of loops)" -> [_]
                      tunnel: [w648] -> w579 mode=indexing
                      tunnel: [w647] -> w578 mode=indexing
                      n447 = global read "AMCS_Data.vi" "AMCS_Data"() -> (w649:u16[][])
                      n448 = disable-structure shown="Disabled" {
                        frame Disabled {
                          n449 = global read "Scalar_Data_4.vi" "Scalar Data 4"() -> ()  [unwired: 1 out]
                          n450 = global read "Scalar_Data_2.vi" "Scalar Data 2"() -> ()  [unwired: 1 out]
                        }
                        frame Enabled {
                        }
                      }
                      n451 = Index Array(array=w649, index (row) #1=1 ("index (row)"), index (row) #2=3 ("index (row)")) -> (element #1=w648:u16[], element #2=w647:u16[])  [unwired: 2 in]
                    }
                    n452 = local read "Total DIAL Integration Time (Minutes)"() -> (w610:i32)
                    n453 = Divide(x=w610, y="Data Reads (number of loops)") -> (x/y=w608:dbl)
                    n454 = local read "Total Aerosol Integration Time (Minutes)"() -> (w612:dbl)
                    n455 = Multiply(x=w608, y=60.0) -> (x*y=w596:dbl)
                    n456 = local read "background length"() -> (w583:i32)
                    n457 = local read "background start"() -> (w584:u32)
                    n458 = Transpose 2D Array(2D array=w579) -> (transposed array=w618:u16[][])
                    n459 = Transpose 2D Array(2D array=w578) -> (transposed array=w602:u16[][])
                    n460 = Divide(x=w612, y="Data Reads (number of loops)") -> (x/y=w613:dbl)
                    n461 = for {
                      tunnel: w618 -> [w655] mode=indexing
                      tunnel: [w654] -> w619 mode=indexing
                      tunnel: w602 -> [w653] mode=indexing
                      tunnel: [w652] -> _ mode=indexing
                      tunnel: [w652] -> w599 mode=indexing
                      n462 = call-poly <vilib>:"Mean.vi"("X"=w655) -> ("mean"=w654:dbl)  [unwired: 1 out]
                      n463 = call-poly <vilib>:"Mean.vi"("X"=w653) -> ("mean"=w652:dbl)  [unwired: 1 out]
                    }
                    n464 = local read "bins"() -> (w591:u32)
                    n465 = Multiply(x=w613, y=60.0) -> (x*y=w575:dbl)
                    n466 = Array Subset(array=w599, index=w590, length=w591) -> (w600:dbl[])
                    "CH3 Bin Readings" <- w600
                    n467 = Array Subset(array=w619, index=w590, length=w591) -> (w598:dbl[])
                    "CH1  Bin Readings" <- w598
                    n468 = Array Subset(array=w600, index=w584, length=w583) -> (w601:dbl[])
                    n469 = Array Subset(array=w598, index=w584, length=w583) -> (w617:dbl[])
                    n470 = local read "Smoothed Bins"() -> (w580:dbl)
                    n471 = call-poly <vilib>:"Mean.vi"("X"=w601) -> ("mean"=w565:dbl)  [unwired: 1 out]
                    n472 = call-poly <vilib>:"Mean.vi"("X"=w617) -> ("mean"=w570:dbl)  [unwired: 1 out]
                    n473 = local read "Index"() -> (w576:i32)
                    n474 = Subtract(x=w600, y=w565) -> (x-y=w577:dbl[])
                    n475 = Subtract(x=w598, y=w570) -> (x-y=w594:dbl[])
                    n476 = call "Ring Buffer CH1 short rev2.vi"("Index"=w576, "Profiles to Average"=w596, "Input Array"=w594) -> ("AvgArray"=w615:dbl[], "RingBufferOut"=→"CH1 RingBuffer long":dbl[][])  [unwired: 7 in]
                    n477 = call "Ring Buffer CH1 long rev2.vi"("Index"=w576, "Profiles to Average"=w575, "Input Array"=w594) -> ("AvgArray"=w611:dbl[], "RingBufferOut"=→"CH1 RingBuffer short":dbl[][])  [unwired: 7 in]
                    n478 = call "Ring Buffer CH3 long rev2.vi"("Index"=w576, "Profiles to Average"=w596, "Input Array"=w577) -> ("AvgArray"=w597:dbl[], "RingBufferOut"=→"CH3 RingBuffer long":dbl[][])  [unwired: 7 in]
                    n479 = call "Ring Buffer CH3 short rev2.vi"("Index"=w576, "Profiles to Average"=w575, "Input Array"=w577) -> ("AvgArray"=w587:dbl[], "RingBufferOut"=→"CH3 RingBuffer short":dbl[][])  [unwired: 7 in]
                    n480 = Reshape Array(w594, w590, w591) -> (→"CH 1 (WV off) counts display":dbl[][])
                    n481 = Reshape Array(w577, w590, w591) -> (→"CH 3 (HSRL comb) counts display":dbl[][])
                    n482 = local read "Time Resolution Per Bin(ns)"() -> (w566:u32)
                    n483 = local read "Number of Accumulates"() -> (w564:u32)
                    n484 = call "Smooth Arrray.vi"("smooth size"=w580, "Raw Array"=w615) -> ("Smoothed Array"=→"CH1 (WV off) smooth S":dbl[])  [unwired: 9 in]
                    n485 = call "Smooth Arrray.vi"("smooth size"=w580, "Raw Array"=w611) -> ("Smoothed Array"=w589:dbl[])  [unwired: 9 in]
                    "CH1 (WV off) smooth L" <- w589
                    n486 = call "Smooth Arrray.vi"("smooth size"=w580, "Raw Array"=w597) -> ("Smoothed Array"=→"CH3 (HSRL combined) smooth L":dbl[])  [unwired: 9 in]
                    n487 = call "Smooth Arrray.vi"("smooth size"=w580, "Raw Array"=w587) -> ("Smoothed Array"=w582:dbl[])  [unwired: 9 in]
                    "CH3 (HSRL combined) smooth S" <- w582
                    n488 = local read "Temperature (C)"() -> (w607:dbl)
                    n489 = local read "Pressure (mb)"() -> (w606:dbl)
                    n490 = To Double Precision Float(number=w564) -> (double precision float=w563:dbl)
                    n491 = To Double Precision Float(number=w566) -> (double precision float=w562:dbl)
                    n492 = Reciprocal(x=w562) -> (1/x=w573:dbl)
                    n493 = disable-structure shown="Enabled" {
                      disable-tunnel: w607 -> [w646 _]
                      disable-tunnel: w606 -> [w645 _]
                      disable-tunnel: w589 -> [w639 _]
                      disable-tunnel: w570 -> [w626 _]
                      disable-tunnel: w565 -> [w625 _]
                      disable-tunnel: w563 -> [w624 _]
                      disable-tunnel: "dead time" -> [w623 _]
                      disable-tunnel: w582 -> [w622 _]
                      disable-tunnel: 6.0 ("Real") -> [w621 _]
                      disable-tunnel: w562 -> [w620 _]
                      frame Enabled {
                        w642 = 1
                        # "Plotting the normalized relative \nbackscatter"
                        # "Calculating the normalized relative backscatter"
                        # "File path in MATLAB script is of old dial is:\nF:\\Micropulse DIAL\\Micropulse DIAL Matlab\\\nFinal Overlap Function.mat')];"
                        n494 = script code="%accum_num=10000;     % scaler card setting number of accumulations\nt_bin = t_bin_in/1e9                 % scaler card setting time per bin\n%t_d = 37.3e-9;                % APD dead time from spec sheet\n\n% conversion from accumulated counts to count rate  (c/s)\nc_convert = 1./t_bin./accum_num;\nCR_far = p_raw_far.*c_convert;\nCR_near = p_raw_near.*c_convert;\nCR_total_far = (p_raw_far+b_far).*c_convert;\nCR_total_near = (p_raw_near+b_near).*c_convert;\nb_CR_far =b_far.*c_convert;\nb_CR_near =b_near.*c_convert;\n \n% create a range array\nsize_p =  size(p_raw_far,2);\ngate = t_bin*3e8/2;\nr = (gate:gate:size_p*gate)./1e3; \n   \n%APD correction factor\n D_far = 1./(1-(t_d*CR_total_far));\n D_near = 1./(1-(t_d*CR_total_near));\n\n %Calculating normalize relative backscatter profile\n nrb_far = CR_far.*D_far.*r.^2.*1e-6;\n nrb_near = CR_near.*D_near.*r.^2.*1e-6;"("E"=w621, "temp"=w646, "press"=w645, "p_raw_far"=w639, "b_far"=w626, "b_near"=w625, "p_raw_near"=w622, "accum_num"=w624, "t_d"=w623, "t_bin_in"=w620) -> ("nrb_far"=w634:cdb[], "D_far"=w631:dbl[], "nrb_near"=w633:cdb[], "D_near"=w630:dbl[])  [unwired: 1 in, 1 out]
                        n495 = local read "bins"() -> (w641:u32)
                        n496 = local read "Altitude Array (km)"() -> (w636:dbl[])
                        n497 = Build Array(w634, w633) -> (w638:cdb[][])
                        n498 = Build Array(w631, w630) -> (w629:dbl[][])
                        n499 = Reshape Array(w633, w642, w641) -> (→"NRB 2":cdb[][])
                        n500 = Reshape Array(w634, w642, w641) -> (→"NRB":cdb[][])
                        n501 = Build Array(w636, w636) -> (w635:dbl[][])
                        n502 = call "Convert to Dynamic Data7"("2D Array"=w629) -> ("Dynamic Data Type"=w628:dynamicdata)  [unwired: 3 in]
                        n503 = call "Convert to Dynamic Data3"("2D Array"=w638) -> ("Dynamic Data Type"=w637:dynamicdata)  [unwired: 3 in]
                        n504 = call "Convert to Dynamic Data4"("2D Array"=w635) -> ("Dynamic Data Type"=w632:dynamicdata)  [unwired: 3 in]
                        n505 = call "Build XY Graph2"("Y Input"=w632, "X Input"=w637) -> ("XY Graph"=→"NRB plot":cluster{"Y":dbl[], "Y":dbl[]}[])  [unwired: 3 in, 6 out]
                        n506 = call "Build XY Graph4"("Y Input"=w632, "X Input"=w628) -> ("XY Graph"=→"Correction":cluster{"Y":dbl[], "Y":dbl[]}[])  [unwired: 3 in, 6 out]
                      }
                      frame Disabled {
                      }
                    }
                    n507 = Divide(x=w573, y=w563) -> (x/y=w571:dbl)
                    n508 = Multiply(x=1000000000.0, y=w571) -> (x*y=w568:dbl)
                    n509 = Multiply(x=w568, y=w570) -> (x*y=w569:dbl)
                    n510 = Multiply(x=w568, y=w565) -> (x*y=w567:dbl)
                    n511 = Bundle(w569, w567) -> (→"?":cluster{dbl, dbl})  [unwired: 1 in]
                  }
                  frame #4 {
                    # "REPLACE WITH NEW AGILTRON TASK!"
                    # "Toggle Agiltron switch to online DBR"
                    n512 = disable-structure shown="Disabled" {
                      frame Disabled {
                        # "ABSORBING"
                        n513 = flat-sequence {
                          frame #0 {
                            # "Third one"
                            # "Command the switch to switch to position 1\ncorresponding to the online DBR"
                            # "Hex string command \ncorrespond to online"
                            n514 = local read "Switch Comm Port"() -> (w659:refnum<visa-resource-name>)
                            n515 = VISA Write(VISA resource name=w659, write buffer="\u0001\u0012\u0000\u0002") -> ()  [unwired: 1 in, 3 out]
                          }
                        }
                        n516 = Build Array(FALSE ("Boolean")) -> (w658:bool[])
                        n517 = call-poly <vilib>:"DAQmx Write.vi"("task/channels in"=refnum<k21> "AgiltronSwitch", "data"=w658) -> ()  [unwired: 11 in, 3 out]
                      }
                      frame Enabled {
                      }
                    }
                  }
                  frame #5 {
                    # "If 'Save Data?' is true, save all relavant offline info"
                    n518 = local read "Save Data?"() -> (w661:bool)
                    n519 = case shown="True" w661 {
                      frame False {
                        # "'Save Data?' is false, do nothing"
                      }
                      frame True {
                        # "Write only one data file at this time"
                        # "Retrive Julian Date"
                        # "'Save Data?' is true, save offline data to the Data Disk"
                        n520 = local read "Readings"() -> (w662:T7)
                        n521 = Unbundle By Name(w662) -> ("WV Offline TEC"=w663:dbl)
                        n522 = Unbundle By Name(w662) -> ("HSRL TEC"=w664:dbl)
                        n523 = local read "HSRL Read (nm)"() -> (w665:dbl)
                        n524 = local read "WV Offline Read (nm)"() -> (w686:dbl)
                        n525 = local read "Relative Humdity (%)"() -> (w690:dbl)
                        n526 = local read "CH3 Bin Readings"() -> (w684:dbl[])
                        n527 = local read "CH1  Bin Readings"() -> (w691:dbl[])
                        n528 = local read "Offline Pulse Energy"() -> (w687:dbl)
                        n529 = local read "Temperature (C)"() -> (w688:dbl)
                        n530 = local read "Pressure (mb)"() -> (w689:dbl)
                        n531 = call "Julian_Date_2.vi"() -> ("Julian Date"=w685:dbl)  [unwired: 11 in]
                        n532 = Build Array (concatenate)(w685, w686, w663, w687, w688, w689, w690, w691) -> (w670:dbl[])
                        n533 = Build Array (concatenate)(w685, w665, w664, w687, w688, w689, w690, w684) -> (w667:dbl[])
                        n534 = local read "FF_Off_Ref"() -> (w672:refnum<file>)
                        n535 = local read "NF_Off_Ref"() -> (w669:refnum<file>)
                        n536 = local read "FF_Off_Ptr"() -> (w671:i64)
                        n537 = local read "NF_Off_Ptr"() -> (w668:i64)
                        n538 = Set File Position(offset (in bytes) (0)=w671, refnum=w672) -> (refnum out=w683:refnum<file>, error out=w681:errorcluster)  [unwired: 2 in]
                        n539 = Set File Position(offset (in bytes) (0)=w668, refnum=w669) -> (refnum out=w679:refnum<file>, error out=w677:errorcluster)  [unwired: 2 in]
                        n540 = Write to Binary File(file (use dialog)=w683, data=w670, error in=w681, 5:FALSE ("prepend array or string size? (T)")) -> (refnum out=w682:refnum<file>, error out=w680:errorcluster)  [unwired: 2 in, 1 out]
                        n541 = Write to Binary File(file (use dialog)=w679, data=w667, error in=w677, 5:FALSE ("prepend array or string size? (T)")) -> (refnum out=w678:refnum<file>, error out=w676:errorcluster)  [unwired: 2 in, 1 out]
                        n542 = Get File Position(4:w680, 7:w682) -> (2:w673:i64)  [unwired: 2 out]
                        n543 = Get File Position(4:w676, 7:w678) -> (2:w666:i64)  [unwired: 2 out]
                        n544 = local write "FF_Off_Ptr"(w673) -> ()
                        n545 = local write "NF_Off_Ptr"(w666) -> ()
                      }
                    }
                  }
                }
              }
              frame #4 {
                n546 = First Call?() -> (First Call?: T/F=w694:bool)
                n547 = Or(x="calculate absorption cross sections", y=w694) -> (x .or. y?=w692:bool)
                n548 = case shown="True" w692 {
                  frame False {
                  }
                  frame True {
                    # "calculate absorption cross sections from HITRAN data base"
                    n549 = local read "WV Offline Set (nm)"() -> (w697:dbl)
                    n550 = local read "CH1 (WV off) smooth S"() -> (w701:dbl[])
                    n551 = local read "WV Online Read (nm)"() -> (w700:dbl)
                    n552 = local read "Temperature (C)"() -> (w699:dbl)
                    n553 = local read "Pressure (mb)"() -> (w698:dbl)
                    n554 = script code="hitran = dlmread('C:\\Users\\H2ODial\\Desktop\\Shared Telescope WV DIAL Code\\Libraries and VIs\\815nm_841nm_HITRAN_2008.csv', ',',[1 1 1676 8]);\n%hitran = dlmread('C:\\Users\\H2ODial\\Desktop\\Shared Telescope WV DIAL Code\\Libraries and VIs\\824nm_841nm_H2O.csv', ',',[0 1 352 7]);\n%hitran = dlmread('C:\\Users\\H2ODial\\Desktop\\Shared Telescope WV DIAL Code\\Libraries and VIs\\824nm_841nm_H2O_Spectral_Calc.csv', ',',[1 1 1209 7]);\n\n%Range vector in meters\nrange = ([75:75:size(Online,2)*75]);\n\nif lambda< 828\nlambda=828.195;\nelse\nlambda=lambda;\nend;\n\n%%\n\n%Voigt profile calculation\nWNmin = 1/(828+4)*1e7;  % 832.0 nm converted to wavenumber\nWNmax = 1/(828-4)*1e7;  % 824.0 nm converted to wavenumber\n\n%Find lines from WNmin to WNmax to calculate voigt profile\nline_indices = hitran(1:size(hitran,1),1)>WNmin & hitran(1:size(hitran,1),1)<WNmax;\n\nline = double(hitran(line_indices, 1:size(hitran,2)));\n\n%Calculate temperature and pressure profile\nT0 = 273+25; % surface temperature\nT0 = 273+T0_C;\nT = T0-0.0065.*range; % set to match the sounding\n\n% pressure in atmospheres\nP0  = 0.83; % surface pressure\nP0  = P0_mb/1000*0.986; %pressure in mb converted to atm\nP = P0.*(T0./T).^-5.5;   % set this value to match sounding\n\nT00 = 296;              % HITRAN reference temperature [K]\nP00 = 1;                % HITRAN reference pressure [atm]\nnu0_0 = line(:,1);      % absorption line center wavenumber from HITRAN [cm^-1]\nS0 = line(:,2);         % initial linestrength from HITRAN [cm^-1/(mol*cm^-2)]   \ngammal0 = line(:,4);    % air-broadened halfwidth at T_ref and P_ref from HITRAN [cm^-1/atm]\ngamma_s = line(:,5);    % self-broadened halfwidth at T_ref and P_ref from HITRAN [cm^-1/atm]\nE = line(:,6);          % ground state transition energy from HITRAN [cm^-1]  \nalpha = line(:,7);      % linewidth temperature dependence factor from HITRAN\ndelta = line(:,8);      % pressure shift from HiTRAN [cm^-1 atm^-1]\n\nnu_on = 1/(lambda)*1e7;\nnu_off = 1/(lambda_off)*1e7;\n\nfor i = 1:size(Online,2); % calculate the absorption cross section at each range\n  \n    nu0 = nu0_0+delta.*(P(i)./P00); % unclear if it should be Pi/P00  \n    gammal = gammal0.*(P(i)./P00).*((T00./T(i)).^alpha);    %Calculate Lorentz lineweidth at P(i) and T(i)\n\n    const.m = 18.015E-3./6.022E23; % mass of a single water molecule\n    const.k_B = 1.3806488e-23; % (J/K)\n    const.c = 299792458; % (m/s) (exact)\n \n    gammad = (nu0).*((2.0.*const.k_B.*T(i).*log(2.0))./(const.m.*const.c^2)).^(0.5);  %Calculate HWHM Doppler linewidth at T(i)\n     \n    % term 1 in the Voigt profile\n    y = (gammal./gammad).*((log(2.0)).^(0.5));\n    \n    % term 2 in the Voigt profile\n    x_on = ((nu_on-nu0)./gammad).*(log(2.0)).^(0.5);\n    x_off = ((nu_off-nu0)./gammad).*(log(2.0)).^(0.5);\n    \n    %setting up Voigt convolution\n    t = (-(size(line,1))/2:1:size(line,1)/2-1); %set up the integration spectral step size\n    t = repmat(t',1,length(x_on))';\n    x_on = repmat(x_on,1,length(t));\n    x_off = repmat(x_off,1,length(t));\n    y = repmat(y,1,length(t));\n    f_on = (exp(-t.^2.0))./(y.^2.0+(x_on-t).^2.0);  % combined Voigt term 1 and 2\n    f_off = (exp(-t.^2.0))./(y.^2.0+(x_off-t).^2.0);\n    %Voigt integration over all of the lines at the on and offline locations\n    z_on = trapz(t(1,:),f_on,2);\n    z_off =  trapz(t(1,:),f_off,2);\n    integral_on = z_on;\n    integral_off = z_off;\n    %Calculate linestrength at temperature T\n    S = S0.*((T00./T(i)).^(1.5)).*exp(1.439.*E.*((1./T00)-(1./T(i))));\n \n    %Calculate the Voigt profile\n    K_on = (y(:,1)./pi).*integral_on;\n    K_off = (y(:,1)./pi).*integral_off;\n    \n    %Calculate the Voigt profile absorption cross section [cm^2]\n    sigmav_on = S.*(1./gammad).*(((log(2.0))./pi).^(0.5)).*K_on; %.*far_wing_on;\n    sigmav_off = S.*(1./gammad).*(((log(2.0))./pi).^(0.5)).*K_off; %.*far_wing_off;\n    \n    %Sum contributions from all of the surrounding lines\n    sigma_on_total(i) = sum(sigmav_on);\n    sigma_off_total(i) = sum(sigmav_off);\n    \nend;"("lambda"=w700, "lambda_off"=w697, "P0_mb"=w698, "T0_C"=w699, "Online"=w701) -> ("sigma_on_total"=→"sigma_on_total":dbl[], "sigma_off_total"=→"sigma_off_total":dbl[])  [unwired: 1 in, 1 out]
                  }
                }
              }
              frame #5 {
                # "normalization factor\nfrom 300 to 450m"
                # "OPTICAL DEPTH PLOT"
                # "Data Processing Far Channel"
                # "Calculating the range resolved water vapor number density and plotting"
                n555 = local read "CH3 (HSRL combined) smooth L"() -> (w731:dbl[])
                n556 = local read "CH2 (molecular) smoothed"() -> (w730:dbl[])
                n557 = local read "CH0 (WV on) smoothed"() -> (w710:dbl[])
                n558 = local read "CH1 (WV off) smooth S"() -> (w709:dbl[])
                n559 = local read "sigma_on_total"() -> (w732:dbl[])
                n560 = local read "sigma_off_total"() -> (w733:dbl[])
                n561 = script code="%Time averaging in seconds.  600 Seconds =10 minutes\ntemporal_average = 600;\n\n%Spatial averaging in bins.  2 bins = 150 meters\nspatial_average = 2;\n\n%Creating r and r+deltar vectors..this can also be acsomplished using the\n%diff command\np_oni = Online(:,1:size(Online,2)-1);\n\np_onii = Online(:,2:size(Online,2));\n\np_offi = Offline(:,1:size(Offline,2)-1);\n\np_offii = Offline(:,2:size(Offline,2));\n\nInside = (p_oni.*p_offii)./(p_onii.*p_offi);\n\ndel_cross = 1./(2.*(sigma_on_total(1:size(Online,2)-1)-sigma_off_total(1:size(Offline,2)-1)).*75*100);\n\ndel_cross(isinf(del_cross)) = 0;\n\n%Calculating Number density\nN = del_cross.*log(Inside);\n\n%Spatial smoothing of the profiles\nfilter1 = ones(1,2)./2;\n\nN_1 = N;\n\nN_1_avg = filter2(filter1,N_1);\n\nfilter1 = ones(1,10)./10;\n\nN_2 = N;\n\nN_2_avg = filter2(filter1,N_2);\n\nN_new = zeros(size(N,1),size(N,2));\n \n%Using different averaging windows for different altitudes \nN_avg=[N_1_avg(:,1:40)';N_2_avg(:,41:size(N,2))']';\n\n\nw = N_avg.*1e6.*18.015./6.022e23"("Online"=w730, "Offline"=w731, "sigma_on_total"=w732, "sigma_off_total"=w733) -> ()  [unwired: 1 in, 3 out]
                n562 = script code="%Time averaging in seconds.  600 Seconds =10 minutes\ntemporal_average = 600;\n\n%Spatial averaging in bins.  2 bins = 150 meters\nspatial_average = 2;\n\n%Creating r and r+deltar vectors..this can also be acsomplished using the\n%diff command\np_oni = Online(:,1:size(Online,2)-1);\n\np_onii = Online(:,2:size(Online,2));\n\np_offi = Offline(:,1:size(Offline,2)-1);\n\np_offii = Offline(:,2:size(Offline,2));\n\nInside = (p_oni.*p_offii)./(p_onii.*p_offi);\n\ndel_cross = 1./(2.*(sigma_on_total(1:size(Online,2)-1)-sigma_off_total(1:size(Offline,2)-1)).*75*100);\n\ndel_cross(isinf(del_cross)) = 0;\n\n%Calculating Number density\nN = del_cross.*log(Inside);\n\n%Spatial smoothing of the profiles\nfilter1 = ones(1,2)./2;\n\nN_1 = N;\n\nN_1_avg = filter2(filter1,N_1);\n\nfilter1 = ones(1,10)./10;\n\nN_2 = N;\n\nN_2_avg = filter2(filter1,N_2);\n\nN_new = zeros(size(N,1),size(N,2));\n \n%Using different averaging windows for different altitudes \nN_avg=[N_1_avg(:,1:40)';N_2_avg(:,41:size(N,2))']';\n\n\nw = N_avg.*1e6.*18.015./6.022e23"("Online"=w710, "Offline"=w709, "sigma_on_total"=w732, "sigma_off_total"=w733) -> ()  [unwired: 1 in, 3 out]
                n563 = local read "Time Resolution Per Bin(ns)"() -> (w708:u32)
                n564 = To Double Precision Float(number=w708) -> (double precision float=w729:dbl)
                n565 = Multiply(x=0.15, y=w729) -> (x*y=w727:dbl)
                n566 = local read "Altitude Array (km)"() -> (w704:dbl[])
                n567 = Divide(x=300.0, y=w727) -> (x/y=w724:dbl)
                n568 = Divide(x=450.0, y=w727) -> (x/y=w723:dbl)
                n569 = To Long Integer(number=w724) -> (32bit integer=w722:i32)
                n570 = To Long Integer(number=w723) -> (32bit integer=w721:i32)
                n571 = Decrement(x=w722) -> (x-1=w719:i32)
                n572 = Decrement(x=w721) -> (x-1=w720:i32)
                n573 = Array Subset(array=w710, index=w719, length=w720) -> (w718:dbl[])
                n574 = Array Subset(array=w709, index=w719, length=w720) -> (w717:dbl[])
                n575 = call-poly <vilib>:"Mean.vi"("X"=w718) -> ("mean"=w716:dbl)  [unwired: 1 out]
                n576 = call-poly <vilib>:"Mean.vi"("X"=w717) -> ("mean"=w715:dbl)  [unwired: 1 out]
                n577 = Divide(x=w716, y=w715) -> (x/y=w714:dbl)
                n578 = Multiply(x=w709, y=w714) -> (x*y=w713:dbl[])
                n579 = Divide(x=w710, y=w713) -> (x/y=w712:dbl[])
                n580 = Natural Logarithm(1:w712) -> (0:w711:dbl[])
                n581 = Multiply(x=-1.0, y=w711) -> (x*y=w705:dbl[])
                n582 = call "Convert to Dynamic Data"("Array"=w705) -> ("Dynamic Data Type"=w707:dynamicdata)  [unwired: 3 in]
                n583 = call "Convert to Dynamic Data2"("Array"=w704) -> ("Dynamic Data Type"=w703:dynamicdata)  [unwired: 3 in]
                n584 = call "Build OD Plot"("Y Input"=w703, "X Input"=w707) -> ("XY Graph"=→"Optical Depth":cluster{"Y":dbl[], "Y":dbl[]}[])  [unwired: 3 in, 6 out]
              }
            }
          }
        }
        "L_Count" <- w129
      }
    }
  }
  n585 = case shown="True" w3 {
    frame False {
    }
    frame True {
      # "close data files"
      n586 = local read "NF_Off_Ref"() -> (w735:refnum<file>)
      n587 = local read "NF_On_Ref"() -> (w736:refnum<file>)
      n588 = local read "FF_Off_Ref"() -> (w737:refnum<file>)
      n589 = local read "FF_On_Ref"() -> (w738:refnum<file>)
      n590 = local read "WS_On/Off"() -> (w734:bool)
      n591 = case shown="True" w734 {
        frame False {
        }
        frame True {
          n592 = local read "WS visa"() -> (w739:refnum<visa-resource-name>)
          n593 = call "T_RH_P.vi"("VISA in"=w739, "WS_Commands"=enum16{"OpenWS", "ReadTRHP", "CloseWS"}."CloseWS") -> ()  [unwired: 11 in, 3 out]
        }
      }
      n594 = Close File(refnum=w738) -> ()  [unwired: 1 in, 2 out]
      n595 = Close File(refnum=w737) -> ()  [unwired: 1 in, 2 out]
      n596 = Close File(refnum=w736) -> ()  [unwired: 1 in, 2 out]
      n597 = Close File(refnum=w735) -> ()  [unwired: 1 in, 2 out]
    }
  }
  "FileHour" <- -1 ("FileHour")
  "DataOpen" <- FALSE
